vi "SSL Detection Frame Simple Estimator Cameras VelCmd.vi"(0 "Side":enum16{"Esquerdo", "Direito"}(ring)=enum."Direito" caption="Enum", 1 "cameras array":dbl[](array[numeric]), 4 "max ball vel":dbl, 5 "Estimador":T5=enum."Nenhum", 6 "Team":enum16{"Azul", "Amarelo"}(ring) caption="Enum", 8 "Fps":dbl=40.0, 9 "grSim?":bool, 10 "Field Size":T6, 11 "NewCameras":T1[](array[typedef]) {"robots_blue"."height" format="%+4.3f"; "robots_blue"."pixel_y" format="%+4.3f"; "robots_blue"."pixel_x" format="%+4.3f"; "robots_blue"."orientation" format="%+4.3f"; "robots_blue"."y" format="%+4.3f"; "robots_blue"."confidence" format="%4.3f"; "robots_blue"."x" format="%+4.3f"; "robots_yellow"."height" format="%+4.3f"; "robots_yellow"."pixel_y" format="%+4.3f"; "robots_yellow"."pixel_x" format="%+4.3f"; "robots_yellow"."orientation" format="%+4.3f"; "robots_yellow"."y" format="%+4.3f"; "robots_yellow"."confidence" format="%4.3f"; "robots_yellow"."x" format="%+4.3f"}) -> (2 "Field Size Out":T6, 3 "Detection Frame Out":T1 {"robots_blue"."height" format="%+4.3f"; "robots_blue"."pixel_y" format="%+4.3f"; "robots_blue"."pixel_x" format="%+4.3f"; "robots_blue"."orientation" format="%+4.3f"; "robots_blue"."y" format="%+4.3f"; "robots_blue"."confidence" format="%4.3f"; "robots_blue"."x" format="%+4.3f"; "robots_yellow"."height" format="%+4.3f"; "robots_yellow"."pixel_y" format="%+4.3f"; "robots_yellow"."pixel_x" format="%+4.3f"; "robots_yellow"."orientation" format="%+4.3f"; "robots_yellow"."y" format="%+4.3f"; "robots_yellow"."confidence" format="%4.3f"; "robots_yellow"."x" format="%+4.3f"})   [LabVIEW 2020]
uses:
  Controls/SSL Detection Frame.ctl
  Controls/SSL Detection Robot.ctl
  <vilib>/Analysis/Matrix/Datatypes/RealMatrix.ctl
  Controls/SSL Detection Ball.ctl
  Controls/Estimadores.ctl
  <vilib>/Analysis/Matrix/Numeric/Conversions/Array To Matrix - RA.vi
  <vilib>/Analysis/Matrix/NI_Matrix.lvlib
  <vilib>/ptbypt/NI_PtbyPt.lvlib
  Utilities_class/Utilities.lvclass
panel:
  in  "Enable":bool=TRUE
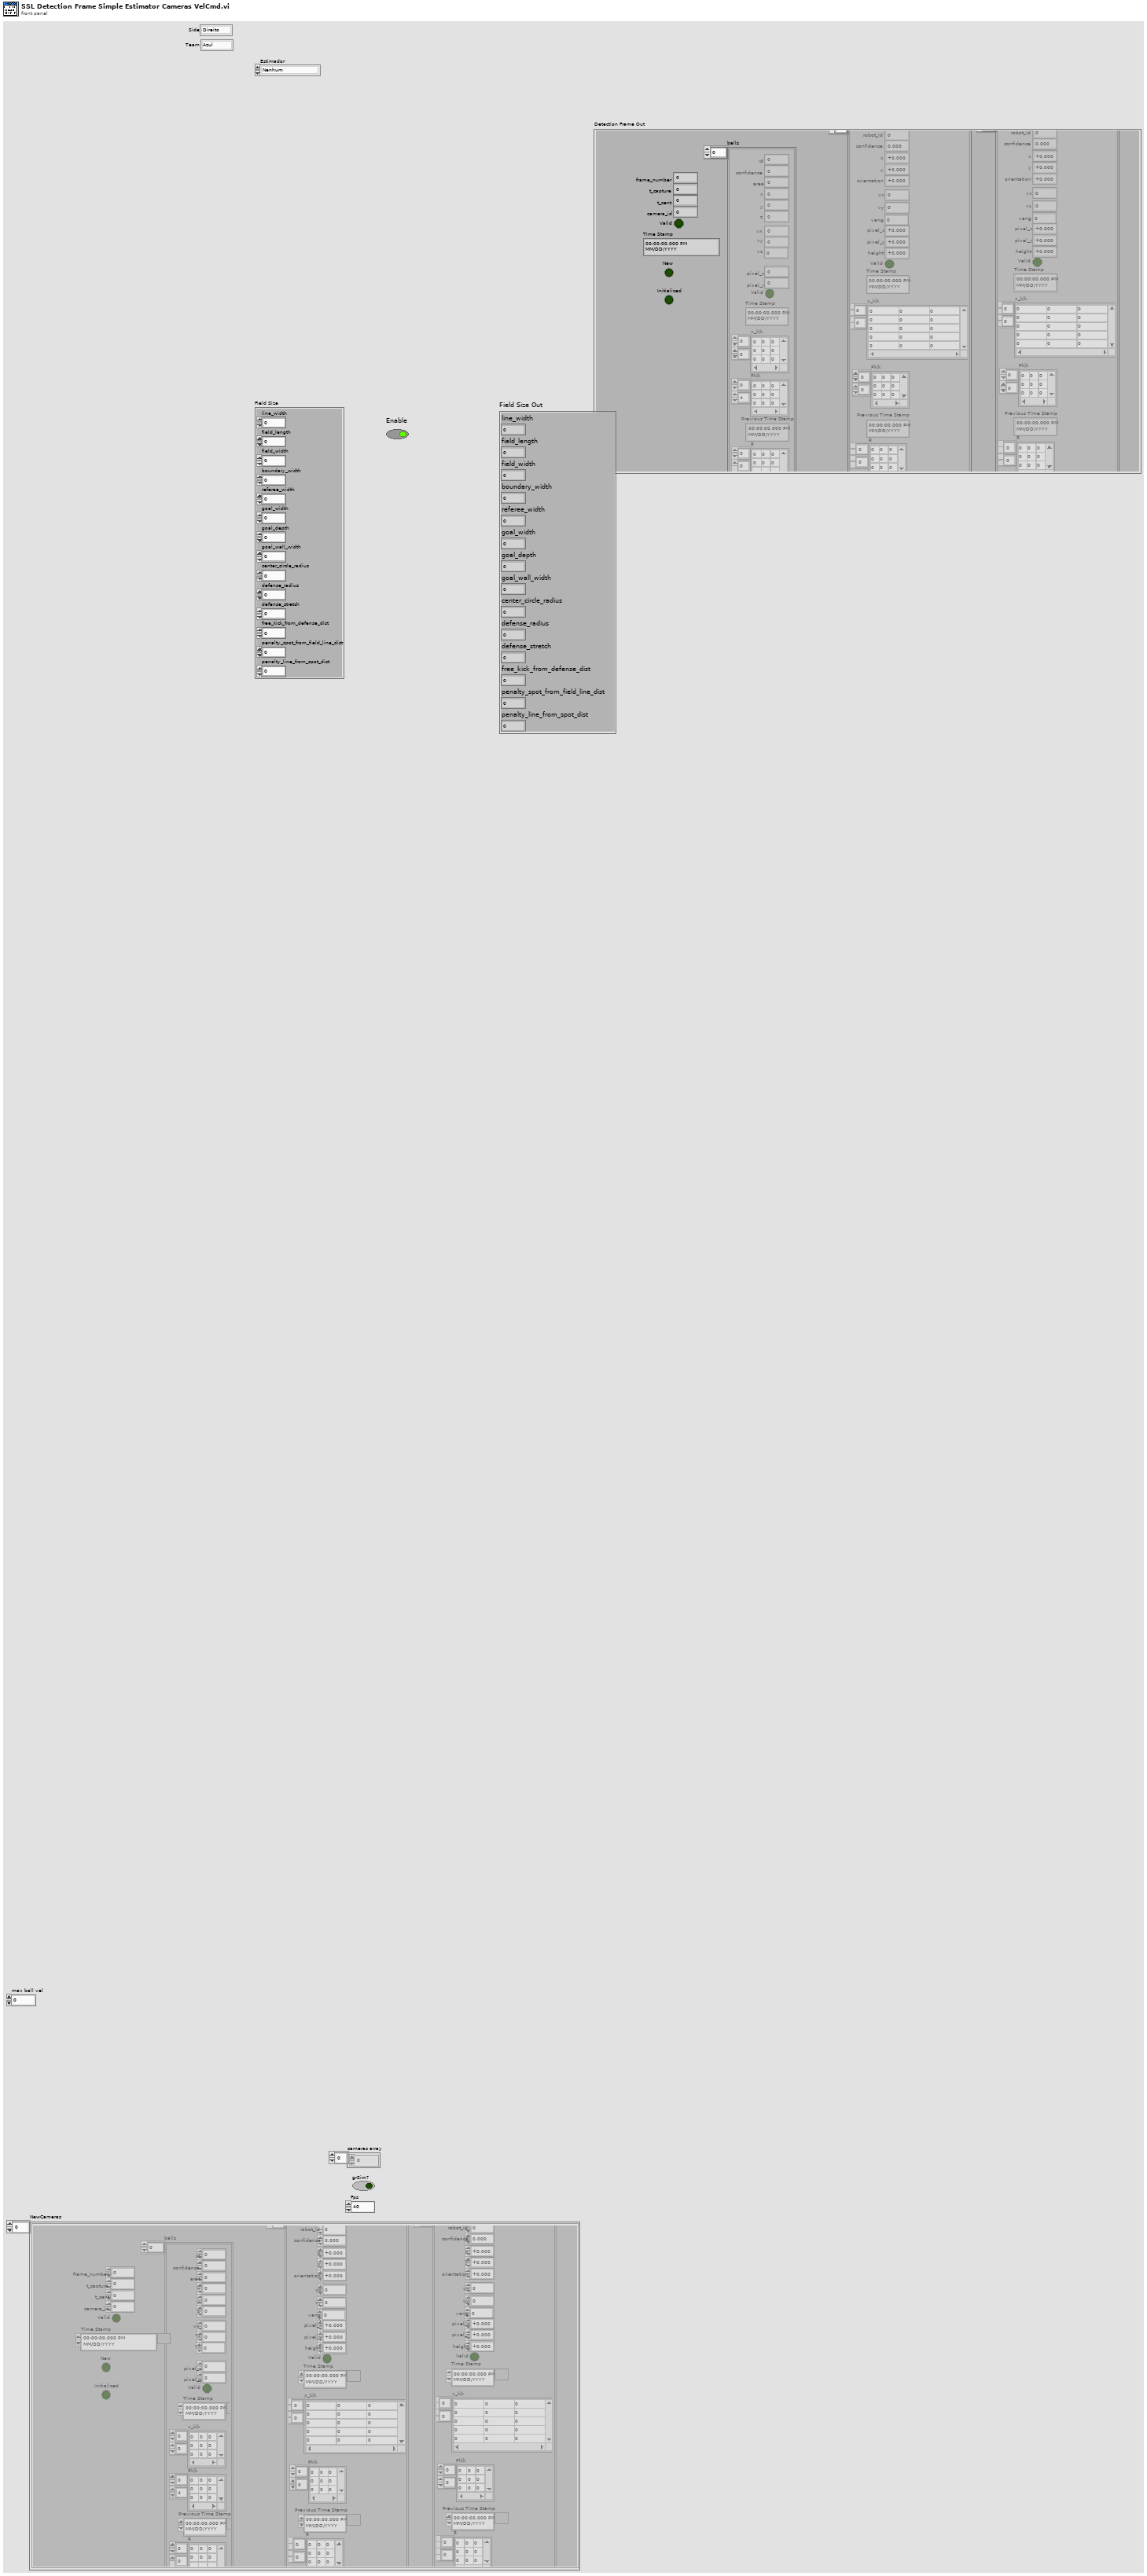
[diagram p1: front panel]
types:
  T1 = typedef "SSL Detection Frame.ctl" = cluster{"frame_number":u32, "t_capture":dbl, "t_sent":dbl, "camera_id":u32, "robots_yellow":T2[], "robots_blue":T2[], "balls":T4[], "Valid":bool, "Time Stamp":timestamp, "New":bool, "Initialized":bool}
  T2 = typedef "SSL Detection Robot.ctl" = cluster{"x":sgl, "robot_id":u32, "confidence":sgl, "y":sgl, "orientation":sgl, "pixel_x":sgl, "pixel_y":sgl, "height":sgl, "Valid":bool, "Time Stamp":timestamp, "x_k|k":T3, "Pk|k":T3, "Previous Time Stamp":timestamp, "R":T3, "vx":dbl, "vy":dbl, "vang":dbl}
  T3 = typedef "NI_Matrix.lvlib/RealMatrix.ctl" = dbl[][]
  T4 = typedef "SSL Detection Ball.ctl" = cluster{"x":sgl, "area":u32, "confidence":sgl, "y":sgl, "z":sgl, "pixel_x":sgl, "pixel_y":sgl, "Valid":bool, "Time Stamp":timestamp, "x_k|k":T3, "Pk|k":T3, "Id":u32, "Previous Time Stamp":timestamp, "R":T3, " vx":sgl, "vy":dbl, "vz":dbl}
  T5 = typedef "Estimadores.ctl" = enum16{"Variable2ndDerivate", "4thDerivate", "2ndDerivate", "Nenhum", "Simples", "Kalman"}
  T6 = cluster{"line_width":u32, "field_length":u32, "field_width":u32, "boundary_width":u32, "referee_width":u32, "goal_width":u32, "goal_depth":u32, "goal_wall_width":u32, "center_circle_radius":u32, "defense_radius":u32, "defense_stretch":u32, "free_kick_from_defense_dist":u32, "penalty_spot_from_field_line_dist":u32, "penalty_line_from_spot_dist":u32}
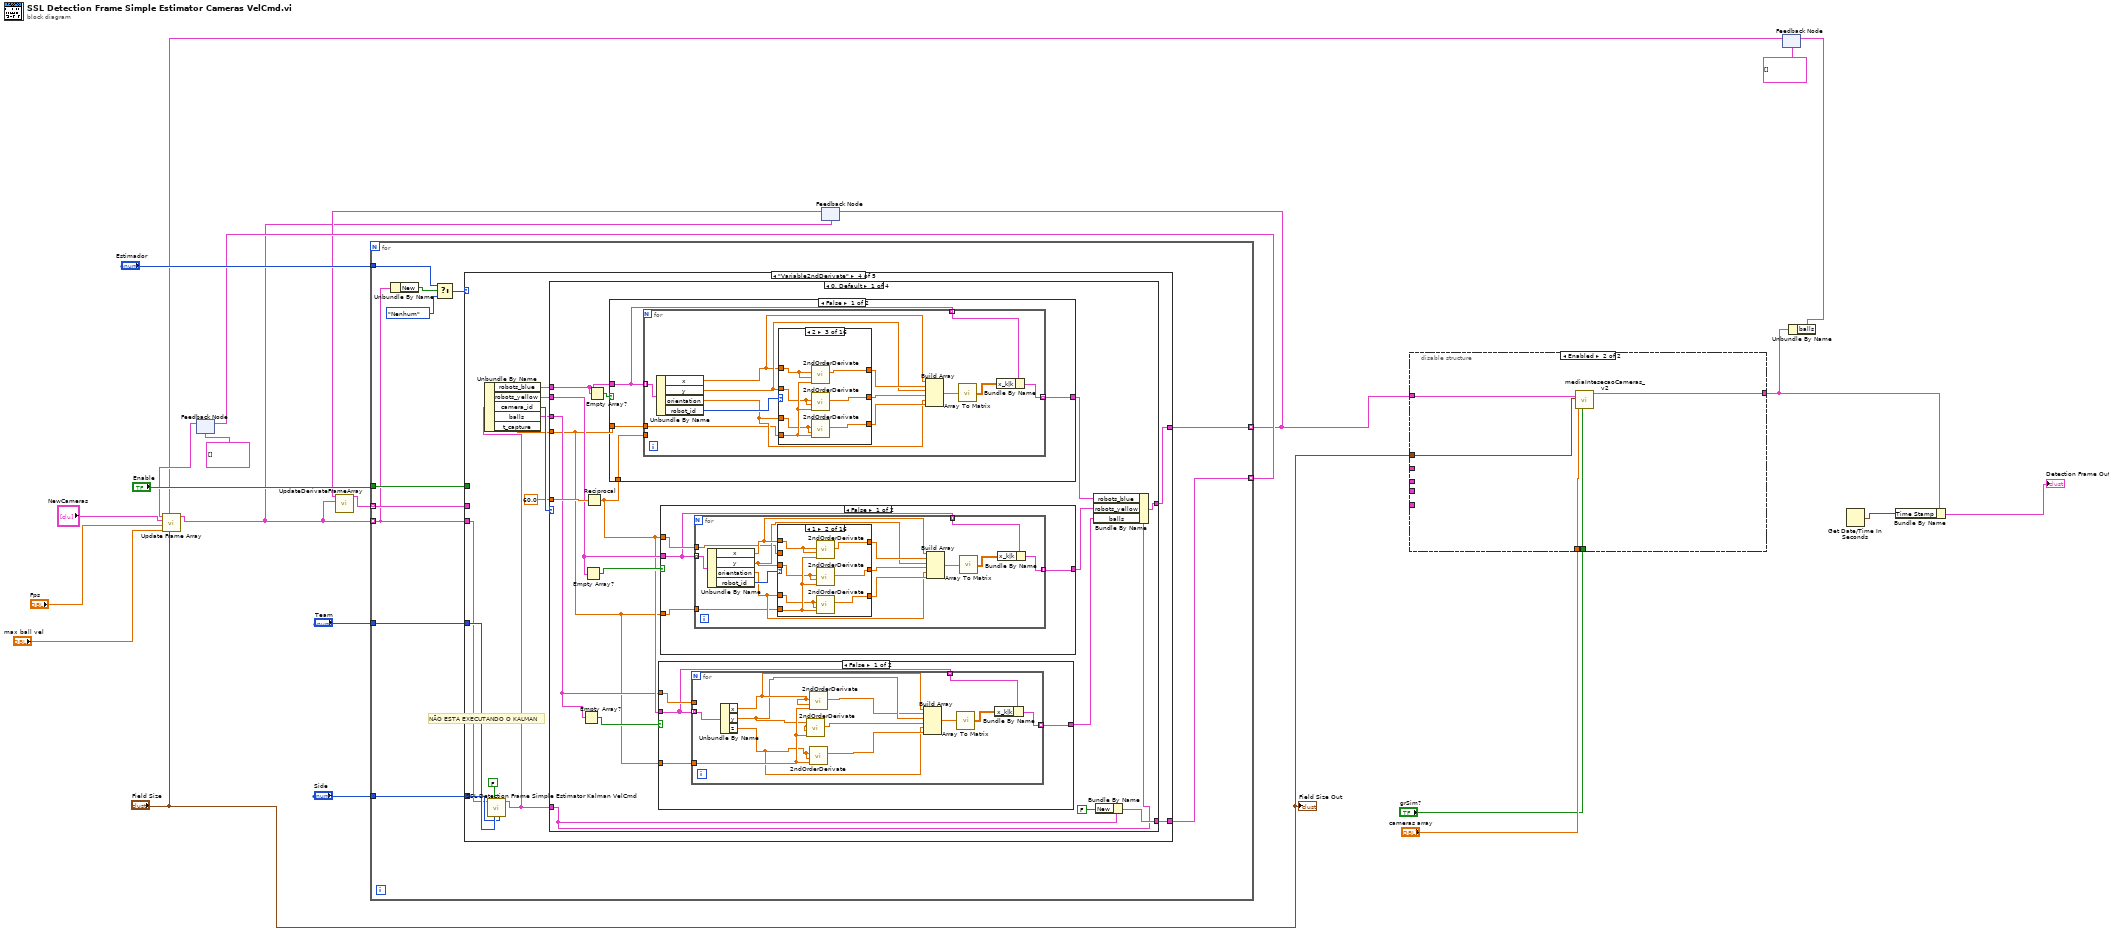
[diagram p0: block diagram]
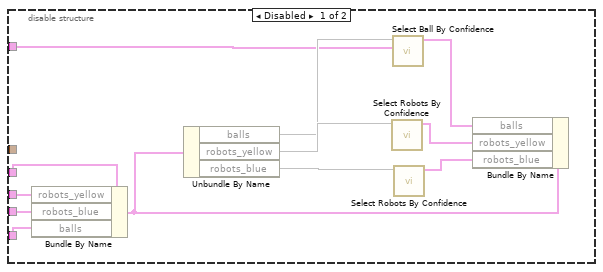
[diagram p2: hidden frame]
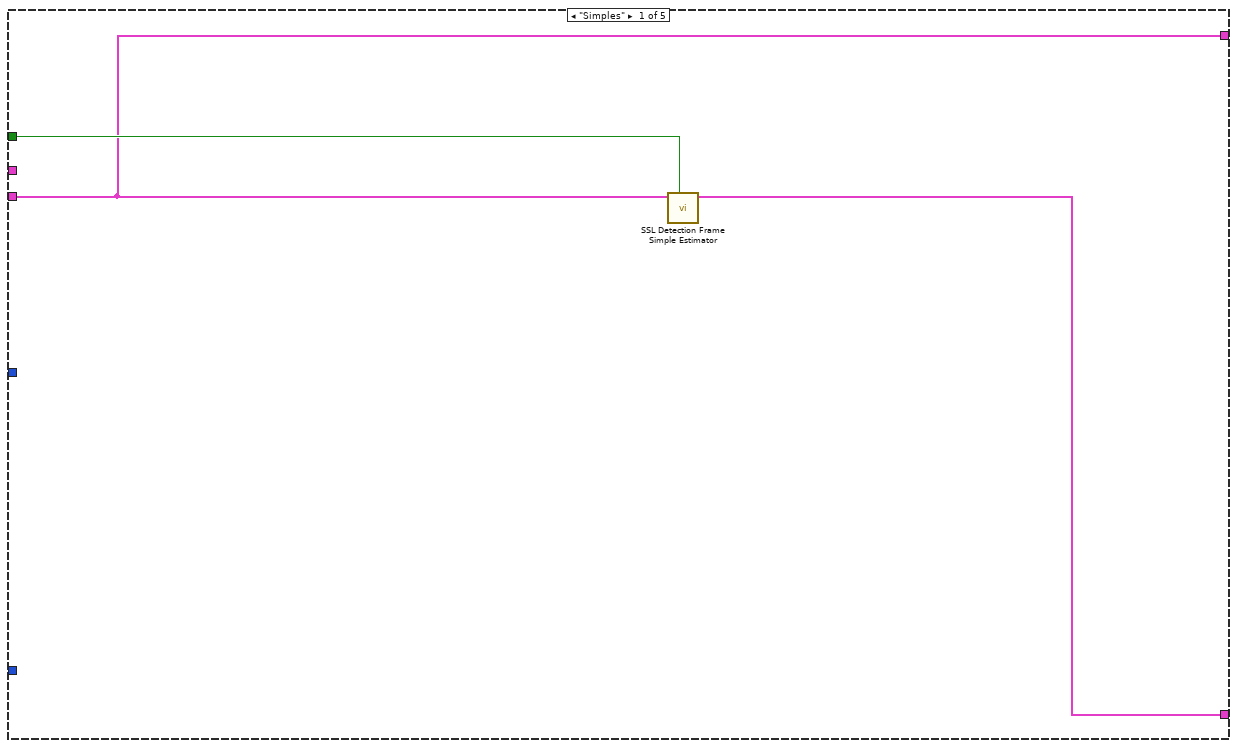
[diagram p3: hidden frame]
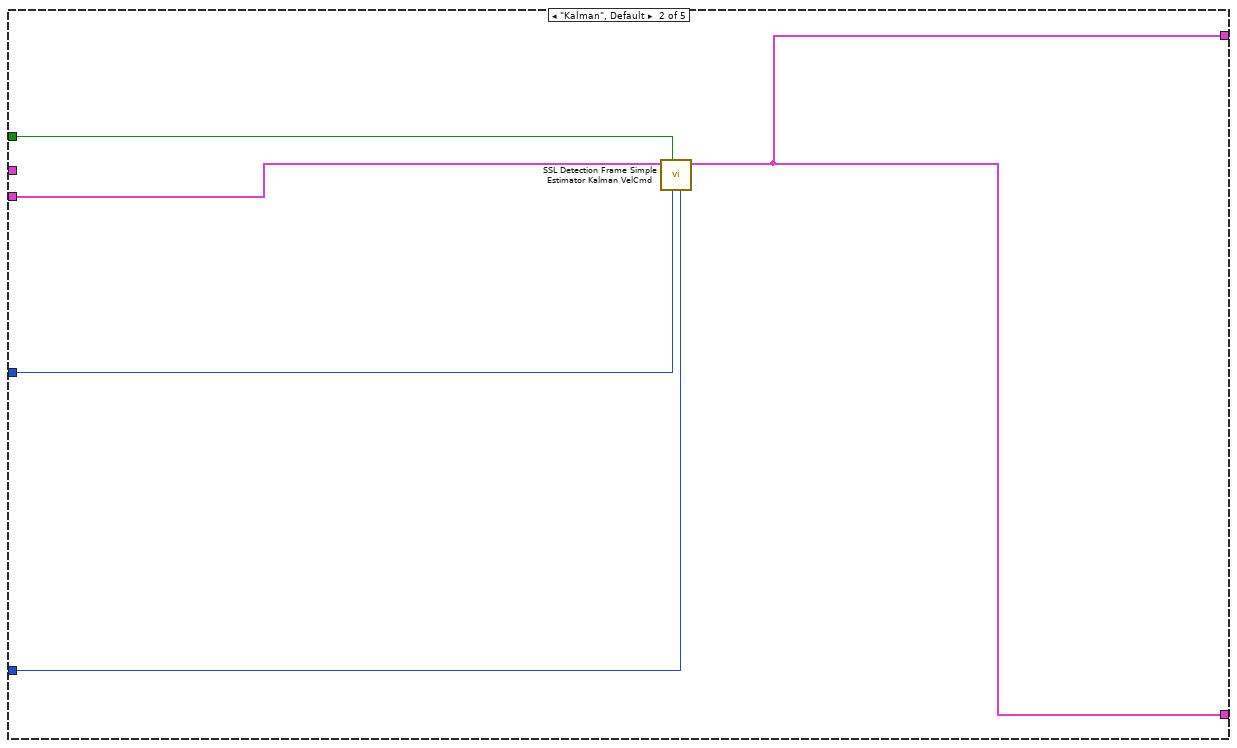
[diagram p4: hidden frame]
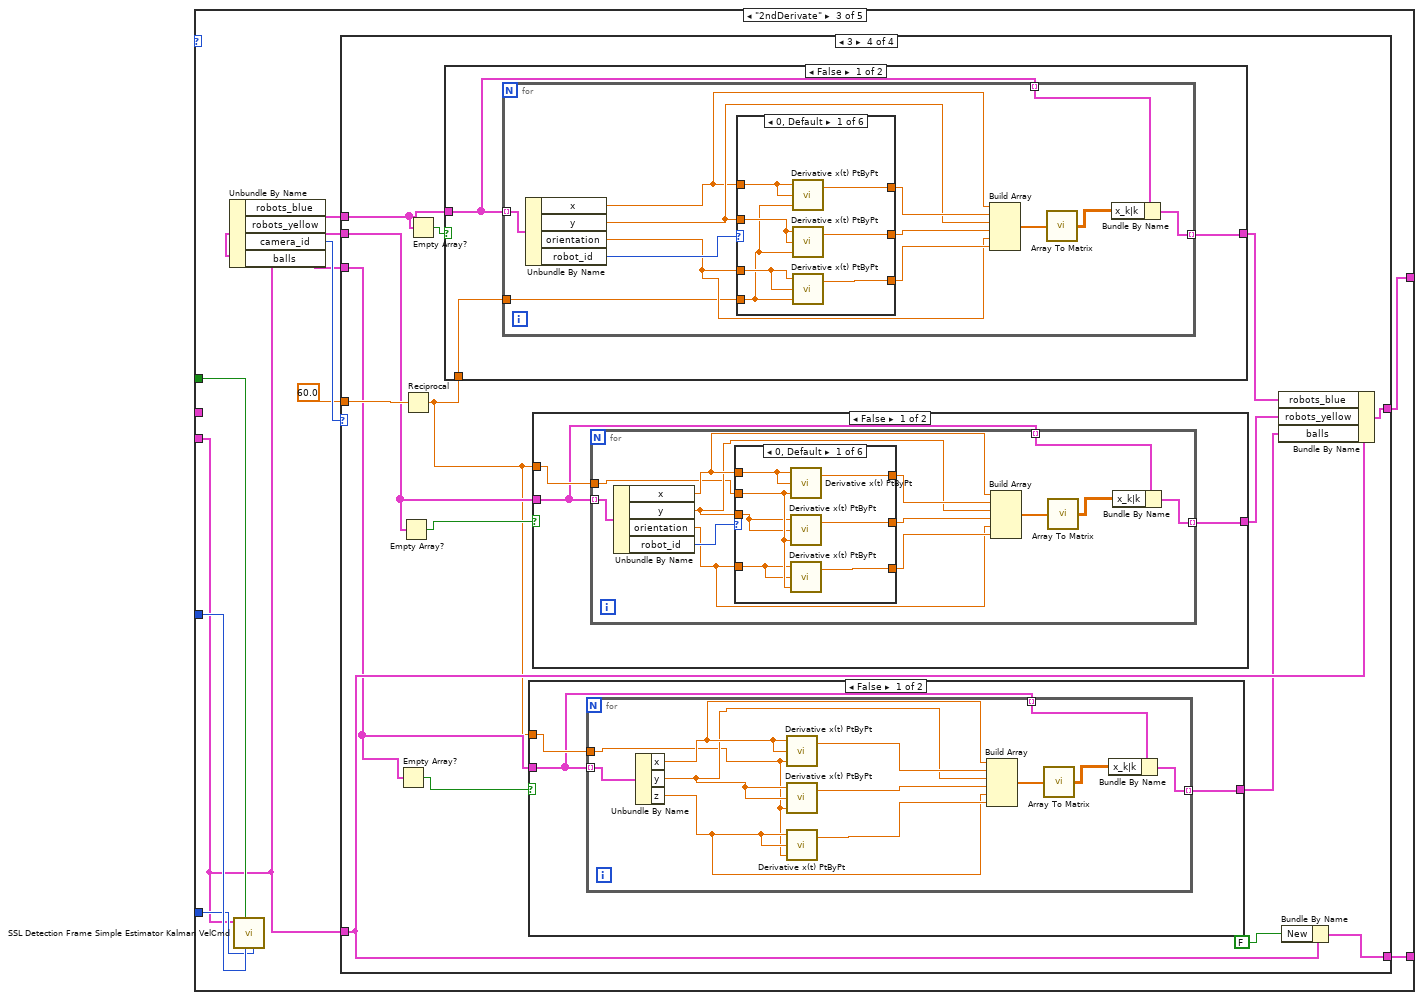
[diagram p5: hidden frame]
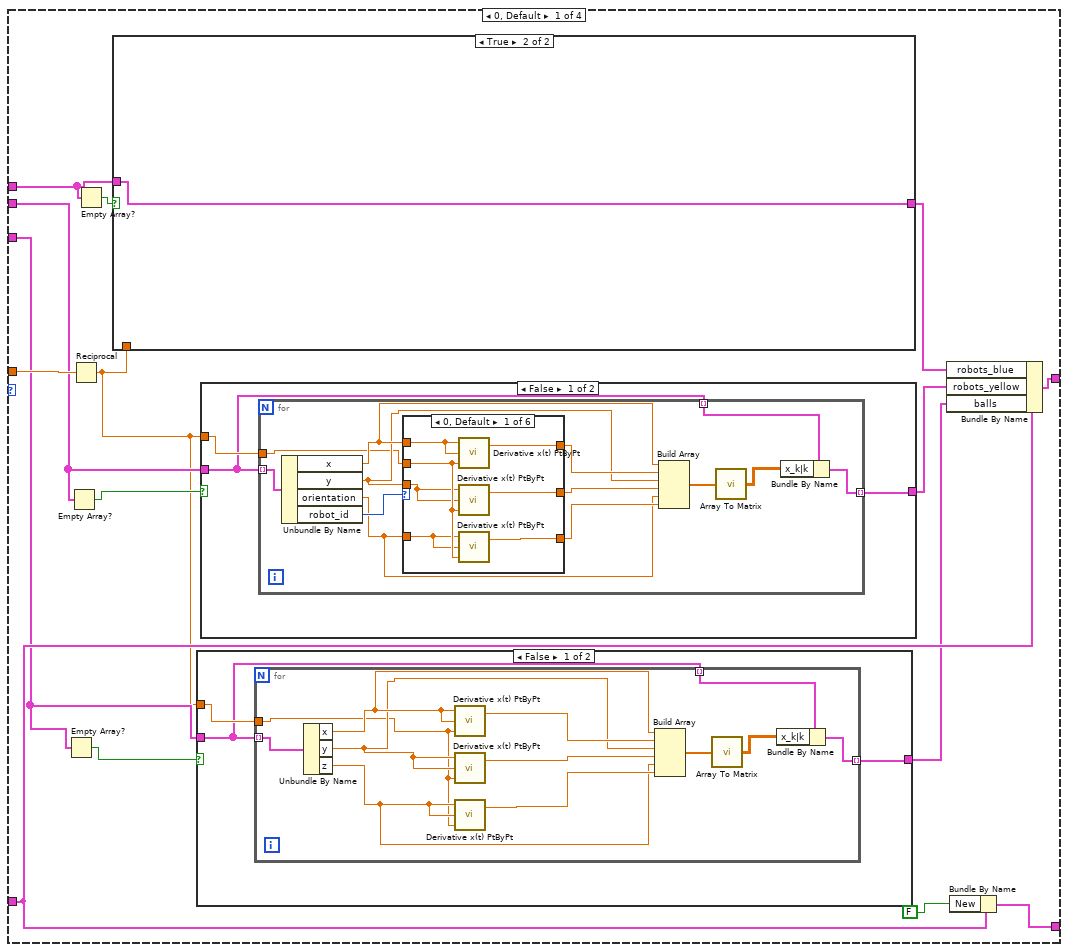
[diagram p6: hidden frame]
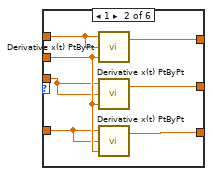
[diagram p8: hidden frame]
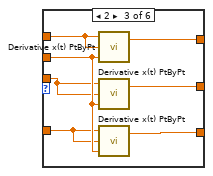
[diagram p9: hidden frame]
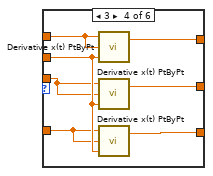
[diagram p10: hidden frame]
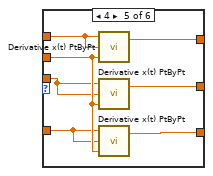
[diagram p11: hidden frame]
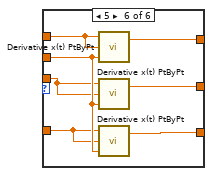
[diagram p12: hidden frame]
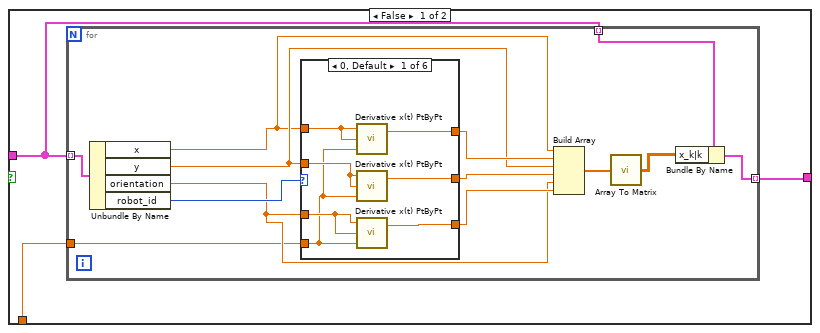
[diagram p14: hidden frame]
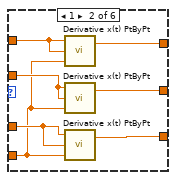
[diagram p15: hidden frame]
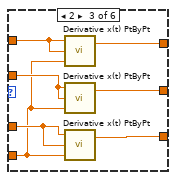
[diagram p16: hidden frame]
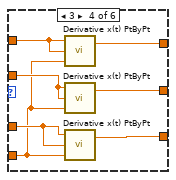
[diagram p17: hidden frame]
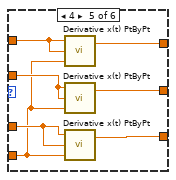
[diagram p18: hidden frame]
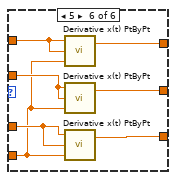
[diagram p19: hidden frame]
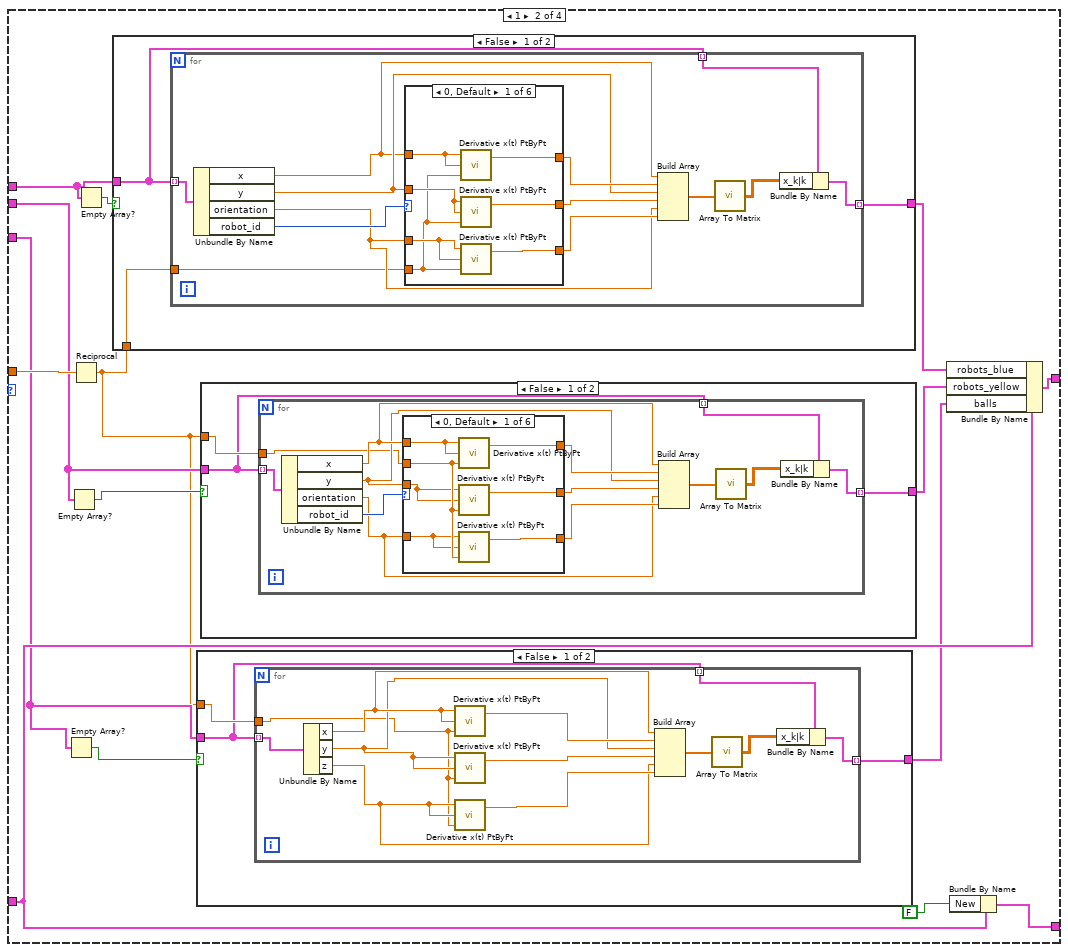
[diagram p20: hidden frame]
diagram:
  n1 = feedback #1(T1[] []) -> (w20:T1[])
  n2 = feedback #2(T4[] [] ("balls")) -> (w14:T4[])
  n3 = call "Update Frame Array.vi"("Field Size"="Field Size", "balls"=w14, "max ball vel"="max ball vel", "Fps"="Fps", "Detection Frame In"="NewCameras", "Array Detection Frame In"=w20) -> ("Detection Frame out"=w6:T1[])  [unwired: 4 in, 1 out]
  n4 = feedback #3(w6) -> (w7:T1[])
  n5 = call "UpdateDerivateFrameArray.vi"("Current Detection Frame In"=w6, "Last Array Detection Frame In"=w7) -> ("Sorted Cameras Array"=w5:T1[])  [unwired: 9 in]
  n6 = for {
    tunnel: [w33] -> w18 mode=indexing
    tunnel: "Estimador" -> [w30]
    tunnel: "Enable" -> [w34]
    tunnel: w6 -> [w25] mode=indexing
    tunnel: "Team" -> [w32]
    tunnel: "Side" -> [w31]
    tunnel: [w28] -> w4 mode=indexing
    tunnel: w5 -> [w27] mode=indexing
    # "NÃO ESTA EXECUTANDO O KALMAN"
    n7 = Unbundle By Name(w25) -> ("New"=w26:bool)
    n8 = Select(t=w30, s=w26, f=Estimadores."Nenhum" ("Estimador")) -> (s? t:f=w29:T5)
    n9 = case shown="\"Variable2ndDerivate\"" w29 {
      tunnel: [w36 w38 w47 w657 w1840] -> w33
      tunnel: w25 -> [w35 w39 w43 w652 w1840]
      tunnel: w34 -> [w37 w42 w53 _ _]
      tunnel: w32 -> [_ w41 w52 w662 _]
      tunnel: w31 -> [_ w40 w51 w661 _]
      tunnel: [w35 w38 w48 w658 w1839] -> w28
      tunnel: w27 -> [_ _ _ _ w1839]
      frame "Simples" {
        n10 = call "SSL Detection Frame Simple Estimator.vi"("Enable"=w37, "Detection Frame In"=w35) -> ("Detection Frame Out"=w36:T1)  [unwired: 8 in, 1 out]
      }
      frame "Kalman", Default {
        n11 = call "SSL Detection Frame Simple Estimator Kalman VelCmd.vi"("Lado"=w40, "Time"=w41, "Enable"=w42, "Detection Frame In"=w39) -> ("Detection Frame Out"=w38:T1)  [unwired: 6 in, 1 out]
      }
      frame "2ndDerivate" {
        n12 = Unbundle By Name(w43) -> ("robots_blue"=w50:T2[], "robots_yellow"=w49:T2[], "camera_id"=w46:u32, "balls"=w45:T4[])
        n13 = call "SSL Detection Frame Simple Estimator Kalman VelCmd.vi"("Lado"=w51, "Time"=w52, "Enable"=w53, "Detection Frame In"=w43) -> ()  [unwired: 6 in, 2 out]
        n14 = case shown="3" w46 {
          tunnel: w50 -> [w67 w216 w365 w514]
          tunnel: 60.0 -> [w66 w215 w364 w513]
          tunnel: w49 -> [w64 w213 w362 w511]
          tunnel: [w61 w210 w359 w508] -> w48
          tunnel: [w59 w208 w357 w506] -> w47
          tunnel: w43 -> [w58 w207 w356 w505]
          tunnel: w45 -> [w56 w205 w354 w503]
          frame 0, Default {
            n15 = Empty Array?(array=w56) -> (empty?=w57:bool)
            n16 = Empty Array?(array=w64) -> (empty?=w65:bool)
            n17 = Reciprocal(x=w66) -> (1/x=w55:dbl)
            n18 = Empty Array?(array=w67) -> (empty?=w68:bool)
            n19 = case shown="True" w68 {
              tunnel: w67 -> [w145 w202]
              tunnel: w55 -> [w146 _]
              tunnel: [w144 w202] -> w63
              frame False {
                n20 = for {
                  tunnel: w145 -> [w159] mode=indexing
                  tunnel: w146 -> [w149]
                  tunnel: w145 -> [w157] mode=indexing
                  tunnel: [w148] -> w144 mode=indexing
                  n21 = Unbundle By Name(w159) -> ("x"=w147:sgl, "y"=w151:sgl, "orientation"=w150:sgl, "robot_id"=w158:u32)
                  n22 = case shown="0, Default" w158 {
                    tunnel: w147 -> [w160 w170 w177 w184 w191 w198]
                    tunnel: [w166 w173 w180 w187 w194 w201] -> w156
                    tunnel: [w165 w172 w179 w186 w193 w200] -> w155
                    tunnel: [w164 w171 w178 w185 w192 w199] -> w154
                    tunnel: w151 -> [w163 w169 w176 w183 w190 w197]
                    tunnel: w150 -> [w162 w168 w175 w182 w189 w196]
                    tunnel: w149 -> [w161 w167 w174 w181 w188 w195]
                    frame 0, Default {
                      n23 = call <vilib>:"Derivative x(t) PtByPt.vi"("dt"=w161, "initial condition"=w160, "x"=w160) -> ("dx/dt"=w166:dbl)  [unwired: 1 in, 1 out]
                      n24 = call <vilib>:"Derivative x(t) PtByPt.vi"("dt"=w161, "initial condition"=w163, "x"=w163) -> ("dx/dt"=w165:dbl)  [unwired: 1 in, 1 out]
                      n25 = call <vilib>:"Derivative x(t) PtByPt.vi"("dt"=w161, "initial condition"=w162, "x"=w162) -> ("dx/dt"=w164:dbl)  [unwired: 1 in, 1 out]
                    }
                    frame 1 {
                      n26 = call <vilib>:"Derivative x(t) PtByPt.vi"("dt"=w167, "initial condition"=w170, "x"=w170) -> ("dx/dt"=w173:dbl)  [unwired: 1 in, 1 out]
                      n27 = call <vilib>:"Derivative x(t) PtByPt.vi"("dt"=w167, "initial condition"=w169, "x"=w169) -> ("dx/dt"=w172:dbl)  [unwired: 1 in, 1 out]
                      n28 = call <vilib>:"Derivative x(t) PtByPt.vi"("dt"=w167, "initial condition"=w168, "x"=w168) -> ("dx/dt"=w171:dbl)  [unwired: 1 in, 1 out]
                    }
                    frame 2 {
                      n29 = call <vilib>:"Derivative x(t) PtByPt.vi"("dt"=w174, "initial condition"=w177, "x"=w177) -> ("dx/dt"=w180:dbl)  [unwired: 1 in, 1 out]
                      n30 = call <vilib>:"Derivative x(t) PtByPt.vi"("dt"=w174, "initial condition"=w176, "x"=w176) -> ("dx/dt"=w179:dbl)  [unwired: 1 in, 1 out]
                      n31 = call <vilib>:"Derivative x(t) PtByPt.vi"("dt"=w174, "initial condition"=w175, "x"=w175) -> ("dx/dt"=w178:dbl)  [unwired: 1 in, 1 out]
                    }
                    frame 3 {
                      n32 = call <vilib>:"Derivative x(t) PtByPt.vi"("dt"=w181, "initial condition"=w184, "x"=w184) -> ("dx/dt"=w187:dbl)  [unwired: 1 in, 1 out]
                      n33 = call <vilib>:"Derivative x(t) PtByPt.vi"("dt"=w181, "initial condition"=w183, "x"=w183) -> ("dx/dt"=w186:dbl)  [unwired: 1 in, 1 out]
                      n34 = call <vilib>:"Derivative x(t) PtByPt.vi"("dt"=w181, "initial condition"=w182, "x"=w182) -> ("dx/dt"=w185:dbl)  [unwired: 1 in, 1 out]
                    }
                    frame 4 {
                      n35 = call <vilib>:"Derivative x(t) PtByPt.vi"("dt"=w188, "initial condition"=w191, "x"=w191) -> ("dx/dt"=w194:dbl)  [unwired: 1 in, 1 out]
                      n36 = call <vilib>:"Derivative x(t) PtByPt.vi"("dt"=w188, "initial condition"=w190, "x"=w190) -> ("dx/dt"=w193:dbl)  [unwired: 1 in, 1 out]
                      n37 = call <vilib>:"Derivative x(t) PtByPt.vi"("dt"=w188, "initial condition"=w189, "x"=w189) -> ("dx/dt"=w192:dbl)  [unwired: 1 in, 1 out]
                    }
                    frame 5 {
                      n38 = call <vilib>:"Derivative x(t) PtByPt.vi"("dt"=w195, "initial condition"=w198, "x"=w198) -> ("dx/dt"=w201:dbl)  [unwired: 1 in, 1 out]
                      n39 = call <vilib>:"Derivative x(t) PtByPt.vi"("dt"=w195, "initial condition"=w197, "x"=w197) -> ("dx/dt"=w200:dbl)  [unwired: 1 in, 1 out]
                      n40 = call <vilib>:"Derivative x(t) PtByPt.vi"("dt"=w195, "initial condition"=w196, "x"=w196) -> ("dx/dt"=w199:dbl)  [unwired: 1 in, 1 out]
                    }
                  }
                  n41 = Build Array(w147, w156, w151, w155, w150, w154) -> (w153:dbl[])
                  n42 = call-poly <vilib>:"Array To Matrix.vi"("Real 1D Array"=w153) -> ("Real Matrix (Column Vector)"=w152:T3)
                  n43 = Bundle By Name(cluster=w157, "x_k|k"=w152) -> (w148:T2)
                }
              }
              frame True {
              }
            }
            n44 = case shown="False" w57 {
              tunnel: w56 -> [w70 w84]
              tunnel: w55 -> [w71 _]
              tunnel: [w69 w84] -> w54
              frame False {
                n45 = for {
                  tunnel: w70 -> [w83] mode=indexing
                  tunnel: w71 -> [w72]
                  tunnel: w70 -> [w82] mode=indexing
                  tunnel: [w73] -> w69 mode=indexing
                  n46 = Unbundle By Name(w83) -> ("x"=w77:sgl, "y"=w76:sgl, "z"=w78:sgl)
                  n47 = call <vilib>:"Derivative x(t) PtByPt.vi"("dt"=w72, "initial condition"=w77, "x"=w77) -> ("dx/dt"=w81:dbl)  [unwired: 1 in, 1 out]
                  n48 = call <vilib>:"Derivative x(t) PtByPt.vi"("dt"=w72, "initial condition"=w76, "x"=w76) -> ("dx/dt"=w80:dbl)  [unwired: 1 in, 1 out]
                  n49 = call <vilib>:"Derivative x(t) PtByPt.vi"("dt"=w72, "initial condition"=w78, "x"=w78) -> ("dx/dt"=w79:dbl)  [unwired: 1 in, 1 out]
                  n50 = Build Array(w77, w81, w76, w80, w78, w79) -> (w75:dbl[])
                  n51 = call-poly <vilib>:"Array To Matrix.vi"("Real 1D Array"=w75) -> ("Real Matrix (Column Vector)"=w74:T3)
                  n52 = Bundle By Name(cluster=w82, "x_k|k"=w74) -> (w73:T4)
                }
              }
              frame True {
              }
            }
            n53 = case shown="False" w65 {
              tunnel: w64 -> [w86 w143]
              tunnel: w55 -> [w87 _]
              tunnel: [w85 w143] -> w62
              frame False {
                n54 = for {
                  tunnel: w86 -> [w100] mode=indexing
                  tunnel: w87 -> [w88]
                  tunnel: w86 -> [w98] mode=indexing
                  tunnel: [w89] -> w85 mode=indexing
                  n55 = Unbundle By Name(w100) -> ("x"=w93:sgl, "y"=w92:sgl, "orientation"=w94:sgl, "robot_id"=w99:u32)
                  n56 = case shown="0, Default" w99 {
                    tunnel: w93 -> [w104 w111 w118 w125 w132 w139]
                    tunnel: w92 -> [w102 w109 w116 w123 w130 w137]
                    tunnel: w94 -> [w101 w108 w115 w122 w129 w136]
                    tunnel: [w107 w114 w121 w128 w135 w142] -> w97
                    tunnel: [w106 w113 w120 w127 w134 w141] -> w96
                    tunnel: [w105 w112 w119 w126 w133 w140] -> w95
                    tunnel: w88 -> [w103 w110 w117 w124 w131 w138]
                    frame 0, Default {
                      n57 = call <vilib>:"Derivative x(t) PtByPt.vi"("dt"=w103, "initial condition"=w104, "x"=w104) -> ("dx/dt"=w107:dbl)  [unwired: 1 in, 1 out]
                      n58 = call <vilib>:"Derivative x(t) PtByPt.vi"("dt"=w103, "initial condition"=w102, "x"=w102) -> ("dx/dt"=w106:dbl)  [unwired: 1 in, 1 out]
                      n59 = call <vilib>:"Derivative x(t) PtByPt.vi"("dt"=w103, "initial condition"=w101, "x"=w101) -> ("dx/dt"=w105:dbl)  [unwired: 1 in, 1 out]
                    }
                    frame 1 {
                      n60 = call <vilib>:"Derivative x(t) PtByPt.vi"("dt"=w110, "initial condition"=w111, "x"=w111) -> ("dx/dt"=w114:dbl)  [unwired: 1 in, 1 out]
                      n61 = call <vilib>:"Derivative x(t) PtByPt.vi"("dt"=w110, "initial condition"=w109, "x"=w109) -> ("dx/dt"=w113:dbl)  [unwired: 1 in, 1 out]
                      n62 = call <vilib>:"Derivative x(t) PtByPt.vi"("dt"=w110, "initial condition"=w108, "x"=w108) -> ("dx/dt"=w112:dbl)  [unwired: 1 in, 1 out]
                    }
                    frame 2 {
                      n63 = call <vilib>:"Derivative x(t) PtByPt.vi"("dt"=w117, "initial condition"=w118, "x"=w118) -> ("dx/dt"=w121:dbl)  [unwired: 1 in, 1 out]
                      n64 = call <vilib>:"Derivative x(t) PtByPt.vi"("dt"=w117, "initial condition"=w116, "x"=w116) -> ("dx/dt"=w120:dbl)  [unwired: 1 in, 1 out]
                      n65 = call <vilib>:"Derivative x(t) PtByPt.vi"("dt"=w117, "initial condition"=w115, "x"=w115) -> ("dx/dt"=w119:dbl)  [unwired: 1 in, 1 out]
                    }
                    frame 3 {
                      n66 = call <vilib>:"Derivative x(t) PtByPt.vi"("dt"=w124, "initial condition"=w125, "x"=w125) -> ("dx/dt"=w128:dbl)  [unwired: 1 in, 1 out]
                      n67 = call <vilib>:"Derivative x(t) PtByPt.vi"("dt"=w124, "initial condition"=w123, "x"=w123) -> ("dx/dt"=w127:dbl)  [unwired: 1 in, 1 out]
                      n68 = call <vilib>:"Derivative x(t) PtByPt.vi"("dt"=w124, "initial condition"=w122, "x"=w122) -> ("dx/dt"=w126:dbl)  [unwired: 1 in, 1 out]
                    }
                    frame 4 {
                      n69 = call <vilib>:"Derivative x(t) PtByPt.vi"("dt"=w131, "initial condition"=w132, "x"=w132) -> ("dx/dt"=w135:dbl)  [unwired: 1 in, 1 out]
                      n70 = call <vilib>:"Derivative x(t) PtByPt.vi"("dt"=w131, "initial condition"=w130, "x"=w130) -> ("dx/dt"=w134:dbl)  [unwired: 1 in, 1 out]
                      n71 = call <vilib>:"Derivative x(t) PtByPt.vi"("dt"=w131, "initial condition"=w129, "x"=w129) -> ("dx/dt"=w133:dbl)  [unwired: 1 in, 1 out]
                    }
                    frame 5 {
                      n72 = call <vilib>:"Derivative x(t) PtByPt.vi"("dt"=w138, "initial condition"=w139, "x"=w139) -> ("dx/dt"=w142:dbl)  [unwired: 1 in, 1 out]
                      n73 = call <vilib>:"Derivative x(t) PtByPt.vi"("dt"=w138, "initial condition"=w137, "x"=w137) -> ("dx/dt"=w141:dbl)  [unwired: 1 in, 1 out]
                      n74 = call <vilib>:"Derivative x(t) PtByPt.vi"("dt"=w138, "initial condition"=w136, "x"=w136) -> ("dx/dt"=w140:dbl)  [unwired: 1 in, 1 out]
                    }
                  }
                  n75 = Build Array(w93, w97, w92, w96, w94, w95) -> (w91:dbl[])
                  n76 = call-poly <vilib>:"Array To Matrix.vi"("Real 1D Array"=w91) -> ("Real Matrix (Column Vector)"=w90:T3)
                  n77 = Bundle By Name(cluster=w98, "x_k|k"=w90) -> (w89:T2)
                }
              }
              frame True {
              }
            }
            n78 = Bundle By Name(cluster=w58, "robots_blue"=w63, "robots_yellow"=w62, "balls"=w54) -> (w61:T1)
            n79 = Bundle By Name(cluster=w58, "New"=FALSE) -> (w59:T1)
          }
          frame 1 {
            n80 = Empty Array?(array=w205) -> (empty?=w206:bool)
            n81 = Empty Array?(array=w213) -> (empty?=w214:bool)
            n82 = Reciprocal(x=w215) -> (1/x=w204:dbl)
            n83 = Empty Array?(array=w216) -> (empty?=w217:bool)
            n84 = case shown="False" w217 {
              tunnel: w216 -> [w294 w351]
              tunnel: w204 -> [w295 _]
              tunnel: [w293 w351] -> w212
              frame False {
                n85 = for {
                  tunnel: w294 -> [w308] mode=indexing
                  tunnel: w295 -> [w298]
                  tunnel: w294 -> [w306] mode=indexing
                  tunnel: [w297] -> w293 mode=indexing
                  n86 = Unbundle By Name(w308) -> ("x"=w296:sgl, "y"=w300:sgl, "orientation"=w299:sgl, "robot_id"=w307:u32)
                  n87 = case shown="0, Default" w307 {
                    tunnel: w296 -> [w309 w319 w326 w333 w340 w347]
                    tunnel: [w315 w322 w329 w336 w343 w350] -> w305
                    tunnel: [w314 w321 w328 w335 w342 w349] -> w304
                    tunnel: [w313 w320 w327 w334 w341 w348] -> w303
                    tunnel: w300 -> [w312 w318 w325 w332 w339 w346]
                    tunnel: w299 -> [w311 w317 w324 w331 w338 w345]
                    tunnel: w298 -> [w310 w316 w323 w330 w337 w344]
                    frame 0, Default {
                      n88 = call <vilib>:"Derivative x(t) PtByPt.vi"("dt"=w310, "initial condition"=w309, "x"=w309) -> ("dx/dt"=w315:dbl)  [unwired: 1 in, 1 out]
                      n89 = call <vilib>:"Derivative x(t) PtByPt.vi"("dt"=w310, "initial condition"=w312, "x"=w312) -> ("dx/dt"=w314:dbl)  [unwired: 1 in, 1 out]
                      n90 = call <vilib>:"Derivative x(t) PtByPt.vi"("dt"=w310, "initial condition"=w311, "x"=w311) -> ("dx/dt"=w313:dbl)  [unwired: 1 in, 1 out]
                    }
                    frame 1 {
                      n91 = call <vilib>:"Derivative x(t) PtByPt.vi"("dt"=w316, "initial condition"=w319, "x"=w319) -> ("dx/dt"=w322:dbl)  [unwired: 1 in, 1 out]
                      n92 = call <vilib>:"Derivative x(t) PtByPt.vi"("dt"=w316, "initial condition"=w318, "x"=w318) -> ("dx/dt"=w321:dbl)  [unwired: 1 in, 1 out]
                      n93 = call <vilib>:"Derivative x(t) PtByPt.vi"("dt"=w316, "initial condition"=w317, "x"=w317) -> ("dx/dt"=w320:dbl)  [unwired: 1 in, 1 out]
                    }
                    frame 2 {
                      n94 = call <vilib>:"Derivative x(t) PtByPt.vi"("dt"=w323, "initial condition"=w326, "x"=w326) -> ("dx/dt"=w329:dbl)  [unwired: 1 in, 1 out]
                      n95 = call <vilib>:"Derivative x(t) PtByPt.vi"("dt"=w323, "initial condition"=w325, "x"=w325) -> ("dx/dt"=w328:dbl)  [unwired: 1 in, 1 out]
                      n96 = call <vilib>:"Derivative x(t) PtByPt.vi"("dt"=w323, "initial condition"=w324, "x"=w324) -> ("dx/dt"=w327:dbl)  [unwired: 1 in, 1 out]
                    }
                    frame 3 {
                      n97 = call <vilib>:"Derivative x(t) PtByPt.vi"("dt"=w330, "initial condition"=w333, "x"=w333) -> ("dx/dt"=w336:dbl)  [unwired: 1 in, 1 out]
                      n98 = call <vilib>:"Derivative x(t) PtByPt.vi"("dt"=w330, "initial condition"=w332, "x"=w332) -> ("dx/dt"=w335:dbl)  [unwired: 1 in, 1 out]
                      n99 = call <vilib>:"Derivative x(t) PtByPt.vi"("dt"=w330, "initial condition"=w331, "x"=w331) -> ("dx/dt"=w334:dbl)  [unwired: 1 in, 1 out]
                    }
                    frame 4 {
                      n100 = call <vilib>:"Derivative x(t) PtByPt.vi"("dt"=w337, "initial condition"=w340, "x"=w340) -> ("dx/dt"=w343:dbl)  [unwired: 1 in, 1 out]
                      n101 = call <vilib>:"Derivative x(t) PtByPt.vi"("dt"=w337, "initial condition"=w339, "x"=w339) -> ("dx/dt"=w342:dbl)  [unwired: 1 in, 1 out]
                      n102 = call <vilib>:"Derivative x(t) PtByPt.vi"("dt"=w337, "initial condition"=w338, "x"=w338) -> ("dx/dt"=w341:dbl)  [unwired: 1 in, 1 out]
                    }
                    frame 5 {
                      n103 = call <vilib>:"Derivative x(t) PtByPt.vi"("dt"=w344, "initial condition"=w347, "x"=w347) -> ("dx/dt"=w350:dbl)  [unwired: 1 in, 1 out]
                      n104 = call <vilib>:"Derivative x(t) PtByPt.vi"("dt"=w344, "initial condition"=w346, "x"=w346) -> ("dx/dt"=w349:dbl)  [unwired: 1 in, 1 out]
                      n105 = call <vilib>:"Derivative x(t) PtByPt.vi"("dt"=w344, "initial condition"=w345, "x"=w345) -> ("dx/dt"=w348:dbl)  [unwired: 1 in, 1 out]
                    }
                  }
                  n106 = Build Array(w296, w305, w300, w304, w299, w303) -> (w302:dbl[])
                  n107 = call-poly <vilib>:"Array To Matrix.vi"("Real 1D Array"=w302) -> ("Real Matrix (Column Vector)"=w301:T3)
                  n108 = Bundle By Name(cluster=w306, "x_k|k"=w301) -> (w297:T2)
                }
              }
              frame True {
              }
            }
            n109 = case shown="False" w206 {
              tunnel: w205 -> [w219 w233]
              tunnel: w204 -> [w220 _]
              tunnel: [w218 w233] -> w203
              frame False {
                n110 = for {
                  tunnel: w219 -> [w232] mode=indexing
                  tunnel: w220 -> [w221]
                  tunnel: w219 -> [w231] mode=indexing
                  tunnel: [w222] -> w218 mode=indexing
                  n111 = Unbundle By Name(w232) -> ("x"=w226:sgl, "y"=w225:sgl, "z"=w227:sgl)
                  n112 = call <vilib>:"Derivative x(t) PtByPt.vi"("dt"=w221, "initial condition"=w226, "x"=w226) -> ("dx/dt"=w230:dbl)  [unwired: 1 in, 1 out]
                  n113 = call <vilib>:"Derivative x(t) PtByPt.vi"("dt"=w221, "initial condition"=w225, "x"=w225) -> ("dx/dt"=w229:dbl)  [unwired: 1 in, 1 out]
                  n114 = call <vilib>:"Derivative x(t) PtByPt.vi"("dt"=w221, "initial condition"=w227, "x"=w227) -> ("dx/dt"=w228:dbl)  [unwired: 1 in, 1 out]
                  n115 = Build Array(w226, w230, w225, w229, w227, w228) -> (w224:dbl[])
                  n116 = call-poly <vilib>:"Array To Matrix.vi"("Real 1D Array"=w224) -> ("Real Matrix (Column Vector)"=w223:T3)
                  n117 = Bundle By Name(cluster=w231, "x_k|k"=w223) -> (w222:T4)
                }
              }
              frame True {
              }
            }
            n118 = case shown="False" w214 {
              tunnel: w213 -> [w235 w292]
              tunnel: w204 -> [w236 _]
              tunnel: [w234 w292] -> w211
              frame False {
                n119 = for {
                  tunnel: w235 -> [w249] mode=indexing
                  tunnel: w236 -> [w237]
                  tunnel: w235 -> [w247] mode=indexing
                  tunnel: [w238] -> w234 mode=indexing
                  n120 = Unbundle By Name(w249) -> ("x"=w242:sgl, "y"=w241:sgl, "orientation"=w243:sgl, "robot_id"=w248:u32)
                  n121 = case shown="0, Default" w248 {
                    tunnel: w242 -> [w253 w260 w267 w274 w281 w288]
                    tunnel: w241 -> [w251 w258 w265 w272 w279 w286]
                    tunnel: w243 -> [w250 w257 w264 w271 w278 w285]
                    tunnel: [w256 w263 w270 w277 w284 w291] -> w246
                    tunnel: [w255 w262 w269 w276 w283 w290] -> w245
                    tunnel: [w254 w261 w268 w275 w282 w289] -> w244
                    tunnel: w237 -> [w252 w259 w266 w273 w280 w287]
                    frame 0, Default {
                      n122 = call <vilib>:"Derivative x(t) PtByPt.vi"("dt"=w252, "initial condition"=w253, "x"=w253) -> ("dx/dt"=w256:dbl)  [unwired: 1 in, 1 out]
                      n123 = call <vilib>:"Derivative x(t) PtByPt.vi"("dt"=w252, "initial condition"=w251, "x"=w251) -> ("dx/dt"=w255:dbl)  [unwired: 1 in, 1 out]
                      n124 = call <vilib>:"Derivative x(t) PtByPt.vi"("dt"=w252, "initial condition"=w250, "x"=w250) -> ("dx/dt"=w254:dbl)  [unwired: 1 in, 1 out]
                    }
                    frame 1 {
                      n125 = call <vilib>:"Derivative x(t) PtByPt.vi"("dt"=w259, "initial condition"=w260, "x"=w260) -> ("dx/dt"=w263:dbl)  [unwired: 1 in, 1 out]
                      n126 = call <vilib>:"Derivative x(t) PtByPt.vi"("dt"=w259, "initial condition"=w258, "x"=w258) -> ("dx/dt"=w262:dbl)  [unwired: 1 in, 1 out]
                      n127 = call <vilib>:"Derivative x(t) PtByPt.vi"("dt"=w259, "initial condition"=w257, "x"=w257) -> ("dx/dt"=w261:dbl)  [unwired: 1 in, 1 out]
                    }
                    frame 2 {
                      n128 = call <vilib>:"Derivative x(t) PtByPt.vi"("dt"=w266, "initial condition"=w267, "x"=w267) -> ("dx/dt"=w270:dbl)  [unwired: 1 in, 1 out]
                      n129 = call <vilib>:"Derivative x(t) PtByPt.vi"("dt"=w266, "initial condition"=w265, "x"=w265) -> ("dx/dt"=w269:dbl)  [unwired: 1 in, 1 out]
                      n130 = call <vilib>:"Derivative x(t) PtByPt.vi"("dt"=w266, "initial condition"=w264, "x"=w264) -> ("dx/dt"=w268:dbl)  [unwired: 1 in, 1 out]
                    }
                    frame 3 {
                      n131 = call <vilib>:"Derivative x(t) PtByPt.vi"("dt"=w273, "initial condition"=w274, "x"=w274) -> ("dx/dt"=w277:dbl)  [unwired: 1 in, 1 out]
                      n132 = call <vilib>:"Derivative x(t) PtByPt.vi"("dt"=w273, "initial condition"=w272, "x"=w272) -> ("dx/dt"=w276:dbl)  [unwired: 1 in, 1 out]
                      n133 = call <vilib>:"Derivative x(t) PtByPt.vi"("dt"=w273, "initial condition"=w271, "x"=w271) -> ("dx/dt"=w275:dbl)  [unwired: 1 in, 1 out]
                    }
                    frame 4 {
                      n134 = call <vilib>:"Derivative x(t) PtByPt.vi"("dt"=w280, "initial condition"=w281, "x"=w281) -> ("dx/dt"=w284:dbl)  [unwired: 1 in, 1 out]
                      n135 = call <vilib>:"Derivative x(t) PtByPt.vi"("dt"=w280, "initial condition"=w279, "x"=w279) -> ("dx/dt"=w283:dbl)  [unwired: 1 in, 1 out]
                      n136 = call <vilib>:"Derivative x(t) PtByPt.vi"("dt"=w280, "initial condition"=w278, "x"=w278) -> ("dx/dt"=w282:dbl)  [unwired: 1 in, 1 out]
                    }
                    frame 5 {
                      n137 = call <vilib>:"Derivative x(t) PtByPt.vi"("dt"=w287, "initial condition"=w288, "x"=w288) -> ("dx/dt"=w291:dbl)  [unwired: 1 in, 1 out]
                      n138 = call <vilib>:"Derivative x(t) PtByPt.vi"("dt"=w287, "initial condition"=w286, "x"=w286) -> ("dx/dt"=w290:dbl)  [unwired: 1 in, 1 out]
                      n139 = call <vilib>:"Derivative x(t) PtByPt.vi"("dt"=w287, "initial condition"=w285, "x"=w285) -> ("dx/dt"=w289:dbl)  [unwired: 1 in, 1 out]
                    }
                  }
                  n140 = Build Array(w242, w246, w241, w245, w243, w244) -> (w240:dbl[])
                  n141 = call-poly <vilib>:"Array To Matrix.vi"("Real 1D Array"=w240) -> ("Real Matrix (Column Vector)"=w239:T3)
                  n142 = Bundle By Name(cluster=w247, "x_k|k"=w239) -> (w238:T2)
                }
              }
              frame True {
              }
            }
            n143 = Bundle By Name(cluster=w207, "robots_blue"=w212, "robots_yellow"=w211, "balls"=w203) -> (w210:T1)
            n144 = Bundle By Name(cluster=w207, "New"=FALSE) -> (w208:T1)
          }
          frame 2 {
            n145 = Empty Array?(array=w354) -> (empty?=w355:bool)
            n146 = Empty Array?(array=w362) -> (empty?=w363:bool)
            n147 = Reciprocal(x=w364) -> (1/x=w353:dbl)
            n148 = Empty Array?(array=w365) -> (empty?=w366:bool)
            n149 = case shown="False" w366 {
              tunnel: w365 -> [w443 w500]
              tunnel: w353 -> [w444 _]
              tunnel: [w442 w500] -> w361
              frame False {
                n150 = for {
                  tunnel: w443 -> [w457] mode=indexing
                  tunnel: w444 -> [w447]
                  tunnel: w443 -> [w455] mode=indexing
                  tunnel: [w446] -> w442 mode=indexing
                  n151 = Unbundle By Name(w457) -> ("x"=w445:sgl, "y"=w449:sgl, "orientation"=w448:sgl, "robot_id"=w456:u32)
                  n152 = case shown="0, Default" w456 {
                    tunnel: w445 -> [w458 w468 w475 w482 w489 w496]
                    tunnel: [w464 w471 w478 w485 w492 w499] -> w454
                    tunnel: [w463 w470 w477 w484 w491 w498] -> w453
                    tunnel: [w462 w469 w476 w483 w490 w497] -> w452
                    tunnel: w449 -> [w461 w467 w474 w481 w488 w495]
                    tunnel: w448 -> [w460 w466 w473 w480 w487 w494]
                    tunnel: w447 -> [w459 w465 w472 w479 w486 w493]
                    frame 0, Default {
                      n153 = call <vilib>:"Derivative x(t) PtByPt.vi"("dt"=w459, "initial condition"=w458, "x"=w458) -> ("dx/dt"=w464:dbl)  [unwired: 1 in, 1 out]
                      n154 = call <vilib>:"Derivative x(t) PtByPt.vi"("dt"=w459, "initial condition"=w461, "x"=w461) -> ("dx/dt"=w463:dbl)  [unwired: 1 in, 1 out]
                      n155 = call <vilib>:"Derivative x(t) PtByPt.vi"("dt"=w459, "initial condition"=w460, "x"=w460) -> ("dx/dt"=w462:dbl)  [unwired: 1 in, 1 out]
                    }
                    frame 1 {
                      n156 = call <vilib>:"Derivative x(t) PtByPt.vi"("dt"=w465, "initial condition"=w468, "x"=w468) -> ("dx/dt"=w471:dbl)  [unwired: 1 in, 1 out]
                      n157 = call <vilib>:"Derivative x(t) PtByPt.vi"("dt"=w465, "initial condition"=w467, "x"=w467) -> ("dx/dt"=w470:dbl)  [unwired: 1 in, 1 out]
                      n158 = call <vilib>:"Derivative x(t) PtByPt.vi"("dt"=w465, "initial condition"=w466, "x"=w466) -> ("dx/dt"=w469:dbl)  [unwired: 1 in, 1 out]
                    }
                    frame 2 {
                      n159 = call <vilib>:"Derivative x(t) PtByPt.vi"("dt"=w472, "initial condition"=w475, "x"=w475) -> ("dx/dt"=w478:dbl)  [unwired: 1 in, 1 out]
                      n160 = call <vilib>:"Derivative x(t) PtByPt.vi"("dt"=w472, "initial condition"=w474, "x"=w474) -> ("dx/dt"=w477:dbl)  [unwired: 1 in, 1 out]
                      n161 = call <vilib>:"Derivative x(t) PtByPt.vi"("dt"=w472, "initial condition"=w473, "x"=w473) -> ("dx/dt"=w476:dbl)  [unwired: 1 in, 1 out]
                    }
                    frame 3 {
                      n162 = call <vilib>:"Derivative x(t) PtByPt.vi"("dt"=w479, "initial condition"=w482, "x"=w482) -> ("dx/dt"=w485:dbl)  [unwired: 1 in, 1 out]
                      n163 = call <vilib>:"Derivative x(t) PtByPt.vi"("dt"=w479, "initial condition"=w481, "x"=w481) -> ("dx/dt"=w484:dbl)  [unwired: 1 in, 1 out]
                      n164 = call <vilib>:"Derivative x(t) PtByPt.vi"("dt"=w479, "initial condition"=w480, "x"=w480) -> ("dx/dt"=w483:dbl)  [unwired: 1 in, 1 out]
                    }
                    frame 4 {
                      n165 = call <vilib>:"Derivative x(t) PtByPt.vi"("dt"=w486, "initial condition"=w489, "x"=w489) -> ("dx/dt"=w492:dbl)  [unwired: 1 in, 1 out]
                      n166 = call <vilib>:"Derivative x(t) PtByPt.vi"("dt"=w486, "initial condition"=w488, "x"=w488) -> ("dx/dt"=w491:dbl)  [unwired: 1 in, 1 out]
                      n167 = call <vilib>:"Derivative x(t) PtByPt.vi"("dt"=w486, "initial condition"=w487, "x"=w487) -> ("dx/dt"=w490:dbl)  [unwired: 1 in, 1 out]
                    }
                    frame 5 {
                      n168 = call <vilib>:"Derivative x(t) PtByPt.vi"("dt"=w493, "initial condition"=w496, "x"=w496) -> ("dx/dt"=w499:dbl)  [unwired: 1 in, 1 out]
                      n169 = call <vilib>:"Derivative x(t) PtByPt.vi"("dt"=w493, "initial condition"=w495, "x"=w495) -> ("dx/dt"=w498:dbl)  [unwired: 1 in, 1 out]
                      n170 = call <vilib>:"Derivative x(t) PtByPt.vi"("dt"=w493, "initial condition"=w494, "x"=w494) -> ("dx/dt"=w497:dbl)  [unwired: 1 in, 1 out]
                    }
                  }
                  n171 = Build Array(w445, w454, w449, w453, w448, w452) -> (w451:dbl[])
                  n172 = call-poly <vilib>:"Array To Matrix.vi"("Real 1D Array"=w451) -> ("Real Matrix (Column Vector)"=w450:T3)
                  n173 = Bundle By Name(cluster=w455, "x_k|k"=w450) -> (w446:T2)
                }
              }
              frame True {
              }
            }
            n174 = case shown="False" w355 {
              tunnel: w354 -> [w368 w382]
              tunnel: w353 -> [w369 _]
              tunnel: [w367 w382] -> w352
              frame False {
                n175 = for {
                  tunnel: w368 -> [w381] mode=indexing
                  tunnel: w369 -> [w370]
                  tunnel: w368 -> [w380] mode=indexing
                  tunnel: [w371] -> w367 mode=indexing
                  n176 = Unbundle By Name(w381) -> ("x"=w375:sgl, "y"=w374:sgl, "z"=w376:sgl)
                  n177 = call <vilib>:"Derivative x(t) PtByPt.vi"("dt"=w370, "initial condition"=w375, "x"=w375) -> ("dx/dt"=w379:dbl)  [unwired: 1 in, 1 out]
                  n178 = call <vilib>:"Derivative x(t) PtByPt.vi"("dt"=w370, "initial condition"=w374, "x"=w374) -> ("dx/dt"=w378:dbl)  [unwired: 1 in, 1 out]
                  n179 = call <vilib>:"Derivative x(t) PtByPt.vi"("dt"=w370, "initial condition"=w376, "x"=w376) -> ("dx/dt"=w377:dbl)  [unwired: 1 in, 1 out]
                  n180 = Build Array(w375, w379, w374, w378, w376, w377) -> (w373:dbl[])
                  n181 = call-poly <vilib>:"Array To Matrix.vi"("Real 1D Array"=w373) -> ("Real Matrix (Column Vector)"=w372:T3)
                  n182 = Bundle By Name(cluster=w380, "x_k|k"=w372) -> (w371:T4)
                }
              }
              frame True {
              }
            }
            n183 = case shown="False" w363 {
              tunnel: w362 -> [w384 w441]
              tunnel: w353 -> [w385 _]
              tunnel: [w383 w441] -> w360
              frame False {
                n184 = for {
                  tunnel: w384 -> [w398] mode=indexing
                  tunnel: w385 -> [w386]
                  tunnel: w384 -> [w396] mode=indexing
                  tunnel: [w387] -> w383 mode=indexing
                  n185 = Unbundle By Name(w398) -> ("x"=w391:sgl, "y"=w390:sgl, "orientation"=w392:sgl, "robot_id"=w397:u32)
                  n186 = case shown="0, Default" w397 {
                    tunnel: w391 -> [w402 w409 w416 w423 w430 w437]
                    tunnel: w390 -> [w400 w407 w414 w421 w428 w435]
                    tunnel: w392 -> [w399 w406 w413 w420 w427 w434]
                    tunnel: [w405 w412 w419 w426 w433 w440] -> w395
                    tunnel: [w404 w411 w418 w425 w432 w439] -> w394
                    tunnel: [w403 w410 w417 w424 w431 w438] -> w393
                    tunnel: w386 -> [w401 w408 w415 w422 w429 w436]
                    frame 0, Default {
                      n187 = call <vilib>:"Derivative x(t) PtByPt.vi"("dt"=w401, "initial condition"=w402, "x"=w402) -> ("dx/dt"=w405:dbl)  [unwired: 1 in, 1 out]
                      n188 = call <vilib>:"Derivative x(t) PtByPt.vi"("dt"=w401, "initial condition"=w400, "x"=w400) -> ("dx/dt"=w404:dbl)  [unwired: 1 in, 1 out]
                      n189 = call <vilib>:"Derivative x(t) PtByPt.vi"("dt"=w401, "initial condition"=w399, "x"=w399) -> ("dx/dt"=w403:dbl)  [unwired: 1 in, 1 out]
                    }
                    frame 1 {
                      n190 = call <vilib>:"Derivative x(t) PtByPt.vi"("dt"=w408, "initial condition"=w409, "x"=w409) -> ("dx/dt"=w412:dbl)  [unwired: 1 in, 1 out]
                      n191 = call <vilib>:"Derivative x(t) PtByPt.vi"("dt"=w408, "initial condition"=w407, "x"=w407) -> ("dx/dt"=w411:dbl)  [unwired: 1 in, 1 out]
                      n192 = call <vilib>:"Derivative x(t) PtByPt.vi"("dt"=w408, "initial condition"=w406, "x"=w406) -> ("dx/dt"=w410:dbl)  [unwired: 1 in, 1 out]
                    }
                    frame 2 {
                      n193 = call <vilib>:"Derivative x(t) PtByPt.vi"("dt"=w415, "initial condition"=w416, "x"=w416) -> ("dx/dt"=w419:dbl)  [unwired: 1 in, 1 out]
                      n194 = call <vilib>:"Derivative x(t) PtByPt.vi"("dt"=w415, "initial condition"=w414, "x"=w414) -> ("dx/dt"=w418:dbl)  [unwired: 1 in, 1 out]
                      n195 = call <vilib>:"Derivative x(t) PtByPt.vi"("dt"=w415, "initial condition"=w413, "x"=w413) -> ("dx/dt"=w417:dbl)  [unwired: 1 in, 1 out]
                    }
                    frame 3 {
                      n196 = call <vilib>:"Derivative x(t) PtByPt.vi"("dt"=w422, "initial condition"=w423, "x"=w423) -> ("dx/dt"=w426:dbl)  [unwired: 1 in, 1 out]
                      n197 = call <vilib>:"Derivative x(t) PtByPt.vi"("dt"=w422, "initial condition"=w421, "x"=w421) -> ("dx/dt"=w425:dbl)  [unwired: 1 in, 1 out]
                      n198 = call <vilib>:"Derivative x(t) PtByPt.vi"("dt"=w422, "initial condition"=w420, "x"=w420) -> ("dx/dt"=w424:dbl)  [unwired: 1 in, 1 out]
                    }
                    frame 4 {
                      n199 = call <vilib>:"Derivative x(t) PtByPt.vi"("dt"=w429, "initial condition"=w430, "x"=w430) -> ("dx/dt"=w433:dbl)  [unwired: 1 in, 1 out]
                      n200 = call <vilib>:"Derivative x(t) PtByPt.vi"("dt"=w429, "initial condition"=w428, "x"=w428) -> ("dx/dt"=w432:dbl)  [unwired: 1 in, 1 out]
                      n201 = call <vilib>:"Derivative x(t) PtByPt.vi"("dt"=w429, "initial condition"=w427, "x"=w427) -> ("dx/dt"=w431:dbl)  [unwired: 1 in, 1 out]
                    }
                    frame 5 {
                      n202 = call <vilib>:"Derivative x(t) PtByPt.vi"("dt"=w436, "initial condition"=w437, "x"=w437) -> ("dx/dt"=w440:dbl)  [unwired: 1 in, 1 out]
                      n203 = call <vilib>:"Derivative x(t) PtByPt.vi"("dt"=w436, "initial condition"=w435, "x"=w435) -> ("dx/dt"=w439:dbl)  [unwired: 1 in, 1 out]
                      n204 = call <vilib>:"Derivative x(t) PtByPt.vi"("dt"=w436, "initial condition"=w434, "x"=w434) -> ("dx/dt"=w438:dbl)  [unwired: 1 in, 1 out]
                    }
                  }
                  n205 = Build Array(w391, w395, w390, w394, w392, w393) -> (w389:dbl[])
                  n206 = call-poly <vilib>:"Array To Matrix.vi"("Real 1D Array"=w389) -> ("Real Matrix (Column Vector)"=w388:T3)
                  n207 = Bundle By Name(cluster=w396, "x_k|k"=w388) -> (w387:T2)
                }
              }
              frame True {
              }
            }
            n208 = Bundle By Name(cluster=w356, "robots_blue"=w361, "robots_yellow"=w360, "balls"=w352) -> (w359:T1)
            n209 = Bundle By Name(cluster=w356, "New"=FALSE) -> (w357:T1)
          }
          frame 3 {
            n210 = Empty Array?(array=w503) -> (empty?=w504:bool)
            n211 = Empty Array?(array=w511) -> (empty?=w512:bool)
            n212 = Reciprocal(x=w513) -> (1/x=w502:dbl)
            n213 = Empty Array?(array=w514) -> (empty?=w515:bool)
            n214 = case shown="False" w515 {
              tunnel: w514 -> [w592 w649]
              tunnel: w502 -> [w593 _]
              tunnel: [w591 w649] -> w510
              frame False {
                n215 = for {
                  tunnel: w592 -> [w606] mode=indexing
                  tunnel: w593 -> [w596]
                  tunnel: w592 -> [w604] mode=indexing
                  tunnel: [w595] -> w591 mode=indexing
                  n216 = Unbundle By Name(w606) -> ("x"=w594:sgl, "y"=w598:sgl, "orientation"=w597:sgl, "robot_id"=w605:u32)
                  n217 = case shown="0, Default" w605 {
                    tunnel: w594 -> [w607 w617 w624 w631 w638 w645]
                    tunnel: [w613 w620 w627 w634 w641 w648] -> w603
                    tunnel: [w612 w619 w626 w633 w640 w647] -> w602
                    tunnel: [w611 w618 w625 w632 w639 w646] -> w601
                    tunnel: w598 -> [w610 w616 w623 w630 w637 w644]
                    tunnel: w597 -> [w609 w615 w622 w629 w636 w643]
                    tunnel: w596 -> [w608 w614 w621 w628 w635 w642]
                    frame 0, Default {
                      n218 = call <vilib>:"Derivative x(t) PtByPt.vi"("dt"=w608, "initial condition"=w607, "x"=w607) -> ("dx/dt"=w613:dbl)  [unwired: 1 in, 1 out]
                      n219 = call <vilib>:"Derivative x(t) PtByPt.vi"("dt"=w608, "initial condition"=w610, "x"=w610) -> ("dx/dt"=w612:dbl)  [unwired: 1 in, 1 out]
                      n220 = call <vilib>:"Derivative x(t) PtByPt.vi"("dt"=w608, "initial condition"=w609, "x"=w609) -> ("dx/dt"=w611:dbl)  [unwired: 1 in, 1 out]
                    }
                    frame 1 {
                      n221 = call <vilib>:"Derivative x(t) PtByPt.vi"("dt"=w614, "initial condition"=w617, "x"=w617) -> ("dx/dt"=w620:dbl)  [unwired: 1 in, 1 out]
                      n222 = call <vilib>:"Derivative x(t) PtByPt.vi"("dt"=w614, "initial condition"=w616, "x"=w616) -> ("dx/dt"=w619:dbl)  [unwired: 1 in, 1 out]
                      n223 = call <vilib>:"Derivative x(t) PtByPt.vi"("dt"=w614, "initial condition"=w615, "x"=w615) -> ("dx/dt"=w618:dbl)  [unwired: 1 in, 1 out]
                    }
                    frame 2 {
                      n224 = call <vilib>:"Derivative x(t) PtByPt.vi"("dt"=w621, "initial condition"=w624, "x"=w624) -> ("dx/dt"=w627:dbl)  [unwired: 1 in, 1 out]
                      n225 = call <vilib>:"Derivative x(t) PtByPt.vi"("dt"=w621, "initial condition"=w623, "x"=w623) -> ("dx/dt"=w626:dbl)  [unwired: 1 in, 1 out]
                      n226 = call <vilib>:"Derivative x(t) PtByPt.vi"("dt"=w621, "initial condition"=w622, "x"=w622) -> ("dx/dt"=w625:dbl)  [unwired: 1 in, 1 out]
                    }
                    frame 3 {
                      n227 = call <vilib>:"Derivative x(t) PtByPt.vi"("dt"=w628, "initial condition"=w631, "x"=w631) -> ("dx/dt"=w634:dbl)  [unwired: 1 in, 1 out]
                      n228 = call <vilib>:"Derivative x(t) PtByPt.vi"("dt"=w628, "initial condition"=w630, "x"=w630) -> ("dx/dt"=w633:dbl)  [unwired: 1 in, 1 out]
                      n229 = call <vilib>:"Derivative x(t) PtByPt.vi"("dt"=w628, "initial condition"=w629, "x"=w629) -> ("dx/dt"=w632:dbl)  [unwired: 1 in, 1 out]
                    }
                    frame 4 {
                      n230 = call <vilib>:"Derivative x(t) PtByPt.vi"("dt"=w635, "initial condition"=w638, "x"=w638) -> ("dx/dt"=w641:dbl)  [unwired: 1 in, 1 out]
                      n231 = call <vilib>:"Derivative x(t) PtByPt.vi"("dt"=w635, "initial condition"=w637, "x"=w637) -> ("dx/dt"=w640:dbl)  [unwired: 1 in, 1 out]
                      n232 = call <vilib>:"Derivative x(t) PtByPt.vi"("dt"=w635, "initial condition"=w636, "x"=w636) -> ("dx/dt"=w639:dbl)  [unwired: 1 in, 1 out]
                    }
                    frame 5 {
                      n233 = call <vilib>:"Derivative x(t) PtByPt.vi"("dt"=w642, "initial condition"=w645, "x"=w645) -> ("dx/dt"=w648:dbl)  [unwired: 1 in, 1 out]
                      n234 = call <vilib>:"Derivative x(t) PtByPt.vi"("dt"=w642, "initial condition"=w644, "x"=w644) -> ("dx/dt"=w647:dbl)  [unwired: 1 in, 1 out]
                      n235 = call <vilib>:"Derivative x(t) PtByPt.vi"("dt"=w642, "initial condition"=w643, "x"=w643) -> ("dx/dt"=w646:dbl)  [unwired: 1 in, 1 out]
                    }
                  }
                  n236 = Build Array(w594, w603, w598, w602, w597, w601) -> (w600:dbl[])
                  n237 = call-poly <vilib>:"Array To Matrix.vi"("Real 1D Array"=w600) -> ("Real Matrix (Column Vector)"=w599:T3)
                  n238 = Bundle By Name(cluster=w604, "x_k|k"=w599) -> (w595:T2)
                }
              }
              frame True {
              }
            }
            n239 = case shown="False" w504 {
              tunnel: w503 -> [w517 w531]
              tunnel: w502 -> [w518 _]
              tunnel: [w516 w531] -> w501
              frame False {
                n240 = for {
                  tunnel: w517 -> [w530] mode=indexing
                  tunnel: w518 -> [w519]
                  tunnel: w517 -> [w529] mode=indexing
                  tunnel: [w520] -> w516 mode=indexing
                  n241 = Unbundle By Name(w530) -> ("x"=w524:sgl, "y"=w523:sgl, "z"=w525:sgl)
                  n242 = call <vilib>:"Derivative x(t) PtByPt.vi"("dt"=w519, "initial condition"=w524, "x"=w524) -> ("dx/dt"=w528:dbl)  [unwired: 1 in, 1 out]
                  n243 = call <vilib>:"Derivative x(t) PtByPt.vi"("dt"=w519, "initial condition"=w523, "x"=w523) -> ("dx/dt"=w527:dbl)  [unwired: 1 in, 1 out]
                  n244 = call <vilib>:"Derivative x(t) PtByPt.vi"("dt"=w519, "initial condition"=w525, "x"=w525) -> ("dx/dt"=w526:dbl)  [unwired: 1 in, 1 out]
                  n245 = Build Array(w524, w528, w523, w527, w525, w526) -> (w522:dbl[])
                  n246 = call-poly <vilib>:"Array To Matrix.vi"("Real 1D Array"=w522) -> ("Real Matrix (Column Vector)"=w521:T3)
                  n247 = Bundle By Name(cluster=w529, "x_k|k"=w521) -> (w520:T4)
                }
              }
              frame True {
              }
            }
            n248 = case shown="False" w512 {
              tunnel: w511 -> [w533 w590]
              tunnel: w502 -> [w534 _]
              tunnel: [w532 w590] -> w509
              frame False {
                n249 = for {
                  tunnel: w533 -> [w547] mode=indexing
                  tunnel: w534 -> [w535]
                  tunnel: w533 -> [w545] mode=indexing
                  tunnel: [w536] -> w532 mode=indexing
                  n250 = Unbundle By Name(w547) -> ("x"=w540:sgl, "y"=w539:sgl, "orientation"=w541:sgl, "robot_id"=w546:u32)
                  n251 = case shown="0, Default" w546 {
                    tunnel: w540 -> [w551 w558 w565 w572 w579 w586]
                    tunnel: w539 -> [w549 w556 w563 w570 w577 w584]
                    tunnel: w541 -> [w548 w555 w562 w569 w576 w583]
                    tunnel: [w554 w561 w568 w575 w582 w589] -> w544
                    tunnel: [w553 w560 w567 w574 w581 w588] -> w543
                    tunnel: [w552 w559 w566 w573 w580 w587] -> w542
                    tunnel: w535 -> [w550 w557 w564 w571 w578 w585]
                    frame 0, Default {
                      n252 = call <vilib>:"Derivative x(t) PtByPt.vi"("dt"=w550, "initial condition"=w551, "x"=w551) -> ("dx/dt"=w554:dbl)  [unwired: 1 in, 1 out]
                      n253 = call <vilib>:"Derivative x(t) PtByPt.vi"("dt"=w550, "initial condition"=w549, "x"=w549) -> ("dx/dt"=w553:dbl)  [unwired: 1 in, 1 out]
                      n254 = call <vilib>:"Derivative x(t) PtByPt.vi"("dt"=w550, "initial condition"=w548, "x"=w548) -> ("dx/dt"=w552:dbl)  [unwired: 1 in, 1 out]
                    }
                    frame 1 {
                      n255 = call <vilib>:"Derivative x(t) PtByPt.vi"("dt"=w557, "initial condition"=w558, "x"=w558) -> ("dx/dt"=w561:dbl)  [unwired: 1 in, 1 out]
                      n256 = call <vilib>:"Derivative x(t) PtByPt.vi"("dt"=w557, "initial condition"=w556, "x"=w556) -> ("dx/dt"=w560:dbl)  [unwired: 1 in, 1 out]
                      n257 = call <vilib>:"Derivative x(t) PtByPt.vi"("dt"=w557, "initial condition"=w555, "x"=w555) -> ("dx/dt"=w559:dbl)  [unwired: 1 in, 1 out]
                    }
                    frame 2 {
                      n258 = call <vilib>:"Derivative x(t) PtByPt.vi"("dt"=w564, "initial condition"=w565, "x"=w565) -> ("dx/dt"=w568:dbl)  [unwired: 1 in, 1 out]
                      n259 = call <vilib>:"Derivative x(t) PtByPt.vi"("dt"=w564, "initial condition"=w563, "x"=w563) -> ("dx/dt"=w567:dbl)  [unwired: 1 in, 1 out]
                      n260 = call <vilib>:"Derivative x(t) PtByPt.vi"("dt"=w564, "initial condition"=w562, "x"=w562) -> ("dx/dt"=w566:dbl)  [unwired: 1 in, 1 out]
                    }
                    frame 3 {
                      n261 = call <vilib>:"Derivative x(t) PtByPt.vi"("dt"=w571, "initial condition"=w572, "x"=w572) -> ("dx/dt"=w575:dbl)  [unwired: 1 in, 1 out]
                      n262 = call <vilib>:"Derivative x(t) PtByPt.vi"("dt"=w571, "initial condition"=w570, "x"=w570) -> ("dx/dt"=w574:dbl)  [unwired: 1 in, 1 out]
                      n263 = call <vilib>:"Derivative x(t) PtByPt.vi"("dt"=w571, "initial condition"=w569, "x"=w569) -> ("dx/dt"=w573:dbl)  [unwired: 1 in, 1 out]
                    }
                    frame 4 {
                      n264 = call <vilib>:"Derivative x(t) PtByPt.vi"("dt"=w578, "initial condition"=w579, "x"=w579) -> ("dx/dt"=w582:dbl)  [unwired: 1 in, 1 out]
                      n265 = call <vilib>:"Derivative x(t) PtByPt.vi"("dt"=w578, "initial condition"=w577, "x"=w577) -> ("dx/dt"=w581:dbl)  [unwired: 1 in, 1 out]
                      n266 = call <vilib>:"Derivative x(t) PtByPt.vi"("dt"=w578, "initial condition"=w576, "x"=w576) -> ("dx/dt"=w580:dbl)  [unwired: 1 in, 1 out]
                    }
                    frame 5 {
                      n267 = call <vilib>:"Derivative x(t) PtByPt.vi"("dt"=w585, "initial condition"=w586, "x"=w586) -> ("dx/dt"=w589:dbl)  [unwired: 1 in, 1 out]
                      n268 = call <vilib>:"Derivative x(t) PtByPt.vi"("dt"=w585, "initial condition"=w584, "x"=w584) -> ("dx/dt"=w588:dbl)  [unwired: 1 in, 1 out]
                      n269 = call <vilib>:"Derivative x(t) PtByPt.vi"("dt"=w585, "initial condition"=w583, "x"=w583) -> ("dx/dt"=w587:dbl)  [unwired: 1 in, 1 out]
                    }
                  }
                  n270 = Build Array(w540, w544, w539, w543, w541, w542) -> (w538:dbl[])
                  n271 = call-poly <vilib>:"Array To Matrix.vi"("Real 1D Array"=w538) -> ("Real Matrix (Column Vector)"=w537:T3)
                  n272 = Bundle By Name(cluster=w545, "x_k|k"=w537) -> (w536:T2)
                }
              }
              frame True {
              }
            }
            n273 = Bundle By Name(cluster=w505, "robots_blue"=w510, "robots_yellow"=w509, "balls"=w501) -> (w508:T1)
            n274 = Bundle By Name(cluster=w505, "New"=FALSE) -> (w506:T1)
          }
        }
      }
      frame "Variable2ndDerivate" {
        n275 = call "SSL Detection Frame Simple Estimator Kalman VelCmd.vi"("Lado"=w661, "Time"=w662, "Enable"=FALSE, "Detection Frame In"=w652) -> ("Detection Frame Out"=w651:T1)  [unwired: 6 in, 1 out]
        n276 = Unbundle By Name(w651) -> ("robots_blue"=w660:T2[], "robots_yellow"=w659:T2[], "camera_id"=w656:u32, "balls"=w655:T4[], "t_capture"=w653:dbl)
        n277 = case shown="0, Default" w656 {
          tunnel: w660 -> [w677 w971 w1265 w1559]
          tunnel: 60.0 -> [w676 w970 w1264 w1558]
          tunnel: w659 -> [w674 w968 w1262 w1556]
          tunnel: [w671 w965 w1259 w1553] -> w658
          tunnel: [w669 w963 w1257 w1551] -> w657
          tunnel: w651 -> [w668 w962 w1256 w1550]
          tunnel: w655 -> [w666 w960 w1254 w1548]
          tunnel: w653 -> [w663 w957 w1251 w1545]
          frame 0, Default {
            n278 = Empty Array?(array=w666) -> (empty?=w667:bool)
            n279 = Empty Array?(array=w674) -> (empty?=w675:bool)
            n280 = Reciprocal(x=w676) -> (1/x=w665:dbl)
            n281 = Empty Array?(array=w677) -> (empty?=w678:bool)
            n282 = case shown="False" w678 {
              tunnel: w677 -> [w829 w956]
              tunnel: w665 -> [w830 _]
              tunnel: [w828 w956] -> w673
              tunnel: w663 -> [w827 _]
              frame False {
                n283 = for {
                  tunnel: w829 -> [w843] mode=indexing
                  tunnel: w830 -> [_]
                  tunnel: w829 -> [w841] mode=indexing
                  tunnel: [w833] -> w828 mode=indexing
                  tunnel: w827 -> [w831]
                  n284 = Unbundle By Name(w843) -> ("x"=w832:sgl, "y"=w835:sgl, "orientation"=w834:sgl, "robot_id"=w842:u32)
                  n285 = case shown="2" w842 {
                    tunnel: w832 -> [w846 w853 w860 w867 w874 w881 w888 w895 w902 w909 w916 w923 w930 w937 w944 w951]
                    tunnel: [w848 w855 w862 w869 w876 w883 w890 w897 w904 w911 w918 w925 w932 w939 w946 w953] -> w840
                    tunnel: [w850 w857 w864 w871 w878 w885 w892 w899 w906 w913 w920 w927 w934 w941 w948 w955] -> w839
                    tunnel: [w849 w856 w863 w870 w877 w884 w891 w898 w905 w912 w919 w926 w933 w940 w947 w954] -> w838
                    tunnel: w835 -> [w845 w852 w859 w866 w873 w880 w887 w894 w901 w908 w915 w922 w929 w936 w943 w950]
                    tunnel: w834 -> [w844 w851 w858 w865 w872 w879 w886 w893 w900 w907 w914 w921 w928 w935 w942 w949]
                    tunnel: w831 -> [w847 w854 w861 w868 w875 w882 w889 w896 w903 w910 w917 w924 w931 w938 w945 w952]
                    frame 0, Default {
                      n286 = call "2ndOrderDerivate.vi"("t_capture"=w847, "initial condition"=w846, "x"=w846) -> ("dx/dt"=w848:dbl)  [unwired: 5 in, 3 out]
                      n287 = call "2ndOrderDerivate.vi"("t_capture"=w847, "initial condition"=w845, "x"=w845) -> ("dx/dt"=w850:dbl)  [unwired: 5 in, 3 out]
                      n288 = call "2ndOrderDerivate.vi"("t_capture"=w847, "initial condition"=w844, "x"=w844) -> ("dx/dt"=w849:dbl)  [unwired: 5 in, 3 out]
                    }
                    frame 1 {
                      n289 = call "2ndOrderDerivate.vi"("t_capture"=w854, "initial condition"=w853, "x"=w853) -> ("dx/dt"=w855:dbl)  [unwired: 5 in, 3 out]
                      n290 = call "2ndOrderDerivate.vi"("t_capture"=w854, "initial condition"=w852, "x"=w852) -> ("dx/dt"=w857:dbl)  [unwired: 5 in, 3 out]
                      n291 = call "2ndOrderDerivate.vi"("t_capture"=w854, "initial condition"=w851, "x"=w851) -> ("dx/dt"=w856:dbl)  [unwired: 5 in, 3 out]
                    }
                    frame 2 {
                      n292 = call "2ndOrderDerivate.vi"("t_capture"=w861, "initial condition"=w860, "x"=w860) -> ("dx/dt"=w862:dbl)  [unwired: 5 in, 3 out]
                      n293 = call "2ndOrderDerivate.vi"("t_capture"=w861, "initial condition"=w859, "x"=w859) -> ("dx/dt"=w864:dbl)  [unwired: 5 in, 3 out]
                      n294 = call "2ndOrderDerivate.vi"("t_capture"=w861, "initial condition"=w858, "x"=w858) -> ("dx/dt"=w863:dbl)  [unwired: 5 in, 3 out]
                    }
                    frame 3 {
                      n295 = call "2ndOrderDerivate.vi"("t_capture"=w868, "initial condition"=w867, "x"=w867) -> ("dx/dt"=w869:dbl)  [unwired: 5 in, 3 out]
                      n296 = call "2ndOrderDerivate.vi"("t_capture"=w868, "initial condition"=w866, "x"=w866) -> ("dx/dt"=w871:dbl)  [unwired: 5 in, 3 out]
                      n297 = call "2ndOrderDerivate.vi"("t_capture"=w868, "initial condition"=w865, "x"=w865) -> ("dx/dt"=w870:dbl)  [unwired: 5 in, 3 out]
                    }
                    frame 4 {
                      n298 = call "2ndOrderDerivate.vi"("t_capture"=w875, "initial condition"=w874, "x"=w874) -> ("dx/dt"=w876:dbl)  [unwired: 5 in, 3 out]
                      n299 = call "2ndOrderDerivate.vi"("t_capture"=w875, "initial condition"=w873, "x"=w873) -> ("dx/dt"=w878:dbl)  [unwired: 5 in, 3 out]
                      n300 = call "2ndOrderDerivate.vi"("t_capture"=w875, "initial condition"=w872, "x"=w872) -> ("dx/dt"=w877:dbl)  [unwired: 5 in, 3 out]
                    }
                    frame 5 {
                      n301 = call "2ndOrderDerivate.vi"("t_capture"=w882, "initial condition"=w881, "x"=w881) -> ("dx/dt"=w883:dbl)  [unwired: 5 in, 3 out]
                      n302 = call "2ndOrderDerivate.vi"("t_capture"=w882, "initial condition"=w880, "x"=w880) -> ("dx/dt"=w885:dbl)  [unwired: 5 in, 3 out]
                      n303 = call "2ndOrderDerivate.vi"("t_capture"=w882, "initial condition"=w879, "x"=w879) -> ("dx/dt"=w884:dbl)  [unwired: 5 in, 3 out]
                    }
                    frame 6 {
                      n304 = call "2ndOrderDerivate.vi"("t_capture"=w889, "initial condition"=w888, "x"=w888) -> ("dx/dt"=w890:dbl)  [unwired: 5 in, 3 out]
                      n305 = call "2ndOrderDerivate.vi"("t_capture"=w889, "initial condition"=w887, "x"=w887) -> ("dx/dt"=w892:dbl)  [unwired: 5 in, 3 out]
                      n306 = call "2ndOrderDerivate.vi"("t_capture"=w889, "initial condition"=w886, "x"=w886) -> ("dx/dt"=w891:dbl)  [unwired: 5 in, 3 out]
                    }
                    frame 7 {
                      n307 = call "2ndOrderDerivate.vi"("t_capture"=w896, "initial condition"=w895, "x"=w895) -> ("dx/dt"=w897:dbl)  [unwired: 5 in, 3 out]
                      n308 = call "2ndOrderDerivate.vi"("t_capture"=w896, "initial condition"=w894, "x"=w894) -> ("dx/dt"=w899:dbl)  [unwired: 5 in, 3 out]
                      n309 = call "2ndOrderDerivate.vi"("t_capture"=w896, "initial condition"=w893, "x"=w893) -> ("dx/dt"=w898:dbl)  [unwired: 5 in, 3 out]
                    }
                    frame 8 {
                      n310 = call "2ndOrderDerivate.vi"("t_capture"=w903, "initial condition"=w902, "x"=w902) -> ("dx/dt"=w904:dbl)  [unwired: 5 in, 3 out]
                      n311 = call "2ndOrderDerivate.vi"("t_capture"=w903, "initial condition"=w901, "x"=w901) -> ("dx/dt"=w906:dbl)  [unwired: 5 in, 3 out]
                      n312 = call "2ndOrderDerivate.vi"("t_capture"=w903, "initial condition"=w900, "x"=w900) -> ("dx/dt"=w905:dbl)  [unwired: 5 in, 3 out]
                    }
                    frame 9 {
                      n313 = call "2ndOrderDerivate.vi"("t_capture"=w910, "initial condition"=w909, "x"=w909) -> ("dx/dt"=w911:dbl)  [unwired: 5 in, 3 out]
                      n314 = call "2ndOrderDerivate.vi"("t_capture"=w910, "initial condition"=w908, "x"=w908) -> ("dx/dt"=w913:dbl)  [unwired: 5 in, 3 out]
                      n315 = call "2ndOrderDerivate.vi"("t_capture"=w910, "initial condition"=w907, "x"=w907) -> ("dx/dt"=w912:dbl)  [unwired: 5 in, 3 out]
                    }
                    frame 10 {
                      n316 = call "2ndOrderDerivate.vi"("t_capture"=w917, "initial condition"=w916, "x"=w916) -> ("dx/dt"=w918:dbl)  [unwired: 5 in, 3 out]
                      n317 = call "2ndOrderDerivate.vi"("t_capture"=w917, "initial condition"=w915, "x"=w915) -> ("dx/dt"=w920:dbl)  [unwired: 5 in, 3 out]
                      n318 = call "2ndOrderDerivate.vi"("t_capture"=w917, "initial condition"=w914, "x"=w914) -> ("dx/dt"=w919:dbl)  [unwired: 5 in, 3 out]
                    }
                    frame 11 {
                      n319 = call "2ndOrderDerivate.vi"("t_capture"=w924, "initial condition"=w923, "x"=w923) -> ("dx/dt"=w925:dbl)  [unwired: 5 in, 3 out]
                      n320 = call "2ndOrderDerivate.vi"("t_capture"=w924, "initial condition"=w922, "x"=w922) -> ("dx/dt"=w927:dbl)  [unwired: 5 in, 3 out]
                      n321 = call "2ndOrderDerivate.vi"("t_capture"=w924, "initial condition"=w921, "x"=w921) -> ("dx/dt"=w926:dbl)  [unwired: 5 in, 3 out]
                    }
                    frame 12 {
                      n322 = call "2ndOrderDerivate.vi"("t_capture"=w931, "initial condition"=w930, "x"=w930) -> ("dx/dt"=w932:dbl)  [unwired: 5 in, 3 out]
                      n323 = call "2ndOrderDerivate.vi"("t_capture"=w931, "initial condition"=w929, "x"=w929) -> ("dx/dt"=w934:dbl)  [unwired: 5 in, 3 out]
                      n324 = call "2ndOrderDerivate.vi"("t_capture"=w931, "initial condition"=w928, "x"=w928) -> ("dx/dt"=w933:dbl)  [unwired: 5 in, 3 out]
                    }
                    frame 13 {
                      n325 = call "2ndOrderDerivate.vi"("t_capture"=w938, "initial condition"=w937, "x"=w937) -> ("dx/dt"=w939:dbl)  [unwired: 5 in, 3 out]
                      n326 = call "2ndOrderDerivate.vi"("t_capture"=w938, "initial condition"=w936, "x"=w936) -> ("dx/dt"=w941:dbl)  [unwired: 5 in, 3 out]
                      n327 = call "2ndOrderDerivate.vi"("t_capture"=w938, "initial condition"=w935, "x"=w935) -> ("dx/dt"=w940:dbl)  [unwired: 5 in, 3 out]
                    }
                    frame 14 {
                      n328 = call "2ndOrderDerivate.vi"("t_capture"=w945, "initial condition"=w944, "x"=w944) -> ("dx/dt"=w946:dbl)  [unwired: 5 in, 3 out]
                      n329 = call "2ndOrderDerivate.vi"("t_capture"=w945, "initial condition"=w943, "x"=w943) -> ("dx/dt"=w948:dbl)  [unwired: 5 in, 3 out]
                      n330 = call "2ndOrderDerivate.vi"("t_capture"=w945, "initial condition"=w942, "x"=w942) -> ("dx/dt"=w947:dbl)  [unwired: 5 in, 3 out]
                    }
                    frame 15 {
                      n331 = call "2ndOrderDerivate.vi"("t_capture"=w952, "initial condition"=w951, "x"=w951) -> ("dx/dt"=w953:dbl)  [unwired: 5 in, 3 out]
                      n332 = call "2ndOrderDerivate.vi"("t_capture"=w952, "initial condition"=w950, "x"=w950) -> ("dx/dt"=w955:dbl)  [unwired: 5 in, 3 out]
                      n333 = call "2ndOrderDerivate.vi"("t_capture"=w952, "initial condition"=w949, "x"=w949) -> ("dx/dt"=w954:dbl)  [unwired: 5 in, 3 out]
                    }
                  }
                  n334 = Build Array(w832, w840, w835, w839, w834, w838) -> (w837:dbl[])
                  n335 = call-poly <vilib>:"Array To Matrix.vi"("Real 1D Array"=w837) -> ("Real Matrix (Column Vector)"=w836:T3)
                  n336 = Bundle By Name(cluster=w841, "x_k|k"=w836) -> (w833:T2)
                }
              }
              frame True {
              }
            }
            n337 = case shown="False" w667 {
              tunnel: w666 -> [w681 w695]
              tunnel: w665 -> [w682 _]
              tunnel: [w680 w695] -> w664
              tunnel: w663 -> [w679 _]
              frame False {
                n338 = for {
                  tunnel: w681 -> [w694] mode=indexing
                  tunnel: w682 -> [_]
                  tunnel: w681 -> [w693] mode=indexing
                  tunnel: [w690] -> w680 mode=indexing
                  tunnel: w679 -> [w688]
                  n339 = Unbundle By Name(w694) -> ("x"=w689:sgl, "y"=w687:sgl, "z"=w683:sgl)
                  n340 = call "2ndOrderDerivate.vi"("t_capture"=w688, "initial condition"=w687, "x"=w687) -> ("dx/dt"=w685:dbl)  [unwired: 5 in, 3 out]
                  n341 = call "2ndOrderDerivate.vi"("t_capture"=w688, "initial condition"=w689, "x"=w689) -> ("dx/dt"=w686:dbl)  [unwired: 5 in, 3 out]
                  n342 = call "2ndOrderDerivate.vi"("t_capture"=w688, "initial condition"=w683, "x"=w683) -> ("dx/dt"=w684:dbl)  [unwired: 5 in, 3 out]
                  n343 = Build Array(w689, w686, w687, w685, w683, w684) -> (w692:dbl[])
                  n344 = call-poly <vilib>:"Array To Matrix.vi"("Real 1D Array"=w692) -> ("Real Matrix (Column Vector)"=w691:T3)
                  n345 = Bundle By Name(cluster=w693, "x_k|k"=w691) -> (w690:T4)
                }
              }
              frame True {
              }
            }
            n346 = case shown="False" w675 {
              tunnel: w674 -> [w698 w826]
              tunnel: w665 -> [w699 _]
              tunnel: [w697 w826] -> w672
              tunnel: w663 -> [w696 _]
              frame False {
                n347 = for {
                  tunnel: w698 -> [w713] mode=indexing
                  tunnel: w699 -> [w701]
                  tunnel: w698 -> [w711] mode=indexing
                  tunnel: [w702] -> w697 mode=indexing
                  tunnel: w696 -> [w700]
                  n348 = Unbundle By Name(w713) -> ("x"=w706:sgl, "y"=w705:sgl, "orientation"=w707:sgl, "robot_id"=w712:u32)
                  n349 = case shown="1" w712 {
                    tunnel: w706 -> [w720 w727 w734 w741 w748 w755 w762 w769 w776 w783 w790 w797 w804 w811 w818 w825]
                    tunnel: w705 -> [w718 w725 w732 w739 w746 w753 w760 w767 w774 w781 w788 w795 w802 w809 w816 w823]
                    tunnel: w707 -> [w717 w724 w731 w738 w745 w752 w759 w766 w773 w780 w787 w794 w801 w808 w815 w822]
                    tunnel: [w716 w723 w730 w737 w744 w751 w758 w765 w772 w779 w786 w793 w800 w807 w814 w821] -> w710
                    tunnel: [w715 w722 w729 w736 w743 w750 w757 w764 w771 w778 w785 w792 w799 w806 w813 w820] -> w709
                    tunnel: [w714 w721 w728 w735 w742 w749 w756 w763 w770 w777 w784 w791 w798 w805 w812 w819] -> w708
                    tunnel: w701 -> [_ _ _ _ _ _ _ _ _ _ _ _ _ _ _ _]
                    tunnel: w700 -> [w719 w726 w733 w740 w747 w754 w761 w768 w775 w782 w789 w796 w803 w810 w817 w824]
                    frame 0, Default {
                      n350 = call "2ndOrderDerivate.vi"("t_capture"=w719, "initial condition"=w720, "x"=w720) -> ("dx/dt"=w716:dbl)  [unwired: 5 in, 3 out]
                      n351 = call "2ndOrderDerivate.vi"("t_capture"=w719, "initial condition"=w718, "x"=w718) -> ("dx/dt"=w715:dbl)  [unwired: 5 in, 3 out]
                      n352 = call "2ndOrderDerivate.vi"("t_capture"=w719, "initial condition"=w717, "x"=w717) -> ("dx/dt"=w714:dbl)  [unwired: 5 in, 3 out]
                    }
                    frame 1 {
                      n353 = call "2ndOrderDerivate.vi"("t_capture"=w726, "initial condition"=w727, "x"=w727) -> ("dx/dt"=w723:dbl)  [unwired: 5 in, 3 out]
                      n354 = call "2ndOrderDerivate.vi"("t_capture"=w726, "initial condition"=w725, "x"=w725) -> ("dx/dt"=w722:dbl)  [unwired: 5 in, 3 out]
                      n355 = call "2ndOrderDerivate.vi"("t_capture"=w726, "initial condition"=w724, "x"=w724) -> ("dx/dt"=w721:dbl)  [unwired: 5 in, 3 out]
                    }
                    frame 2 {
                      n356 = call "2ndOrderDerivate.vi"("t_capture"=w733, "initial condition"=w734, "x"=w734) -> ("dx/dt"=w730:dbl)  [unwired: 5 in, 3 out]
                      n357 = call "2ndOrderDerivate.vi"("t_capture"=w733, "initial condition"=w732, "x"=w732) -> ("dx/dt"=w729:dbl)  [unwired: 5 in, 3 out]
                      n358 = call "2ndOrderDerivate.vi"("t_capture"=w733, "initial condition"=w731, "x"=w731) -> ("dx/dt"=w728:dbl)  [unwired: 5 in, 3 out]
                    }
                    frame 3 {
                      n359 = call "2ndOrderDerivate.vi"("t_capture"=w740, "initial condition"=w741, "x"=w741) -> ("dx/dt"=w737:dbl)  [unwired: 5 in, 3 out]
                      n360 = call "2ndOrderDerivate.vi"("t_capture"=w740, "initial condition"=w739, "x"=w739) -> ("dx/dt"=w736:dbl)  [unwired: 5 in, 3 out]
                      n361 = call "2ndOrderDerivate.vi"("t_capture"=w740, "initial condition"=w738, "x"=w738) -> ("dx/dt"=w735:dbl)  [unwired: 5 in, 3 out]
                    }
                    frame 4 {
                      n362 = call "2ndOrderDerivate.vi"("t_capture"=w747, "initial condition"=w748, "x"=w748) -> ("dx/dt"=w744:dbl)  [unwired: 5 in, 3 out]
                      n363 = call "2ndOrderDerivate.vi"("t_capture"=w747, "initial condition"=w746, "x"=w746) -> ("dx/dt"=w743:dbl)  [unwired: 5 in, 3 out]
                      n364 = call "2ndOrderDerivate.vi"("t_capture"=w747, "initial condition"=w745, "x"=w745) -> ("dx/dt"=w742:dbl)  [unwired: 5 in, 3 out]
                    }
                    frame 5 {
                      n365 = call "2ndOrderDerivate.vi"("t_capture"=w754, "initial condition"=w755, "x"=w755) -> ("dx/dt"=w751:dbl)  [unwired: 5 in, 3 out]
                      n366 = call "2ndOrderDerivate.vi"("t_capture"=w754, "initial condition"=w753, "x"=w753) -> ("dx/dt"=w750:dbl)  [unwired: 5 in, 3 out]
                      n367 = call "2ndOrderDerivate.vi"("t_capture"=w754, "initial condition"=w752, "x"=w752) -> ("dx/dt"=w749:dbl)  [unwired: 5 in, 3 out]
                    }
                    frame 6 {
                      n368 = call "2ndOrderDerivate.vi"("t_capture"=w761, "initial condition"=w762, "x"=w762) -> ("dx/dt"=w758:dbl)  [unwired: 5 in, 3 out]
                      n369 = call "2ndOrderDerivate.vi"("t_capture"=w761, "initial condition"=w760, "x"=w760) -> ("dx/dt"=w757:dbl)  [unwired: 5 in, 3 out]
                      n370 = call "2ndOrderDerivate.vi"("t_capture"=w761, "initial condition"=w759, "x"=w759) -> ("dx/dt"=w756:dbl)  [unwired: 5 in, 3 out]
                    }
                    frame 7 {
                      n371 = call "2ndOrderDerivate.vi"("t_capture"=w768, "initial condition"=w769, "x"=w769) -> ("dx/dt"=w765:dbl)  [unwired: 5 in, 3 out]
                      n372 = call "2ndOrderDerivate.vi"("t_capture"=w768, "initial condition"=w767, "x"=w767) -> ("dx/dt"=w764:dbl)  [unwired: 5 in, 3 out]
                      n373 = call "2ndOrderDerivate.vi"("t_capture"=w768, "initial condition"=w766, "x"=w766) -> ("dx/dt"=w763:dbl)  [unwired: 5 in, 3 out]
                    }
                    frame 8 {
                      n374 = call "2ndOrderDerivate.vi"("t_capture"=w775, "initial condition"=w776, "x"=w776) -> ("dx/dt"=w772:dbl)  [unwired: 5 in, 3 out]
                      n375 = call "2ndOrderDerivate.vi"("t_capture"=w775, "initial condition"=w774, "x"=w774) -> ("dx/dt"=w771:dbl)  [unwired: 5 in, 3 out]
                      n376 = call "2ndOrderDerivate.vi"("t_capture"=w775, "initial condition"=w773, "x"=w773) -> ("dx/dt"=w770:dbl)  [unwired: 5 in, 3 out]
                    }
                    frame 9 {
                      n377 = call "2ndOrderDerivate.vi"("t_capture"=w782, "initial condition"=w783, "x"=w783) -> ("dx/dt"=w779:dbl)  [unwired: 5 in, 3 out]
                      n378 = call "2ndOrderDerivate.vi"("t_capture"=w782, "initial condition"=w781, "x"=w781) -> ("dx/dt"=w778:dbl)  [unwired: 5 in, 3 out]
                      n379 = call "2ndOrderDerivate.vi"("t_capture"=w782, "initial condition"=w780, "x"=w780) -> ("dx/dt"=w777:dbl)  [unwired: 5 in, 3 out]
                    }
                    frame 10 {
                      n380 = call "2ndOrderDerivate.vi"("t_capture"=w789, "initial condition"=w790, "x"=w790) -> ("dx/dt"=w786:dbl)  [unwired: 5 in, 3 out]
                      n381 = call "2ndOrderDerivate.vi"("t_capture"=w789, "initial condition"=w788, "x"=w788) -> ("dx/dt"=w785:dbl)  [unwired: 5 in, 3 out]
                      n382 = call "2ndOrderDerivate.vi"("t_capture"=w789, "initial condition"=w787, "x"=w787) -> ("dx/dt"=w784:dbl)  [unwired: 5 in, 3 out]
                    }
                    frame 11 {
                      n383 = call "2ndOrderDerivate.vi"("t_capture"=w796, "initial condition"=w797, "x"=w797) -> ("dx/dt"=w793:dbl)  [unwired: 5 in, 3 out]
                      n384 = call "2ndOrderDerivate.vi"("t_capture"=w796, "initial condition"=w795, "x"=w795) -> ("dx/dt"=w792:dbl)  [unwired: 5 in, 3 out]
                      n385 = call "2ndOrderDerivate.vi"("t_capture"=w796, "initial condition"=w794, "x"=w794) -> ("dx/dt"=w791:dbl)  [unwired: 5 in, 3 out]
                    }
                    frame 12 {
                      n386 = call "2ndOrderDerivate.vi"("t_capture"=w803, "initial condition"=w804, "x"=w804) -> ("dx/dt"=w800:dbl)  [unwired: 5 in, 3 out]
                      n387 = call "2ndOrderDerivate.vi"("t_capture"=w803, "initial condition"=w802, "x"=w802) -> ("dx/dt"=w799:dbl)  [unwired: 5 in, 3 out]
                      n388 = call "2ndOrderDerivate.vi"("t_capture"=w803, "initial condition"=w801, "x"=w801) -> ("dx/dt"=w798:dbl)  [unwired: 5 in, 3 out]
                    }
                    frame 13 {
                      n389 = call "2ndOrderDerivate.vi"("t_capture"=w810, "initial condition"=w811, "x"=w811) -> ("dx/dt"=w807:dbl)  [unwired: 5 in, 3 out]
                      n390 = call "2ndOrderDerivate.vi"("t_capture"=w810, "initial condition"=w809, "x"=w809) -> ("dx/dt"=w806:dbl)  [unwired: 5 in, 3 out]
                      n391 = call "2ndOrderDerivate.vi"("t_capture"=w810, "initial condition"=w808, "x"=w808) -> ("dx/dt"=w805:dbl)  [unwired: 5 in, 3 out]
                    }
                    frame 14 {
                      n392 = call "2ndOrderDerivate.vi"("t_capture"=w817, "initial condition"=w818, "x"=w818) -> ("dx/dt"=w814:dbl)  [unwired: 5 in, 3 out]
                      n393 = call "2ndOrderDerivate.vi"("t_capture"=w817, "initial condition"=w816, "x"=w816) -> ("dx/dt"=w813:dbl)  [unwired: 5 in, 3 out]
                      n394 = call "2ndOrderDerivate.vi"("t_capture"=w817, "initial condition"=w815, "x"=w815) -> ("dx/dt"=w812:dbl)  [unwired: 5 in, 3 out]
                    }
                    frame 15 {
                      n395 = call "2ndOrderDerivate.vi"("t_capture"=w824, "initial condition"=w825, "x"=w825) -> ("dx/dt"=w821:dbl)  [unwired: 5 in, 3 out]
                      n396 = call "2ndOrderDerivate.vi"("t_capture"=w824, "initial condition"=w823, "x"=w823) -> ("dx/dt"=w820:dbl)  [unwired: 5 in, 3 out]
                      n397 = call "2ndOrderDerivate.vi"("t_capture"=w824, "initial condition"=w822, "x"=w822) -> ("dx/dt"=w819:dbl)  [unwired: 5 in, 3 out]
                    }
                  }
                  n398 = Build Array(w706, w710, w705, w709, w707, w708) -> (w704:dbl[])
                  n399 = call-poly <vilib>:"Array To Matrix.vi"("Real 1D Array"=w704) -> ("Real Matrix (Column Vector)"=w703:T3)
                  n400 = Bundle By Name(cluster=w711, "x_k|k"=w703) -> (w702:T2)
                }
              }
              frame True {
              }
            }
            n401 = Bundle By Name(cluster=w668, "robots_blue"=w673, "robots_yellow"=w672, "balls"=w664) -> (w671:T1)
            n402 = Bundle By Name(cluster=w668, "New"=FALSE) -> (w669:T1)
          }
          frame 1 {
            n403 = Empty Array?(array=w960) -> (empty?=w961:bool)
            n404 = Empty Array?(array=w968) -> (empty?=w969:bool)
            n405 = Reciprocal(x=w970) -> (1/x=w959:dbl)
            n406 = Empty Array?(array=w971) -> (empty?=w972:bool)
            n407 = case shown="False" w972 {
              tunnel: w971 -> [w1123 w1250]
              tunnel: w959 -> [w1124 _]
              tunnel: [w1122 w1250] -> w967
              tunnel: w957 -> [w1121 _]
              frame False {
                n408 = for {
                  tunnel: w1123 -> [w1137] mode=indexing
                  tunnel: w1124 -> [_]
                  tunnel: w1123 -> [w1135] mode=indexing
                  tunnel: [w1127] -> w1122 mode=indexing
                  tunnel: w1121 -> [w1125]
                  n409 = Unbundle By Name(w1137) -> ("x"=w1126:sgl, "y"=w1129:sgl, "orientation"=w1128:sgl, "robot_id"=w1136:u32)
                  n410 = case shown="2" w1136 {
                    tunnel: w1126 -> [w1140 w1147 w1154 w1161 w1168 w1175 w1182 w1189 w1196 w1203 w1210 w1217 w1224 w1231 w1238 w1245]
                    tunnel: [w1142 w1149 w1156 w1163 w1170 w1177 w1184 w1191 w1198 w1205 w1212 w1219 w1226 w1233 w1240 w1247] -> w1134
                    tunnel: [w1144 w1151 w1158 w1165 w1172 w1179 w1186 w1193 w1200 w1207 w1214 w1221 w1228 w1235 w1242 w1249] -> w1133
                    tunnel: [w1143 w1150 w1157 w1164 w1171 w1178 w1185 w1192 w1199 w1206 w1213 w1220 w1227 w1234 w1241 w1248] -> w1132
                    tunnel: w1129 -> [w1139 w1146 w1153 w1160 w1167 w1174 w1181 w1188 w1195 w1202 w1209 w1216 w1223 w1230 w1237 w1244]
                    tunnel: w1128 -> [w1138 w1145 w1152 w1159 w1166 w1173 w1180 w1187 w1194 w1201 w1208 w1215 w1222 w1229 w1236 w1243]
                    tunnel: w1125 -> [w1141 w1148 w1155 w1162 w1169 w1176 w1183 w1190 w1197 w1204 w1211 w1218 w1225 w1232 w1239 w1246]
                    frame 0, Default {
                      n411 = call "2ndOrderDerivate.vi"("t_capture"=w1141, "initial condition"=w1140, "x"=w1140) -> ("dx/dt"=w1142:dbl)  [unwired: 5 in, 3 out]
                      n412 = call "2ndOrderDerivate.vi"("t_capture"=w1141, "initial condition"=w1139, "x"=w1139) -> ("dx/dt"=w1144:dbl)  [unwired: 5 in, 3 out]
                      n413 = call "2ndOrderDerivate.vi"("t_capture"=w1141, "initial condition"=w1138, "x"=w1138) -> ("dx/dt"=w1143:dbl)  [unwired: 5 in, 3 out]
                    }
                    frame 1 {
                      n414 = call "2ndOrderDerivate.vi"("t_capture"=w1148, "initial condition"=w1147, "x"=w1147) -> ("dx/dt"=w1149:dbl)  [unwired: 5 in, 3 out]
                      n415 = call "2ndOrderDerivate.vi"("t_capture"=w1148, "initial condition"=w1146, "x"=w1146) -> ("dx/dt"=w1151:dbl)  [unwired: 5 in, 3 out]
                      n416 = call "2ndOrderDerivate.vi"("t_capture"=w1148, "initial condition"=w1145, "x"=w1145) -> ("dx/dt"=w1150:dbl)  [unwired: 5 in, 3 out]
                    }
                    frame 2 {
                      n417 = call "2ndOrderDerivate.vi"("t_capture"=w1155, "initial condition"=w1154, "x"=w1154) -> ("dx/dt"=w1156:dbl)  [unwired: 5 in, 3 out]
                      n418 = call "2ndOrderDerivate.vi"("t_capture"=w1155, "initial condition"=w1153, "x"=w1153) -> ("dx/dt"=w1158:dbl)  [unwired: 5 in, 3 out]
                      n419 = call "2ndOrderDerivate.vi"("t_capture"=w1155, "initial condition"=w1152, "x"=w1152) -> ("dx/dt"=w1157:dbl)  [unwired: 5 in, 3 out]
                    }
                    frame 3 {
                      n420 = call "2ndOrderDerivate.vi"("t_capture"=w1162, "initial condition"=w1161, "x"=w1161) -> ("dx/dt"=w1163:dbl)  [unwired: 5 in, 3 out]
                      n421 = call "2ndOrderDerivate.vi"("t_capture"=w1162, "initial condition"=w1160, "x"=w1160) -> ("dx/dt"=w1165:dbl)  [unwired: 5 in, 3 out]
                      n422 = call "2ndOrderDerivate.vi"("t_capture"=w1162, "initial condition"=w1159, "x"=w1159) -> ("dx/dt"=w1164:dbl)  [unwired: 5 in, 3 out]
                    }
                    frame 4 {
                      n423 = call "2ndOrderDerivate.vi"("t_capture"=w1169, "initial condition"=w1168, "x"=w1168) -> ("dx/dt"=w1170:dbl)  [unwired: 5 in, 3 out]
                      n424 = call "2ndOrderDerivate.vi"("t_capture"=w1169, "initial condition"=w1167, "x"=w1167) -> ("dx/dt"=w1172:dbl)  [unwired: 5 in, 3 out]
                      n425 = call "2ndOrderDerivate.vi"("t_capture"=w1169, "initial condition"=w1166, "x"=w1166) -> ("dx/dt"=w1171:dbl)  [unwired: 5 in, 3 out]
                    }
                    frame 5 {
                      n426 = call "2ndOrderDerivate.vi"("t_capture"=w1176, "initial condition"=w1175, "x"=w1175) -> ("dx/dt"=w1177:dbl)  [unwired: 5 in, 3 out]
                      n427 = call "2ndOrderDerivate.vi"("t_capture"=w1176, "initial condition"=w1174, "x"=w1174) -> ("dx/dt"=w1179:dbl)  [unwired: 5 in, 3 out]
                      n428 = call "2ndOrderDerivate.vi"("t_capture"=w1176, "initial condition"=w1173, "x"=w1173) -> ("dx/dt"=w1178:dbl)  [unwired: 5 in, 3 out]
                    }
                    frame 6 {
                      n429 = call "2ndOrderDerivate.vi"("t_capture"=w1183, "initial condition"=w1182, "x"=w1182) -> ("dx/dt"=w1184:dbl)  [unwired: 5 in, 3 out]
                      n430 = call "2ndOrderDerivate.vi"("t_capture"=w1183, "initial condition"=w1181, "x"=w1181) -> ("dx/dt"=w1186:dbl)  [unwired: 5 in, 3 out]
                      n431 = call "2ndOrderDerivate.vi"("t_capture"=w1183, "initial condition"=w1180, "x"=w1180) -> ("dx/dt"=w1185:dbl)  [unwired: 5 in, 3 out]
                    }
                    frame 7 {
                      n432 = call "2ndOrderDerivate.vi"("t_capture"=w1190, "initial condition"=w1189, "x"=w1189) -> ("dx/dt"=w1191:dbl)  [unwired: 5 in, 3 out]
                      n433 = call "2ndOrderDerivate.vi"("t_capture"=w1190, "initial condition"=w1188, "x"=w1188) -> ("dx/dt"=w1193:dbl)  [unwired: 5 in, 3 out]
                      n434 = call "2ndOrderDerivate.vi"("t_capture"=w1190, "initial condition"=w1187, "x"=w1187) -> ("dx/dt"=w1192:dbl)  [unwired: 5 in, 3 out]
                    }
                    frame 8 {
                      n435 = call "2ndOrderDerivate.vi"("t_capture"=w1197, "initial condition"=w1196, "x"=w1196) -> ("dx/dt"=w1198:dbl)  [unwired: 5 in, 3 out]
                      n436 = call "2ndOrderDerivate.vi"("t_capture"=w1197, "initial condition"=w1195, "x"=w1195) -> ("dx/dt"=w1200:dbl)  [unwired: 5 in, 3 out]
                      n437 = call "2ndOrderDerivate.vi"("t_capture"=w1197, "initial condition"=w1194, "x"=w1194) -> ("dx/dt"=w1199:dbl)  [unwired: 5 in, 3 out]
                    }
                    frame 9 {
                      n438 = call "2ndOrderDerivate.vi"("t_capture"=w1204, "initial condition"=w1203, "x"=w1203) -> ("dx/dt"=w1205:dbl)  [unwired: 5 in, 3 out]
                      n439 = call "2ndOrderDerivate.vi"("t_capture"=w1204, "initial condition"=w1202, "x"=w1202) -> ("dx/dt"=w1207:dbl)  [unwired: 5 in, 3 out]
                      n440 = call "2ndOrderDerivate.vi"("t_capture"=w1204, "initial condition"=w1201, "x"=w1201) -> ("dx/dt"=w1206:dbl)  [unwired: 5 in, 3 out]
                    }
                    frame 10 {
                      n441 = call "2ndOrderDerivate.vi"("t_capture"=w1211, "initial condition"=w1210, "x"=w1210) -> ("dx/dt"=w1212:dbl)  [unwired: 5 in, 3 out]
                      n442 = call "2ndOrderDerivate.vi"("t_capture"=w1211, "initial condition"=w1209, "x"=w1209) -> ("dx/dt"=w1214:dbl)  [unwired: 5 in, 3 out]
                      n443 = call "2ndOrderDerivate.vi"("t_capture"=w1211, "initial condition"=w1208, "x"=w1208) -> ("dx/dt"=w1213:dbl)  [unwired: 5 in, 3 out]
                    }
                    frame 11 {
                      n444 = call "2ndOrderDerivate.vi"("t_capture"=w1218, "initial condition"=w1217, "x"=w1217) -> ("dx/dt"=w1219:dbl)  [unwired: 5 in, 3 out]
                      n445 = call "2ndOrderDerivate.vi"("t_capture"=w1218, "initial condition"=w1216, "x"=w1216) -> ("dx/dt"=w1221:dbl)  [unwired: 5 in, 3 out]
                      n446 = call "2ndOrderDerivate.vi"("t_capture"=w1218, "initial condition"=w1215, "x"=w1215) -> ("dx/dt"=w1220:dbl)  [unwired: 5 in, 3 out]
                    }
                    frame 12 {
                      n447 = call "2ndOrderDerivate.vi"("t_capture"=w1225, "initial condition"=w1224, "x"=w1224) -> ("dx/dt"=w1226:dbl)  [unwired: 5 in, 3 out]
                      n448 = call "2ndOrderDerivate.vi"("t_capture"=w1225, "initial condition"=w1223, "x"=w1223) -> ("dx/dt"=w1228:dbl)  [unwired: 5 in, 3 out]
                      n449 = call "2ndOrderDerivate.vi"("t_capture"=w1225, "initial condition"=w1222, "x"=w1222) -> ("dx/dt"=w1227:dbl)  [unwired: 5 in, 3 out]
                    }
                    frame 13 {
                      n450 = call "2ndOrderDerivate.vi"("t_capture"=w1232, "initial condition"=w1231, "x"=w1231) -> ("dx/dt"=w1233:dbl)  [unwired: 5 in, 3 out]
                      n451 = call "2ndOrderDerivate.vi"("t_capture"=w1232, "initial condition"=w1230, "x"=w1230) -> ("dx/dt"=w1235:dbl)  [unwired: 5 in, 3 out]
                      n452 = call "2ndOrderDerivate.vi"("t_capture"=w1232, "initial condition"=w1229, "x"=w1229) -> ("dx/dt"=w1234:dbl)  [unwired: 5 in, 3 out]
                    }
                    frame 14 {
                      n453 = call "2ndOrderDerivate.vi"("t_capture"=w1239, "initial condition"=w1238, "x"=w1238) -> ("dx/dt"=w1240:dbl)  [unwired: 5 in, 3 out]
                      n454 = call "2ndOrderDerivate.vi"("t_capture"=w1239, "initial condition"=w1237, "x"=w1237) -> ("dx/dt"=w1242:dbl)  [unwired: 5 in, 3 out]
                      n455 = call "2ndOrderDerivate.vi"("t_capture"=w1239, "initial condition"=w1236, "x"=w1236) -> ("dx/dt"=w1241:dbl)  [unwired: 5 in, 3 out]
                    }
                    frame 15 {
                      n456 = call "2ndOrderDerivate.vi"("t_capture"=w1246, "initial condition"=w1245, "x"=w1245) -> ("dx/dt"=w1247:dbl)  [unwired: 5 in, 3 out]
                      n457 = call "2ndOrderDerivate.vi"("t_capture"=w1246, "initial condition"=w1244, "x"=w1244) -> ("dx/dt"=w1249:dbl)  [unwired: 5 in, 3 out]
                      n458 = call "2ndOrderDerivate.vi"("t_capture"=w1246, "initial condition"=w1243, "x"=w1243) -> ("dx/dt"=w1248:dbl)  [unwired: 5 in, 3 out]
                    }
                  }
                  n459 = Build Array(w1126, w1134, w1129, w1133, w1128, w1132) -> (w1131:dbl[])
                  n460 = call-poly <vilib>:"Array To Matrix.vi"("Real 1D Array"=w1131) -> ("Real Matrix (Column Vector)"=w1130:T3)
                  n461 = Bundle By Name(cluster=w1135, "x_k|k"=w1130) -> (w1127:T2)
                }
              }
              frame True {
              }
            }
            n462 = case shown="False" w961 {
              tunnel: w960 -> [w975 w989]
              tunnel: w959 -> [w976 _]
              tunnel: [w974 w989] -> w958
              tunnel: w957 -> [w973 _]
              frame False {
                n463 = for {
                  tunnel: w975 -> [w988] mode=indexing
                  tunnel: w976 -> [_]
                  tunnel: w975 -> [w987] mode=indexing
                  tunnel: [w984] -> w974 mode=indexing
                  tunnel: w973 -> [w982]
                  n464 = Unbundle By Name(w988) -> ("x"=w983:sgl, "y"=w981:sgl, "z"=w977:sgl)
                  n465 = call "2ndOrderDerivate.vi"("t_capture"=w982, "initial condition"=w981, "x"=w981) -> ("dx/dt"=w979:dbl)  [unwired: 5 in, 3 out]
                  n466 = call "2ndOrderDerivate.vi"("t_capture"=w982, "initial condition"=w983, "x"=w983) -> ("dx/dt"=w980:dbl)  [unwired: 5 in, 3 out]
                  n467 = call "2ndOrderDerivate.vi"("t_capture"=w982, "initial condition"=w977, "x"=w977) -> ("dx/dt"=w978:dbl)  [unwired: 5 in, 3 out]
                  n468 = Build Array(w983, w980, w981, w979, w977, w978) -> (w986:dbl[])
                  n469 = call-poly <vilib>:"Array To Matrix.vi"("Real 1D Array"=w986) -> ("Real Matrix (Column Vector)"=w985:T3)
                  n470 = Bundle By Name(cluster=w987, "x_k|k"=w985) -> (w984:T4)
                }
              }
              frame True {
              }
            }
            n471 = case shown="False" w969 {
              tunnel: w968 -> [w992 w1120]
              tunnel: w959 -> [w993 _]
              tunnel: [w991 w1120] -> w966
              tunnel: w957 -> [w990 _]
              frame False {
                n472 = for {
                  tunnel: w992 -> [w1007] mode=indexing
                  tunnel: w993 -> [w995]
                  tunnel: w992 -> [w1005] mode=indexing
                  tunnel: [w996] -> w991 mode=indexing
                  tunnel: w990 -> [w994]
                  n473 = Unbundle By Name(w1007) -> ("x"=w1000:sgl, "y"=w999:sgl, "orientation"=w1001:sgl, "robot_id"=w1006:u32)
                  n474 = case shown="1" w1006 {
                    tunnel: w1000 -> [w1014 w1021 w1028 w1035 w1042 w1049 w1056 w1063 w1070 w1077 w1084 w1091 w1098 w1105 w1112 w1119]
                    tunnel: w999 -> [w1012 w1019 w1026 w1033 w1040 w1047 w1054 w1061 w1068 w1075 w1082 w1089 w1096 w1103 w1110 w1117]
                    tunnel: w1001 -> [w1011 w1018 w1025 w1032 w1039 w1046 w1053 w1060 w1067 w1074 w1081 w1088 w1095 w1102 w1109 w1116]
                    tunnel: [w1010 w1017 w1024 w1031 w1038 w1045 w1052 w1059 w1066 w1073 w1080 w1087 w1094 w1101 w1108 w1115] -> w1004
                    tunnel: [w1009 w1016 w1023 w1030 w1037 w1044 w1051 w1058 w1065 w1072 w1079 w1086 w1093 w1100 w1107 w1114] -> w1003
                    tunnel: [w1008 w1015 w1022 w1029 w1036 w1043 w1050 w1057 w1064 w1071 w1078 w1085 w1092 w1099 w1106 w1113] -> w1002
                    tunnel: w995 -> [_ _ _ _ _ _ _ _ _ _ _ _ _ _ _ _]
                    tunnel: w994 -> [w1013 w1020 w1027 w1034 w1041 w1048 w1055 w1062 w1069 w1076 w1083 w1090 w1097 w1104 w1111 w1118]
                    frame 0, Default {
                      n475 = call "2ndOrderDerivate.vi"("t_capture"=w1013, "initial condition"=w1014, "x"=w1014) -> ("dx/dt"=w1010:dbl)  [unwired: 5 in, 3 out]
                      n476 = call "2ndOrderDerivate.vi"("t_capture"=w1013, "initial condition"=w1012, "x"=w1012) -> ("dx/dt"=w1009:dbl)  [unwired: 5 in, 3 out]
                      n477 = call "2ndOrderDerivate.vi"("t_capture"=w1013, "initial condition"=w1011, "x"=w1011) -> ("dx/dt"=w1008:dbl)  [unwired: 5 in, 3 out]
                    }
                    frame 1 {
                      n478 = call "2ndOrderDerivate.vi"("t_capture"=w1020, "initial condition"=w1021, "x"=w1021) -> ("dx/dt"=w1017:dbl)  [unwired: 5 in, 3 out]
                      n479 = call "2ndOrderDerivate.vi"("t_capture"=w1020, "initial condition"=w1019, "x"=w1019) -> ("dx/dt"=w1016:dbl)  [unwired: 5 in, 3 out]
                      n480 = call "2ndOrderDerivate.vi"("t_capture"=w1020, "initial condition"=w1018, "x"=w1018) -> ("dx/dt"=w1015:dbl)  [unwired: 5 in, 3 out]
                    }
                    frame 2 {
                      n481 = call "2ndOrderDerivate.vi"("t_capture"=w1027, "initial condition"=w1028, "x"=w1028) -> ("dx/dt"=w1024:dbl)  [unwired: 5 in, 3 out]
                      n482 = call "2ndOrderDerivate.vi"("t_capture"=w1027, "initial condition"=w1026, "x"=w1026) -> ("dx/dt"=w1023:dbl)  [unwired: 5 in, 3 out]
                      n483 = call "2ndOrderDerivate.vi"("t_capture"=w1027, "initial condition"=w1025, "x"=w1025) -> ("dx/dt"=w1022:dbl)  [unwired: 5 in, 3 out]
                    }
                    frame 3 {
                      n484 = call "2ndOrderDerivate.vi"("t_capture"=w1034, "initial condition"=w1035, "x"=w1035) -> ("dx/dt"=w1031:dbl)  [unwired: 5 in, 3 out]
                      n485 = call "2ndOrderDerivate.vi"("t_capture"=w1034, "initial condition"=w1033, "x"=w1033) -> ("dx/dt"=w1030:dbl)  [unwired: 5 in, 3 out]
                      n486 = call "2ndOrderDerivate.vi"("t_capture"=w1034, "initial condition"=w1032, "x"=w1032) -> ("dx/dt"=w1029:dbl)  [unwired: 5 in, 3 out]
                    }
                    frame 4 {
                      n487 = call "2ndOrderDerivate.vi"("t_capture"=w1041, "initial condition"=w1042, "x"=w1042) -> ("dx/dt"=w1038:dbl)  [unwired: 5 in, 3 out]
                      n488 = call "2ndOrderDerivate.vi"("t_capture"=w1041, "initial condition"=w1040, "x"=w1040) -> ("dx/dt"=w1037:dbl)  [unwired: 5 in, 3 out]
                      n489 = call "2ndOrderDerivate.vi"("t_capture"=w1041, "initial condition"=w1039, "x"=w1039) -> ("dx/dt"=w1036:dbl)  [unwired: 5 in, 3 out]
                    }
                    frame 5 {
                      n490 = call "2ndOrderDerivate.vi"("t_capture"=w1048, "initial condition"=w1049, "x"=w1049) -> ("dx/dt"=w1045:dbl)  [unwired: 5 in, 3 out]
                      n491 = call "2ndOrderDerivate.vi"("t_capture"=w1048, "initial condition"=w1047, "x"=w1047) -> ("dx/dt"=w1044:dbl)  [unwired: 5 in, 3 out]
                      n492 = call "2ndOrderDerivate.vi"("t_capture"=w1048, "initial condition"=w1046, "x"=w1046) -> ("dx/dt"=w1043:dbl)  [unwired: 5 in, 3 out]
                    }
                    frame 6 {
                      n493 = call "2ndOrderDerivate.vi"("t_capture"=w1055, "initial condition"=w1056, "x"=w1056) -> ("dx/dt"=w1052:dbl)  [unwired: 5 in, 3 out]
                      n494 = call "2ndOrderDerivate.vi"("t_capture"=w1055, "initial condition"=w1054, "x"=w1054) -> ("dx/dt"=w1051:dbl)  [unwired: 5 in, 3 out]
                      n495 = call "2ndOrderDerivate.vi"("t_capture"=w1055, "initial condition"=w1053, "x"=w1053) -> ("dx/dt"=w1050:dbl)  [unwired: 5 in, 3 out]
                    }
                    frame 7 {
                      n496 = call "2ndOrderDerivate.vi"("t_capture"=w1062, "initial condition"=w1063, "x"=w1063) -> ("dx/dt"=w1059:dbl)  [unwired: 5 in, 3 out]
                      n497 = call "2ndOrderDerivate.vi"("t_capture"=w1062, "initial condition"=w1061, "x"=w1061) -> ("dx/dt"=w1058:dbl)  [unwired: 5 in, 3 out]
                      n498 = call "2ndOrderDerivate.vi"("t_capture"=w1062, "initial condition"=w1060, "x"=w1060) -> ("dx/dt"=w1057:dbl)  [unwired: 5 in, 3 out]
                    }
                    frame 8 {
                      n499 = call "2ndOrderDerivate.vi"("t_capture"=w1069, "initial condition"=w1070, "x"=w1070) -> ("dx/dt"=w1066:dbl)  [unwired: 5 in, 3 out]
                      n500 = call "2ndOrderDerivate.vi"("t_capture"=w1069, "initial condition"=w1068, "x"=w1068) -> ("dx/dt"=w1065:dbl)  [unwired: 5 in, 3 out]
                      n501 = call "2ndOrderDerivate.vi"("t_capture"=w1069, "initial condition"=w1067, "x"=w1067) -> ("dx/dt"=w1064:dbl)  [unwired: 5 in, 3 out]
                    }
                    frame 9 {
                      n502 = call "2ndOrderDerivate.vi"("t_capture"=w1076, "initial condition"=w1077, "x"=w1077) -> ("dx/dt"=w1073:dbl)  [unwired: 5 in, 3 out]
                      n503 = call "2ndOrderDerivate.vi"("t_capture"=w1076, "initial condition"=w1075, "x"=w1075) -> ("dx/dt"=w1072:dbl)  [unwired: 5 in, 3 out]
                      n504 = call "2ndOrderDerivate.vi"("t_capture"=w1076, "initial condition"=w1074, "x"=w1074) -> ("dx/dt"=w1071:dbl)  [unwired: 5 in, 3 out]
                    }
                    frame 10 {
                      n505 = call "2ndOrderDerivate.vi"("t_capture"=w1083, "initial condition"=w1084, "x"=w1084) -> ("dx/dt"=w1080:dbl)  [unwired: 5 in, 3 out]
                      n506 = call "2ndOrderDerivate.vi"("t_capture"=w1083, "initial condition"=w1082, "x"=w1082) -> ("dx/dt"=w1079:dbl)  [unwired: 5 in, 3 out]
                      n507 = call "2ndOrderDerivate.vi"("t_capture"=w1083, "initial condition"=w1081, "x"=w1081) -> ("dx/dt"=w1078:dbl)  [unwired: 5 in, 3 out]
                    }
                    frame 11 {
                      n508 = call "2ndOrderDerivate.vi"("t_capture"=w1090, "initial condition"=w1091, "x"=w1091) -> ("dx/dt"=w1087:dbl)  [unwired: 5 in, 3 out]
                      n509 = call "2ndOrderDerivate.vi"("t_capture"=w1090, "initial condition"=w1089, "x"=w1089) -> ("dx/dt"=w1086:dbl)  [unwired: 5 in, 3 out]
                      n510 = call "2ndOrderDerivate.vi"("t_capture"=w1090, "initial condition"=w1088, "x"=w1088) -> ("dx/dt"=w1085:dbl)  [unwired: 5 in, 3 out]
                    }
                    frame 12 {
                      n511 = call "2ndOrderDerivate.vi"("t_capture"=w1097, "initial condition"=w1098, "x"=w1098) -> ("dx/dt"=w1094:dbl)  [unwired: 5 in, 3 out]
                      n512 = call "2ndOrderDerivate.vi"("t_capture"=w1097, "initial condition"=w1096, "x"=w1096) -> ("dx/dt"=w1093:dbl)  [unwired: 5 in, 3 out]
                      n513 = call "2ndOrderDerivate.vi"("t_capture"=w1097, "initial condition"=w1095, "x"=w1095) -> ("dx/dt"=w1092:dbl)  [unwired: 5 in, 3 out]
                    }
                    frame 13 {
                      n514 = call "2ndOrderDerivate.vi"("t_capture"=w1104, "initial condition"=w1105, "x"=w1105) -> ("dx/dt"=w1101:dbl)  [unwired: 5 in, 3 out]
                      n515 = call "2ndOrderDerivate.vi"("t_capture"=w1104, "initial condition"=w1103, "x"=w1103) -> ("dx/dt"=w1100:dbl)  [unwired: 5 in, 3 out]
                      n516 = call "2ndOrderDerivate.vi"("t_capture"=w1104, "initial condition"=w1102, "x"=w1102) -> ("dx/dt"=w1099:dbl)  [unwired: 5 in, 3 out]
                    }
                    frame 14 {
                      n517 = call "2ndOrderDerivate.vi"("t_capture"=w1111, "initial condition"=w1112, "x"=w1112) -> ("dx/dt"=w1108:dbl)  [unwired: 5 in, 3 out]
                      n518 = call "2ndOrderDerivate.vi"("t_capture"=w1111, "initial condition"=w1110, "x"=w1110) -> ("dx/dt"=w1107:dbl)  [unwired: 5 in, 3 out]
                      n519 = call "2ndOrderDerivate.vi"("t_capture"=w1111, "initial condition"=w1109, "x"=w1109) -> ("dx/dt"=w1106:dbl)  [unwired: 5 in, 3 out]
                    }
                    frame 15 {
                      n520 = call "2ndOrderDerivate.vi"("t_capture"=w1118, "initial condition"=w1119, "x"=w1119) -> ("dx/dt"=w1115:dbl)  [unwired: 5 in, 3 out]
                      n521 = call "2ndOrderDerivate.vi"("t_capture"=w1118, "initial condition"=w1117, "x"=w1117) -> ("dx/dt"=w1114:dbl)  [unwired: 5 in, 3 out]
                      n522 = call "2ndOrderDerivate.vi"("t_capture"=w1118, "initial condition"=w1116, "x"=w1116) -> ("dx/dt"=w1113:dbl)  [unwired: 5 in, 3 out]
                    }
                  }
                  n523 = Build Array(w1000, w1004, w999, w1003, w1001, w1002) -> (w998:dbl[])
                  n524 = call-poly <vilib>:"Array To Matrix.vi"("Real 1D Array"=w998) -> ("Real Matrix (Column Vector)"=w997:T3)
                  n525 = Bundle By Name(cluster=w1005, "x_k|k"=w997) -> (w996:T2)
                }
              }
              frame True {
              }
            }
            n526 = Bundle By Name(cluster=w962, "robots_blue"=w967, "robots_yellow"=w966, "balls"=w958) -> (w965:T1)
            n527 = Bundle By Name(cluster=w962, "New"=FALSE) -> (w963:T1)
          }
          frame 2 {
            n528 = Empty Array?(array=w1254) -> (empty?=w1255:bool)
            n529 = Empty Array?(array=w1262) -> (empty?=w1263:bool)
            n530 = Reciprocal(x=w1264) -> (1/x=w1253:dbl)
            n531 = Empty Array?(array=w1265) -> (empty?=w1266:bool)
            n532 = case shown="False" w1266 {
              tunnel: w1265 -> [w1417 w1544]
              tunnel: w1253 -> [w1418 _]
              tunnel: [w1416 w1544] -> w1261
              tunnel: w1251 -> [w1415 _]
              frame False {
                n533 = for {
                  tunnel: w1417 -> [w1431] mode=indexing
                  tunnel: w1418 -> [_]
                  tunnel: w1417 -> [w1429] mode=indexing
                  tunnel: [w1421] -> w1416 mode=indexing
                  tunnel: w1415 -> [w1419]
                  n534 = Unbundle By Name(w1431) -> ("x"=w1420:sgl, "y"=w1423:sgl, "orientation"=w1422:sgl, "robot_id"=w1430:u32)
                  n535 = case shown="2" w1430 {
                    tunnel: w1420 -> [w1434 w1441 w1448 w1455 w1462 w1469 w1476 w1483 w1490 w1497 w1504 w1511 w1518 w1525 w1532 w1539]
                    tunnel: [w1436 w1443 w1450 w1457 w1464 w1471 w1478 w1485 w1492 w1499 w1506 w1513 w1520 w1527 w1534 w1541] -> w1428
                    tunnel: [w1438 w1445 w1452 w1459 w1466 w1473 w1480 w1487 w1494 w1501 w1508 w1515 w1522 w1529 w1536 w1543] -> w1427
                    tunnel: [w1437 w1444 w1451 w1458 w1465 w1472 w1479 w1486 w1493 w1500 w1507 w1514 w1521 w1528 w1535 w1542] -> w1426
                    tunnel: w1423 -> [w1433 w1440 w1447 w1454 w1461 w1468 w1475 w1482 w1489 w1496 w1503 w1510 w1517 w1524 w1531 w1538]
                    tunnel: w1422 -> [w1432 w1439 w1446 w1453 w1460 w1467 w1474 w1481 w1488 w1495 w1502 w1509 w1516 w1523 w1530 w1537]
                    tunnel: w1419 -> [w1435 w1442 w1449 w1456 w1463 w1470 w1477 w1484 w1491 w1498 w1505 w1512 w1519 w1526 w1533 w1540]
                    frame 0, Default {
                      n536 = call "2ndOrderDerivate.vi"("t_capture"=w1435, "initial condition"=w1434, "x"=w1434) -> ("dx/dt"=w1436:dbl)  [unwired: 5 in, 3 out]
                      n537 = call "2ndOrderDerivate.vi"("t_capture"=w1435, "initial condition"=w1433, "x"=w1433) -> ("dx/dt"=w1438:dbl)  [unwired: 5 in, 3 out]
                      n538 = call "2ndOrderDerivate.vi"("t_capture"=w1435, "initial condition"=w1432, "x"=w1432) -> ("dx/dt"=w1437:dbl)  [unwired: 5 in, 3 out]
                    }
                    frame 1 {
                      n539 = call "2ndOrderDerivate.vi"("t_capture"=w1442, "initial condition"=w1441, "x"=w1441) -> ("dx/dt"=w1443:dbl)  [unwired: 5 in, 3 out]
                      n540 = call "2ndOrderDerivate.vi"("t_capture"=w1442, "initial condition"=w1440, "x"=w1440) -> ("dx/dt"=w1445:dbl)  [unwired: 5 in, 3 out]
                      n541 = call "2ndOrderDerivate.vi"("t_capture"=w1442, "initial condition"=w1439, "x"=w1439) -> ("dx/dt"=w1444:dbl)  [unwired: 5 in, 3 out]
                    }
                    frame 2 {
                      n542 = call "2ndOrderDerivate.vi"("t_capture"=w1449, "initial condition"=w1448, "x"=w1448) -> ("dx/dt"=w1450:dbl)  [unwired: 5 in, 3 out]
                      n543 = call "2ndOrderDerivate.vi"("t_capture"=w1449, "initial condition"=w1447, "x"=w1447) -> ("dx/dt"=w1452:dbl)  [unwired: 5 in, 3 out]
                      n544 = call "2ndOrderDerivate.vi"("t_capture"=w1449, "initial condition"=w1446, "x"=w1446) -> ("dx/dt"=w1451:dbl)  [unwired: 5 in, 3 out]
                    }
                    frame 3 {
                      n545 = call "2ndOrderDerivate.vi"("t_capture"=w1456, "initial condition"=w1455, "x"=w1455) -> ("dx/dt"=w1457:dbl)  [unwired: 5 in, 3 out]
                      n546 = call "2ndOrderDerivate.vi"("t_capture"=w1456, "initial condition"=w1454, "x"=w1454) -> ("dx/dt"=w1459:dbl)  [unwired: 5 in, 3 out]
                      n547 = call "2ndOrderDerivate.vi"("t_capture"=w1456, "initial condition"=w1453, "x"=w1453) -> ("dx/dt"=w1458:dbl)  [unwired: 5 in, 3 out]
                    }
                    frame 4 {
                      n548 = call "2ndOrderDerivate.vi"("t_capture"=w1463, "initial condition"=w1462, "x"=w1462) -> ("dx/dt"=w1464:dbl)  [unwired: 5 in, 3 out]
                      n549 = call "2ndOrderDerivate.vi"("t_capture"=w1463, "initial condition"=w1461, "x"=w1461) -> ("dx/dt"=w1466:dbl)  [unwired: 5 in, 3 out]
                      n550 = call "2ndOrderDerivate.vi"("t_capture"=w1463, "initial condition"=w1460, "x"=w1460) -> ("dx/dt"=w1465:dbl)  [unwired: 5 in, 3 out]
                    }
                    frame 5 {
                      n551 = call "2ndOrderDerivate.vi"("t_capture"=w1470, "initial condition"=w1469, "x"=w1469) -> ("dx/dt"=w1471:dbl)  [unwired: 5 in, 3 out]
                      n552 = call "2ndOrderDerivate.vi"("t_capture"=w1470, "initial condition"=w1468, "x"=w1468) -> ("dx/dt"=w1473:dbl)  [unwired: 5 in, 3 out]
                      n553 = call "2ndOrderDerivate.vi"("t_capture"=w1470, "initial condition"=w1467, "x"=w1467) -> ("dx/dt"=w1472:dbl)  [unwired: 5 in, 3 out]
                    }
                    frame 6 {
                      n554 = call "2ndOrderDerivate.vi"("t_capture"=w1477, "initial condition"=w1476, "x"=w1476) -> ("dx/dt"=w1478:dbl)  [unwired: 5 in, 3 out]
                      n555 = call "2ndOrderDerivate.vi"("t_capture"=w1477, "initial condition"=w1475, "x"=w1475) -> ("dx/dt"=w1480:dbl)  [unwired: 5 in, 3 out]
                      n556 = call "2ndOrderDerivate.vi"("t_capture"=w1477, "initial condition"=w1474, "x"=w1474) -> ("dx/dt"=w1479:dbl)  [unwired: 5 in, 3 out]
                    }
                    frame 7 {
                      n557 = call "2ndOrderDerivate.vi"("t_capture"=w1484, "initial condition"=w1483, "x"=w1483) -> ("dx/dt"=w1485:dbl)  [unwired: 5 in, 3 out]
                      n558 = call "2ndOrderDerivate.vi"("t_capture"=w1484, "initial condition"=w1482, "x"=w1482) -> ("dx/dt"=w1487:dbl)  [unwired: 5 in, 3 out]
                      n559 = call "2ndOrderDerivate.vi"("t_capture"=w1484, "initial condition"=w1481, "x"=w1481) -> ("dx/dt"=w1486:dbl)  [unwired: 5 in, 3 out]
                    }
                    frame 8 {
                      n560 = call "2ndOrderDerivate.vi"("t_capture"=w1491, "initial condition"=w1490, "x"=w1490) -> ("dx/dt"=w1492:dbl)  [unwired: 5 in, 3 out]
                      n561 = call "2ndOrderDerivate.vi"("t_capture"=w1491, "initial condition"=w1489, "x"=w1489) -> ("dx/dt"=w1494:dbl)  [unwired: 5 in, 3 out]
                      n562 = call "2ndOrderDerivate.vi"("t_capture"=w1491, "initial condition"=w1488, "x"=w1488) -> ("dx/dt"=w1493:dbl)  [unwired: 5 in, 3 out]
                    }
                    frame 9 {
                      n563 = call "2ndOrderDerivate.vi"("t_capture"=w1498, "initial condition"=w1497, "x"=w1497) -> ("dx/dt"=w1499:dbl)  [unwired: 5 in, 3 out]
                      n564 = call "2ndOrderDerivate.vi"("t_capture"=w1498, "initial condition"=w1496, "x"=w1496) -> ("dx/dt"=w1501:dbl)  [unwired: 5 in, 3 out]
                      n565 = call "2ndOrderDerivate.vi"("t_capture"=w1498, "initial condition"=w1495, "x"=w1495) -> ("dx/dt"=w1500:dbl)  [unwired: 5 in, 3 out]
                    }
                    frame 10 {
                      n566 = call "2ndOrderDerivate.vi"("t_capture"=w1505, "initial condition"=w1504, "x"=w1504) -> ("dx/dt"=w1506:dbl)  [unwired: 5 in, 3 out]
                      n567 = call "2ndOrderDerivate.vi"("t_capture"=w1505, "initial condition"=w1503, "x"=w1503) -> ("dx/dt"=w1508:dbl)  [unwired: 5 in, 3 out]
                      n568 = call "2ndOrderDerivate.vi"("t_capture"=w1505, "initial condition"=w1502, "x"=w1502) -> ("dx/dt"=w1507:dbl)  [unwired: 5 in, 3 out]
                    }
                    frame 11 {
                      n569 = call "2ndOrderDerivate.vi"("t_capture"=w1512, "initial condition"=w1511, "x"=w1511) -> ("dx/dt"=w1513:dbl)  [unwired: 5 in, 3 out]
                      n570 = call "2ndOrderDerivate.vi"("t_capture"=w1512, "initial condition"=w1510, "x"=w1510) -> ("dx/dt"=w1515:dbl)  [unwired: 5 in, 3 out]
                      n571 = call "2ndOrderDerivate.vi"("t_capture"=w1512, "initial condition"=w1509, "x"=w1509) -> ("dx/dt"=w1514:dbl)  [unwired: 5 in, 3 out]
                    }
                    frame 12 {
                      n572 = call "2ndOrderDerivate.vi"("t_capture"=w1519, "initial condition"=w1518, "x"=w1518) -> ("dx/dt"=w1520:dbl)  [unwired: 5 in, 3 out]
                      n573 = call "2ndOrderDerivate.vi"("t_capture"=w1519, "initial condition"=w1517, "x"=w1517) -> ("dx/dt"=w1522:dbl)  [unwired: 5 in, 3 out]
                      n574 = call "2ndOrderDerivate.vi"("t_capture"=w1519, "initial condition"=w1516, "x"=w1516) -> ("dx/dt"=w1521:dbl)  [unwired: 5 in, 3 out]
                    }
                    frame 13 {
                      n575 = call "2ndOrderDerivate.vi"("t_capture"=w1526, "initial condition"=w1525, "x"=w1525) -> ("dx/dt"=w1527:dbl)  [unwired: 5 in, 3 out]
                      n576 = call "2ndOrderDerivate.vi"("t_capture"=w1526, "initial condition"=w1524, "x"=w1524) -> ("dx/dt"=w1529:dbl)  [unwired: 5 in, 3 out]
                      n577 = call "2ndOrderDerivate.vi"("t_capture"=w1526, "initial condition"=w1523, "x"=w1523) -> ("dx/dt"=w1528:dbl)  [unwired: 5 in, 3 out]
                    }
                    frame 14 {
                      n578 = call "2ndOrderDerivate.vi"("t_capture"=w1533, "initial condition"=w1532, "x"=w1532) -> ("dx/dt"=w1534:dbl)  [unwired: 5 in, 3 out]
                      n579 = call "2ndOrderDerivate.vi"("t_capture"=w1533, "initial condition"=w1531, "x"=w1531) -> ("dx/dt"=w1536:dbl)  [unwired: 5 in, 3 out]
                      n580 = call "2ndOrderDerivate.vi"("t_capture"=w1533, "initial condition"=w1530, "x"=w1530) -> ("dx/dt"=w1535:dbl)  [unwired: 5 in, 3 out]
                    }
                    frame 15 {
                      n581 = call "2ndOrderDerivate.vi"("t_capture"=w1540, "initial condition"=w1539, "x"=w1539) -> ("dx/dt"=w1541:dbl)  [unwired: 5 in, 3 out]
                      n582 = call "2ndOrderDerivate.vi"("t_capture"=w1540, "initial condition"=w1538, "x"=w1538) -> ("dx/dt"=w1543:dbl)  [unwired: 5 in, 3 out]
                      n583 = call "2ndOrderDerivate.vi"("t_capture"=w1540, "initial condition"=w1537, "x"=w1537) -> ("dx/dt"=w1542:dbl)  [unwired: 5 in, 3 out]
                    }
                  }
                  n584 = Build Array(w1420, w1428, w1423, w1427, w1422, w1426) -> (w1425:dbl[])
                  n585 = call-poly <vilib>:"Array To Matrix.vi"("Real 1D Array"=w1425) -> ("Real Matrix (Column Vector)"=w1424:T3)
                  n586 = Bundle By Name(cluster=w1429, "x_k|k"=w1424) -> (w1421:T2)
                }
              }
              frame True {
              }
            }
            n587 = case shown="False" w1255 {
              tunnel: w1254 -> [w1269 w1283]
              tunnel: w1253 -> [w1270 _]
              tunnel: [w1268 w1283] -> w1252
              tunnel: w1251 -> [w1267 _]
              frame False {
                n588 = for {
                  tunnel: w1269 -> [w1282] mode=indexing
                  tunnel: w1270 -> [_]
                  tunnel: w1269 -> [w1281] mode=indexing
                  tunnel: [w1278] -> w1268 mode=indexing
                  tunnel: w1267 -> [w1276]
                  n589 = Unbundle By Name(w1282) -> ("x"=w1277:sgl, "y"=w1275:sgl, "z"=w1271:sgl)
                  n590 = call "2ndOrderDerivate.vi"("t_capture"=w1276, "initial condition"=w1275, "x"=w1275) -> ("dx/dt"=w1273:dbl)  [unwired: 5 in, 3 out]
                  n591 = call "2ndOrderDerivate.vi"("t_capture"=w1276, "initial condition"=w1277, "x"=w1277) -> ("dx/dt"=w1274:dbl)  [unwired: 5 in, 3 out]
                  n592 = call "2ndOrderDerivate.vi"("t_capture"=w1276, "initial condition"=w1271, "x"=w1271) -> ("dx/dt"=w1272:dbl)  [unwired: 5 in, 3 out]
                  n593 = Build Array(w1277, w1274, w1275, w1273, w1271, w1272) -> (w1280:dbl[])
                  n594 = call-poly <vilib>:"Array To Matrix.vi"("Real 1D Array"=w1280) -> ("Real Matrix (Column Vector)"=w1279:T3)
                  n595 = Bundle By Name(cluster=w1281, "x_k|k"=w1279) -> (w1278:T4)
                }
              }
              frame True {
              }
            }
            n596 = case shown="False" w1263 {
              tunnel: w1262 -> [w1286 w1414]
              tunnel: w1253 -> [w1287 _]
              tunnel: [w1285 w1414] -> w1260
              tunnel: w1251 -> [w1284 _]
              frame False {
                n597 = for {
                  tunnel: w1286 -> [w1301] mode=indexing
                  tunnel: w1287 -> [w1289]
                  tunnel: w1286 -> [w1299] mode=indexing
                  tunnel: [w1290] -> w1285 mode=indexing
                  tunnel: w1284 -> [w1288]
                  n598 = Unbundle By Name(w1301) -> ("x"=w1294:sgl, "y"=w1293:sgl, "orientation"=w1295:sgl, "robot_id"=w1300:u32)
                  n599 = case shown="1" w1300 {
                    tunnel: w1294 -> [w1308 w1315 w1322 w1329 w1336 w1343 w1350 w1357 w1364 w1371 w1378 w1385 w1392 w1399 w1406 w1413]
                    tunnel: w1293 -> [w1306 w1313 w1320 w1327 w1334 w1341 w1348 w1355 w1362 w1369 w1376 w1383 w1390 w1397 w1404 w1411]
                    tunnel: w1295 -> [w1305 w1312 w1319 w1326 w1333 w1340 w1347 w1354 w1361 w1368 w1375 w1382 w1389 w1396 w1403 w1410]
                    tunnel: [w1304 w1311 w1318 w1325 w1332 w1339 w1346 w1353 w1360 w1367 w1374 w1381 w1388 w1395 w1402 w1409] -> w1298
                    tunnel: [w1303 w1310 w1317 w1324 w1331 w1338 w1345 w1352 w1359 w1366 w1373 w1380 w1387 w1394 w1401 w1408] -> w1297
                    tunnel: [w1302 w1309 w1316 w1323 w1330 w1337 w1344 w1351 w1358 w1365 w1372 w1379 w1386 w1393 w1400 w1407] -> w1296
                    tunnel: w1289 -> [_ _ _ _ _ _ _ _ _ _ _ _ _ _ _ _]
                    tunnel: w1288 -> [w1307 w1314 w1321 w1328 w1335 w1342 w1349 w1356 w1363 w1370 w1377 w1384 w1391 w1398 w1405 w1412]
                    frame 0, Default {
                      n600 = call "2ndOrderDerivate.vi"("t_capture"=w1307, "initial condition"=w1308, "x"=w1308) -> ("dx/dt"=w1304:dbl)  [unwired: 5 in, 3 out]
                      n601 = call "2ndOrderDerivate.vi"("t_capture"=w1307, "initial condition"=w1306, "x"=w1306) -> ("dx/dt"=w1303:dbl)  [unwired: 5 in, 3 out]
                      n602 = call "2ndOrderDerivate.vi"("t_capture"=w1307, "initial condition"=w1305, "x"=w1305) -> ("dx/dt"=w1302:dbl)  [unwired: 5 in, 3 out]
                    }
                    frame 1 {
                      n603 = call "2ndOrderDerivate.vi"("t_capture"=w1314, "initial condition"=w1315, "x"=w1315) -> ("dx/dt"=w1311:dbl)  [unwired: 5 in, 3 out]
                      n604 = call "2ndOrderDerivate.vi"("t_capture"=w1314, "initial condition"=w1313, "x"=w1313) -> ("dx/dt"=w1310:dbl)  [unwired: 5 in, 3 out]
                      n605 = call "2ndOrderDerivate.vi"("t_capture"=w1314, "initial condition"=w1312, "x"=w1312) -> ("dx/dt"=w1309:dbl)  [unwired: 5 in, 3 out]
                    }
                    frame 2 {
                      n606 = call "2ndOrderDerivate.vi"("t_capture"=w1321, "initial condition"=w1322, "x"=w1322) -> ("dx/dt"=w1318:dbl)  [unwired: 5 in, 3 out]
                      n607 = call "2ndOrderDerivate.vi"("t_capture"=w1321, "initial condition"=w1320, "x"=w1320) -> ("dx/dt"=w1317:dbl)  [unwired: 5 in, 3 out]
                      n608 = call "2ndOrderDerivate.vi"("t_capture"=w1321, "initial condition"=w1319, "x"=w1319) -> ("dx/dt"=w1316:dbl)  [unwired: 5 in, 3 out]
                    }
                    frame 3 {
                      n609 = call "2ndOrderDerivate.vi"("t_capture"=w1328, "initial condition"=w1329, "x"=w1329) -> ("dx/dt"=w1325:dbl)  [unwired: 5 in, 3 out]
                      n610 = call "2ndOrderDerivate.vi"("t_capture"=w1328, "initial condition"=w1327, "x"=w1327) -> ("dx/dt"=w1324:dbl)  [unwired: 5 in, 3 out]
                      n611 = call "2ndOrderDerivate.vi"("t_capture"=w1328, "initial condition"=w1326, "x"=w1326) -> ("dx/dt"=w1323:dbl)  [unwired: 5 in, 3 out]
                    }
                    frame 4 {
                      n612 = call "2ndOrderDerivate.vi"("t_capture"=w1335, "initial condition"=w1336, "x"=w1336) -> ("dx/dt"=w1332:dbl)  [unwired: 5 in, 3 out]
                      n613 = call "2ndOrderDerivate.vi"("t_capture"=w1335, "initial condition"=w1334, "x"=w1334) -> ("dx/dt"=w1331:dbl)  [unwired: 5 in, 3 out]
                      n614 = call "2ndOrderDerivate.vi"("t_capture"=w1335, "initial condition"=w1333, "x"=w1333) -> ("dx/dt"=w1330:dbl)  [unwired: 5 in, 3 out]
                    }
                    frame 5 {
                      n615 = call "2ndOrderDerivate.vi"("t_capture"=w1342, "initial condition"=w1343, "x"=w1343) -> ("dx/dt"=w1339:dbl)  [unwired: 5 in, 3 out]
                      n616 = call "2ndOrderDerivate.vi"("t_capture"=w1342, "initial condition"=w1341, "x"=w1341) -> ("dx/dt"=w1338:dbl)  [unwired: 5 in, 3 out]
                      n617 = call "2ndOrderDerivate.vi"("t_capture"=w1342, "initial condition"=w1340, "x"=w1340) -> ("dx/dt"=w1337:dbl)  [unwired: 5 in, 3 out]
                    }
                    frame 6 {
                      n618 = call "2ndOrderDerivate.vi"("t_capture"=w1349, "initial condition"=w1350, "x"=w1350) -> ("dx/dt"=w1346:dbl)  [unwired: 5 in, 3 out]
                      n619 = call "2ndOrderDerivate.vi"("t_capture"=w1349, "initial condition"=w1348, "x"=w1348) -> ("dx/dt"=w1345:dbl)  [unwired: 5 in, 3 out]
                      n620 = call "2ndOrderDerivate.vi"("t_capture"=w1349, "initial condition"=w1347, "x"=w1347) -> ("dx/dt"=w1344:dbl)  [unwired: 5 in, 3 out]
                    }
                    frame 7 {
                      n621 = call "2ndOrderDerivate.vi"("t_capture"=w1356, "initial condition"=w1357, "x"=w1357) -> ("dx/dt"=w1353:dbl)  [unwired: 5 in, 3 out]
                      n622 = call "2ndOrderDerivate.vi"("t_capture"=w1356, "initial condition"=w1355, "x"=w1355) -> ("dx/dt"=w1352:dbl)  [unwired: 5 in, 3 out]
                      n623 = call "2ndOrderDerivate.vi"("t_capture"=w1356, "initial condition"=w1354, "x"=w1354) -> ("dx/dt"=w1351:dbl)  [unwired: 5 in, 3 out]
                    }
                    frame 8 {
                      n624 = call "2ndOrderDerivate.vi"("t_capture"=w1363, "initial condition"=w1364, "x"=w1364) -> ("dx/dt"=w1360:dbl)  [unwired: 5 in, 3 out]
                      n625 = call "2ndOrderDerivate.vi"("t_capture"=w1363, "initial condition"=w1362, "x"=w1362) -> ("dx/dt"=w1359:dbl)  [unwired: 5 in, 3 out]
                      n626 = call "2ndOrderDerivate.vi"("t_capture"=w1363, "initial condition"=w1361, "x"=w1361) -> ("dx/dt"=w1358:dbl)  [unwired: 5 in, 3 out]
                    }
                    frame 9 {
                      n627 = call "2ndOrderDerivate.vi"("t_capture"=w1370, "initial condition"=w1371, "x"=w1371) -> ("dx/dt"=w1367:dbl)  [unwired: 5 in, 3 out]
                      n628 = call "2ndOrderDerivate.vi"("t_capture"=w1370, "initial condition"=w1369, "x"=w1369) -> ("dx/dt"=w1366:dbl)  [unwired: 5 in, 3 out]
                      n629 = call "2ndOrderDerivate.vi"("t_capture"=w1370, "initial condition"=w1368, "x"=w1368) -> ("dx/dt"=w1365:dbl)  [unwired: 5 in, 3 out]
                    }
                    frame 10 {
                      n630 = call "2ndOrderDerivate.vi"("t_capture"=w1377, "initial condition"=w1378, "x"=w1378) -> ("dx/dt"=w1374:dbl)  [unwired: 5 in, 3 out]
                      n631 = call "2ndOrderDerivate.vi"("t_capture"=w1377, "initial condition"=w1376, "x"=w1376) -> ("dx/dt"=w1373:dbl)  [unwired: 5 in, 3 out]
                      n632 = call "2ndOrderDerivate.vi"("t_capture"=w1377, "initial condition"=w1375, "x"=w1375) -> ("dx/dt"=w1372:dbl)  [unwired: 5 in, 3 out]
                    }
                    frame 11 {
                      n633 = call "2ndOrderDerivate.vi"("t_capture"=w1384, "initial condition"=w1385, "x"=w1385) -> ("dx/dt"=w1381:dbl)  [unwired: 5 in, 3 out]
                      n634 = call "2ndOrderDerivate.vi"("t_capture"=w1384, "initial condition"=w1383, "x"=w1383) -> ("dx/dt"=w1380:dbl)  [unwired: 5 in, 3 out]
                      n635 = call "2ndOrderDerivate.vi"("t_capture"=w1384, "initial condition"=w1382, "x"=w1382) -> ("dx/dt"=w1379:dbl)  [unwired: 5 in, 3 out]
                    }
                    frame 12 {
                      n636 = call "2ndOrderDerivate.vi"("t_capture"=w1391, "initial condition"=w1392, "x"=w1392) -> ("dx/dt"=w1388:dbl)  [unwired: 5 in, 3 out]
                      n637 = call "2ndOrderDerivate.vi"("t_capture"=w1391, "initial condition"=w1390, "x"=w1390) -> ("dx/dt"=w1387:dbl)  [unwired: 5 in, 3 out]
                      n638 = call "2ndOrderDerivate.vi"("t_capture"=w1391, "initial condition"=w1389, "x"=w1389) -> ("dx/dt"=w1386:dbl)  [unwired: 5 in, 3 out]
                    }
                    frame 13 {
                      n639 = call "2ndOrderDerivate.vi"("t_capture"=w1398, "initial condition"=w1399, "x"=w1399) -> ("dx/dt"=w1395:dbl)  [unwired: 5 in, 3 out]
                      n640 = call "2ndOrderDerivate.vi"("t_capture"=w1398, "initial condition"=w1397, "x"=w1397) -> ("dx/dt"=w1394:dbl)  [unwired: 5 in, 3 out]
                      n641 = call "2ndOrderDerivate.vi"("t_capture"=w1398, "initial condition"=w1396, "x"=w1396) -> ("dx/dt"=w1393:dbl)  [unwired: 5 in, 3 out]
                    }
                    frame 14 {
                      n642 = call "2ndOrderDerivate.vi"("t_capture"=w1405, "initial condition"=w1406, "x"=w1406) -> ("dx/dt"=w1402:dbl)  [unwired: 5 in, 3 out]
                      n643 = call "2ndOrderDerivate.vi"("t_capture"=w1405, "initial condition"=w1404, "x"=w1404) -> ("dx/dt"=w1401:dbl)  [unwired: 5 in, 3 out]
                      n644 = call "2ndOrderDerivate.vi"("t_capture"=w1405, "initial condition"=w1403, "x"=w1403) -> ("dx/dt"=w1400:dbl)  [unwired: 5 in, 3 out]
                    }
                    frame 15 {
                      n645 = call "2ndOrderDerivate.vi"("t_capture"=w1412, "initial condition"=w1413, "x"=w1413) -> ("dx/dt"=w1409:dbl)  [unwired: 5 in, 3 out]
                      n646 = call "2ndOrderDerivate.vi"("t_capture"=w1412, "initial condition"=w1411, "x"=w1411) -> ("dx/dt"=w1408:dbl)  [unwired: 5 in, 3 out]
                      n647 = call "2ndOrderDerivate.vi"("t_capture"=w1412, "initial condition"=w1410, "x"=w1410) -> ("dx/dt"=w1407:dbl)  [unwired: 5 in, 3 out]
                    }
                  }
                  n648 = Build Array(w1294, w1298, w1293, w1297, w1295, w1296) -> (w1292:dbl[])
                  n649 = call-poly <vilib>:"Array To Matrix.vi"("Real 1D Array"=w1292) -> ("Real Matrix (Column Vector)"=w1291:T3)
                  n650 = Bundle By Name(cluster=w1299, "x_k|k"=w1291) -> (w1290:T2)
                }
              }
              frame True {
              }
            }
            n651 = Bundle By Name(cluster=w1256, "robots_blue"=w1261, "robots_yellow"=w1260, "balls"=w1252) -> (w1259:T1)
            n652 = Bundle By Name(cluster=w1256, "New"=FALSE) -> (w1257:T1)
          }
          frame 3 {
            n653 = Empty Array?(array=w1548) -> (empty?=w1549:bool)
            n654 = Empty Array?(array=w1556) -> (empty?=w1557:bool)
            n655 = Reciprocal(x=w1558) -> (1/x=w1547:dbl)
            n656 = Empty Array?(array=w1559) -> (empty?=w1560:bool)
            n657 = case shown="False" w1560 {
              tunnel: w1559 -> [w1712 w1838]
              tunnel: w1547 -> [w1713 _]
              tunnel: [w1711 w1838] -> w1555
              tunnel: w1545 -> [w1710 _]
              frame False {
                n658 = for {
                  tunnel: w1712 -> [w1714] mode=indexing
                  tunnel: w1713 -> [_]
                  tunnel: [w1717] -> w1711 mode=indexing
                  tunnel: w1710 -> [w1715]
                  n659 = Unbundle By Name(w1714) -> ("x"=w1716:sgl, "y"=w1719:sgl, "orientation"=w1718:sgl, "robot_id"=w1725:u32)  [unwired: 1 out]
                  n660 = case shown="2" w1725 {
                    tunnel: w1716 -> [w1728 w1735 w1742 w1749 w1756 w1763 w1770 w1777 w1784 w1791 w1798 w1805 w1812 w1819 w1826 w1833]
                    tunnel: [w1730 w1737 w1744 w1751 w1758 w1765 w1772 w1779 w1786 w1793 w1800 w1807 w1814 w1821 w1828 w1835] -> w1724
                    tunnel: [w1732 w1739 w1746 w1753 w1760 w1767 w1774 w1781 w1788 w1795 w1802 w1809 w1816 w1823 w1830 w1837] -> w1723
                    tunnel: [w1731 w1738 w1745 w1752 w1759 w1766 w1773 w1780 w1787 w1794 w1801 w1808 w1815 w1822 w1829 w1836] -> w1722
                    tunnel: w1719 -> [w1727 w1734 w1741 w1748 w1755 w1762 w1769 w1776 w1783 w1790 w1797 w1804 w1811 w1818 w1825 w1832]
                    tunnel: w1718 -> [w1726 w1733 w1740 w1747 w1754 w1761 w1768 w1775 w1782 w1789 w1796 w1803 w1810 w1817 w1824 w1831]
                    tunnel: w1715 -> [w1729 w1736 w1743 w1750 w1757 w1764 w1771 w1778 w1785 w1792 w1799 w1806 w1813 w1820 w1827 w1834]
                    frame 0, Default {
                      n661 = call "2ndOrderDerivate.vi"("t_capture"=w1729, "initial condition"=w1728, "x"=w1728) -> ("dx/dt"=w1730:dbl)  [unwired: 5 in, 3 out]
                      n662 = call "2ndOrderDerivate.vi"("t_capture"=w1729, "initial condition"=w1727, "x"=w1727) -> ("dx/dt"=w1732:dbl)  [unwired: 5 in, 3 out]
                      n663 = call "2ndOrderDerivate.vi"("t_capture"=w1729, "initial condition"=w1726, "x"=w1726) -> ("dx/dt"=w1731:dbl)  [unwired: 5 in, 3 out]
                    }
                    frame 1 {
                      n664 = call "2ndOrderDerivate.vi"("t_capture"=w1736, "initial condition"=w1735, "x"=w1735) -> ("dx/dt"=w1737:dbl)  [unwired: 5 in, 3 out]
                      n665 = call "2ndOrderDerivate.vi"("t_capture"=w1736, "initial condition"=w1734, "x"=w1734) -> ("dx/dt"=w1739:dbl)  [unwired: 5 in, 3 out]
                      n666 = call "2ndOrderDerivate.vi"("t_capture"=w1736, "initial condition"=w1733, "x"=w1733) -> ("dx/dt"=w1738:dbl)  [unwired: 5 in, 3 out]
                    }
                    frame 2 {
                      n667 = call "2ndOrderDerivate.vi"("t_capture"=w1743, "initial condition"=w1742, "x"=w1742) -> ("dx/dt"=w1744:dbl)  [unwired: 5 in, 3 out]
                      n668 = call "2ndOrderDerivate.vi"("t_capture"=w1743, "initial condition"=w1741, "x"=w1741) -> ("dx/dt"=w1746:dbl)  [unwired: 5 in, 3 out]
                      n669 = call "2ndOrderDerivate.vi"("t_capture"=w1743, "initial condition"=w1740, "x"=w1740) -> ("dx/dt"=w1745:dbl)  [unwired: 5 in, 3 out]
                    }
                    frame 3 {
                      n670 = call "2ndOrderDerivate.vi"("t_capture"=w1750, "initial condition"=w1749, "x"=w1749) -> ("dx/dt"=w1751:dbl)  [unwired: 5 in, 3 out]
                      n671 = call "2ndOrderDerivate.vi"("t_capture"=w1750, "initial condition"=w1748, "x"=w1748) -> ("dx/dt"=w1753:dbl)  [unwired: 5 in, 3 out]
                      n672 = call "2ndOrderDerivate.vi"("t_capture"=w1750, "initial condition"=w1747, "x"=w1747) -> ("dx/dt"=w1752:dbl)  [unwired: 5 in, 3 out]
                    }
                    frame 4 {
                      n673 = call "2ndOrderDerivate.vi"("t_capture"=w1757, "initial condition"=w1756, "x"=w1756) -> ("dx/dt"=w1758:dbl)  [unwired: 5 in, 3 out]
                      n674 = call "2ndOrderDerivate.vi"("t_capture"=w1757, "initial condition"=w1755, "x"=w1755) -> ("dx/dt"=w1760:dbl)  [unwired: 5 in, 3 out]
                      n675 = call "2ndOrderDerivate.vi"("t_capture"=w1757, "initial condition"=w1754, "x"=w1754) -> ("dx/dt"=w1759:dbl)  [unwired: 5 in, 3 out]
                    }
                    frame 5 {
                      n676 = call "2ndOrderDerivate.vi"("t_capture"=w1764, "initial condition"=w1763, "x"=w1763) -> ("dx/dt"=w1765:dbl)  [unwired: 5 in, 3 out]
                      n677 = call "2ndOrderDerivate.vi"("t_capture"=w1764, "initial condition"=w1762, "x"=w1762) -> ("dx/dt"=w1767:dbl)  [unwired: 5 in, 3 out]
                      n678 = call "2ndOrderDerivate.vi"("t_capture"=w1764, "initial condition"=w1761, "x"=w1761) -> ("dx/dt"=w1766:dbl)  [unwired: 5 in, 3 out]
                    }
                    frame 6 {
                      n679 = call "2ndOrderDerivate.vi"("t_capture"=w1771, "initial condition"=w1770, "x"=w1770) -> ("dx/dt"=w1772:dbl)  [unwired: 5 in, 3 out]
                      n680 = call "2ndOrderDerivate.vi"("t_capture"=w1771, "initial condition"=w1769, "x"=w1769) -> ("dx/dt"=w1774:dbl)  [unwired: 5 in, 3 out]
                      n681 = call "2ndOrderDerivate.vi"("t_capture"=w1771, "initial condition"=w1768, "x"=w1768) -> ("dx/dt"=w1773:dbl)  [unwired: 5 in, 3 out]
                    }
                    frame 7 {
                      n682 = call "2ndOrderDerivate.vi"("t_capture"=w1778, "initial condition"=w1777, "x"=w1777) -> ("dx/dt"=w1779:dbl)  [unwired: 5 in, 3 out]
                      n683 = call "2ndOrderDerivate.vi"("t_capture"=w1778, "initial condition"=w1776, "x"=w1776) -> ("dx/dt"=w1781:dbl)  [unwired: 5 in, 3 out]
                      n684 = call "2ndOrderDerivate.vi"("t_capture"=w1778, "initial condition"=w1775, "x"=w1775) -> ("dx/dt"=w1780:dbl)  [unwired: 5 in, 3 out]
                    }
                    frame 8 {
                      n685 = call "2ndOrderDerivate.vi"("t_capture"=w1785, "initial condition"=w1784, "x"=w1784) -> ("dx/dt"=w1786:dbl)  [unwired: 5 in, 3 out]
                      n686 = call "2ndOrderDerivate.vi"("t_capture"=w1785, "initial condition"=w1783, "x"=w1783) -> ("dx/dt"=w1788:dbl)  [unwired: 5 in, 3 out]
                      n687 = call "2ndOrderDerivate.vi"("t_capture"=w1785, "initial condition"=w1782, "x"=w1782) -> ("dx/dt"=w1787:dbl)  [unwired: 5 in, 3 out]
                    }
                    frame 9 {
                      n688 = call "2ndOrderDerivate.vi"("t_capture"=w1792, "initial condition"=w1791, "x"=w1791) -> ("dx/dt"=w1793:dbl)  [unwired: 5 in, 3 out]
                      n689 = call "2ndOrderDerivate.vi"("t_capture"=w1792, "initial condition"=w1790, "x"=w1790) -> ("dx/dt"=w1795:dbl)  [unwired: 5 in, 3 out]
                      n690 = call "2ndOrderDerivate.vi"("t_capture"=w1792, "initial condition"=w1789, "x"=w1789) -> ("dx/dt"=w1794:dbl)  [unwired: 5 in, 3 out]
                    }
                    frame 10 {
                      n691 = call "2ndOrderDerivate.vi"("t_capture"=w1799, "initial condition"=w1798, "x"=w1798) -> ("dx/dt"=w1800:dbl)  [unwired: 5 in, 3 out]
                      n692 = call "2ndOrderDerivate.vi"("t_capture"=w1799, "initial condition"=w1797, "x"=w1797) -> ("dx/dt"=w1802:dbl)  [unwired: 5 in, 3 out]
                      n693 = call "2ndOrderDerivate.vi"("t_capture"=w1799, "initial condition"=w1796, "x"=w1796) -> ("dx/dt"=w1801:dbl)  [unwired: 5 in, 3 out]
                    }
                    frame 11 {
                      n694 = call "2ndOrderDerivate.vi"("t_capture"=w1806, "initial condition"=w1805, "x"=w1805) -> ("dx/dt"=w1807:dbl)  [unwired: 5 in, 3 out]
                      n695 = call "2ndOrderDerivate.vi"("t_capture"=w1806, "initial condition"=w1804, "x"=w1804) -> ("dx/dt"=w1809:dbl)  [unwired: 5 in, 3 out]
                      n696 = call "2ndOrderDerivate.vi"("t_capture"=w1806, "initial condition"=w1803, "x"=w1803) -> ("dx/dt"=w1808:dbl)  [unwired: 5 in, 3 out]
                    }
                    frame 12 {
                      n697 = call "2ndOrderDerivate.vi"("t_capture"=w1813, "initial condition"=w1812, "x"=w1812) -> ("dx/dt"=w1814:dbl)  [unwired: 5 in, 3 out]
                      n698 = call "2ndOrderDerivate.vi"("t_capture"=w1813, "initial condition"=w1811, "x"=w1811) -> ("dx/dt"=w1816:dbl)  [unwired: 5 in, 3 out]
                      n699 = call "2ndOrderDerivate.vi"("t_capture"=w1813, "initial condition"=w1810, "x"=w1810) -> ("dx/dt"=w1815:dbl)  [unwired: 5 in, 3 out]
                    }
                    frame 13 {
                      n700 = call "2ndOrderDerivate.vi"("t_capture"=w1820, "initial condition"=w1819, "x"=w1819) -> ("dx/dt"=w1821:dbl)  [unwired: 5 in, 3 out]
                      n701 = call "2ndOrderDerivate.vi"("t_capture"=w1820, "initial condition"=w1818, "x"=w1818) -> ("dx/dt"=w1823:dbl)  [unwired: 5 in, 3 out]
                      n702 = call "2ndOrderDerivate.vi"("t_capture"=w1820, "initial condition"=w1817, "x"=w1817) -> ("dx/dt"=w1822:dbl)  [unwired: 5 in, 3 out]
                    }
                    frame 14 {
                      n703 = call "2ndOrderDerivate.vi"("t_capture"=w1827, "initial condition"=w1826, "x"=w1826) -> ("dx/dt"=w1828:dbl)  [unwired: 5 in, 3 out]
                      n704 = call "2ndOrderDerivate.vi"("t_capture"=w1827, "initial condition"=w1825, "x"=w1825) -> ("dx/dt"=w1830:dbl)  [unwired: 5 in, 3 out]
                      n705 = call "2ndOrderDerivate.vi"("t_capture"=w1827, "initial condition"=w1824, "x"=w1824) -> ("dx/dt"=w1829:dbl)  [unwired: 5 in, 3 out]
                    }
                    frame 15 {
                      n706 = call "2ndOrderDerivate.vi"("t_capture"=w1834, "initial condition"=w1833, "x"=w1833) -> ("dx/dt"=w1835:dbl)  [unwired: 5 in, 3 out]
                      n707 = call "2ndOrderDerivate.vi"("t_capture"=w1834, "initial condition"=w1832, "x"=w1832) -> ("dx/dt"=w1837:dbl)  [unwired: 5 in, 3 out]
                      n708 = call "2ndOrderDerivate.vi"("t_capture"=w1834, "initial condition"=w1831, "x"=w1831) -> ("dx/dt"=w1836:dbl)  [unwired: 5 in, 3 out]
                    }
                  }
                  n709 = Build Array(w1716, w1724, w1719, w1723, w1718, w1722) -> (w1721:dbl[])
                  n710 = call-poly <vilib>:"Array To Matrix.vi"("Real 1D Array"=w1721) -> ("Real Matrix (Column Vector)"=w1720:T3)
                  n711 = Bundle By Name(cluster=w1714, "x_k|k"=w1720) -> (w1717:T2)
                }
              }
              frame True {
              }
            }
            n712 = case shown="False" w1549 {
              tunnel: w1548 -> [w1563 w1577]
              tunnel: w1547 -> [w1564 _]
              tunnel: [w1562 w1577] -> w1546
              tunnel: w1545 -> [w1561 _]
              frame False {
                n713 = for {
                  tunnel: w1563 -> [w1576] mode=indexing
                  tunnel: w1564 -> [_]
                  tunnel: w1563 -> [w1575] mode=indexing
                  tunnel: [w1572] -> w1562 mode=indexing
                  tunnel: w1561 -> [w1570]
                  n714 = Unbundle By Name(w1576) -> ("x"=w1571:sgl, "y"=w1569:sgl, "z"=w1565:sgl)
                  n715 = call "2ndOrderDerivate.vi"("t_capture"=w1570, "initial condition"=w1569, "x"=w1569) -> ("dx/dt"=w1567:dbl)  [unwired: 5 in, 3 out]
                  n716 = call "2ndOrderDerivate.vi"("t_capture"=w1570, "initial condition"=w1571, "x"=w1571) -> ("dx/dt"=w1568:dbl)  [unwired: 5 in, 3 out]
                  n717 = call "2ndOrderDerivate.vi"("t_capture"=w1570, "initial condition"=w1565, "x"=w1565) -> ("dx/dt"=w1566:dbl)  [unwired: 5 in, 3 out]
                  n718 = Build Array(w1571, w1568, w1569, w1567, w1565, w1566) -> (w1574:dbl[])
                  n719 = call-poly <vilib>:"Array To Matrix.vi"("Real 1D Array"=w1574) -> ("Real Matrix (Column Vector)"=w1573:T3)
                  n720 = Bundle By Name(cluster=w1575, "x_k|k"=w1573) -> (w1572:T4)
                }
              }
              frame True {
              }
            }
            n721 = case shown="False" w1557 {
              tunnel: w1556 -> [w1580 w1709]
              tunnel: w1547 -> [w1581 _]
              tunnel: [w1579 w1709] -> w1554
              tunnel: w1545 -> [w1578 _]
              frame False {
                n722 = for {
                  tunnel: w1580 -> [w1596] mode=indexing
                  tunnel: w1581 -> [w1584]
                  tunnel: w1580 -> [w1594] mode=indexing
                  tunnel: [w1585] -> w1579 mode=indexing if=w1582
                  tunnel: w1578 -> [w1583]
                  n723 = Unbundle By Name(w1596) -> ("x"=w1589:sgl, "y"=w1588:sgl, "orientation"=w1590:sgl, "robot_id"=w1595:u32, "Valid"=w1582:bool)
                  n724 = case shown="1" w1595 {
                    tunnel: w1589 -> [w1603 w1610 w1617 w1624 w1631 w1638 w1645 w1652 w1659 w1666 w1673 w1680 w1687 w1694 w1701 w1708]
                    tunnel: w1588 -> [w1601 w1608 w1615 w1622 w1629 w1636 w1643 w1650 w1657 w1664 w1671 w1678 w1685 w1692 w1699 w1706]
                    tunnel: w1590 -> [w1600 w1607 w1614 w1621 w1628 w1635 w1642 w1649 w1656 w1663 w1670 w1677 w1684 w1691 w1698 w1705]
                    tunnel: [w1599 w1606 w1613 w1620 w1627 w1634 w1641 w1648 w1655 w1662 w1669 w1676 w1683 w1690 w1697 w1704] -> w1593
                    tunnel: [w1598 w1605 w1612 w1619 w1626 w1633 w1640 w1647 w1654 w1661 w1668 w1675 w1682 w1689 w1696 w1703] -> w1592
                    tunnel: [w1597 w1604 w1611 w1618 w1625 w1632 w1639 w1646 w1653 w1660 w1667 w1674 w1681 w1688 w1695 w1702] -> w1591
                    tunnel: w1584 -> [_ _ _ _ _ _ _ _ _ _ _ _ _ _ _ _]
                    tunnel: w1583 -> [w1602 w1609 w1616 w1623 w1630 w1637 w1644 w1651 w1658 w1665 w1672 w1679 w1686 w1693 w1700 w1707]
                    frame 0, Default {
                      n725 = call "2ndOrderDerivate.vi"("t_capture"=w1602, "initial condition"=w1603, "x"=w1603) -> ("dx/dt"=w1599:dbl)  [unwired: 5 in, 3 out]
                      n726 = call "2ndOrderDerivate.vi"("t_capture"=w1602, "initial condition"=w1601, "x"=w1601) -> ("dx/dt"=w1598:dbl)  [unwired: 5 in, 3 out]
                      n727 = call "2ndOrderDerivate.vi"("t_capture"=w1602, "initial condition"=w1600, "x"=w1600) -> ("dx/dt"=w1597:dbl)  [unwired: 5 in, 3 out]
                    }
                    frame 1 {
                      n728 = call "2ndOrderDerivate.vi"("t_capture"=w1609, "initial condition"=w1610, "x"=w1610) -> ("dx/dt"=w1606:dbl)  [unwired: 5 in, 3 out]
                      n729 = call "2ndOrderDerivate.vi"("t_capture"=w1609, "initial condition"=w1608, "x"=w1608) -> ("dx/dt"=w1605:dbl)  [unwired: 5 in, 3 out]
                      n730 = call "2ndOrderDerivate.vi"("t_capture"=w1609, "initial condition"=w1607, "x"=w1607) -> ("dx/dt"=w1604:dbl)  [unwired: 5 in, 3 out]
                    }
                    frame 2 {
                      n731 = call "2ndOrderDerivate.vi"("t_capture"=w1616, "initial condition"=w1617, "x"=w1617) -> ("dx/dt"=w1613:dbl)  [unwired: 5 in, 3 out]
                      n732 = call "2ndOrderDerivate.vi"("t_capture"=w1616, "initial condition"=w1615, "x"=w1615) -> ("dx/dt"=w1612:dbl)  [unwired: 5 in, 3 out]
                      n733 = call "2ndOrderDerivate.vi"("t_capture"=w1616, "initial condition"=w1614, "x"=w1614) -> ("dx/dt"=w1611:dbl)  [unwired: 5 in, 3 out]
                    }
                    frame 3 {
                      n734 = call "2ndOrderDerivate.vi"("t_capture"=w1623, "initial condition"=w1624, "x"=w1624) -> ("dx/dt"=w1620:dbl)  [unwired: 5 in, 3 out]
                      n735 = call "2ndOrderDerivate.vi"("t_capture"=w1623, "initial condition"=w1622, "x"=w1622) -> ("dx/dt"=w1619:dbl)  [unwired: 5 in, 3 out]
                      n736 = call "2ndOrderDerivate.vi"("t_capture"=w1623, "initial condition"=w1621, "x"=w1621) -> ("dx/dt"=w1618:dbl)  [unwired: 5 in, 3 out]
                    }
                    frame 4 {
                      n737 = call "2ndOrderDerivate.vi"("t_capture"=w1630, "initial condition"=w1631, "x"=w1631) -> ("dx/dt"=w1627:dbl)  [unwired: 5 in, 3 out]
                      n738 = call "2ndOrderDerivate.vi"("t_capture"=w1630, "initial condition"=w1629, "x"=w1629) -> ("dx/dt"=w1626:dbl)  [unwired: 5 in, 3 out]
                      n739 = call "2ndOrderDerivate.vi"("t_capture"=w1630, "initial condition"=w1628, "x"=w1628) -> ("dx/dt"=w1625:dbl)  [unwired: 5 in, 3 out]
                    }
                    frame 5 {
                      n740 = call "2ndOrderDerivate.vi"("t_capture"=w1637, "initial condition"=w1638, "x"=w1638) -> ("dx/dt"=w1634:dbl)  [unwired: 5 in, 3 out]
                      n741 = call "2ndOrderDerivate.vi"("t_capture"=w1637, "initial condition"=w1636, "x"=w1636) -> ("dx/dt"=w1633:dbl)  [unwired: 5 in, 3 out]
                      n742 = call "2ndOrderDerivate.vi"("t_capture"=w1637, "initial condition"=w1635, "x"=w1635) -> ("dx/dt"=w1632:dbl)  [unwired: 5 in, 3 out]
                    }
                    frame 6 {
                      n743 = call "2ndOrderDerivate.vi"("t_capture"=w1644, "initial condition"=w1645, "x"=w1645) -> ("dx/dt"=w1641:dbl)  [unwired: 5 in, 3 out]
                      n744 = call "2ndOrderDerivate.vi"("t_capture"=w1644, "initial condition"=w1643, "x"=w1643) -> ("dx/dt"=w1640:dbl)  [unwired: 5 in, 3 out]
                      n745 = call "2ndOrderDerivate.vi"("t_capture"=w1644, "initial condition"=w1642, "x"=w1642) -> ("dx/dt"=w1639:dbl)  [unwired: 5 in, 3 out]
                    }
                    frame 7 {
                      n746 = call "2ndOrderDerivate.vi"("t_capture"=w1651, "initial condition"=w1652, "x"=w1652) -> ("dx/dt"=w1648:dbl)  [unwired: 5 in, 3 out]
                      n747 = call "2ndOrderDerivate.vi"("t_capture"=w1651, "initial condition"=w1650, "x"=w1650) -> ("dx/dt"=w1647:dbl)  [unwired: 5 in, 3 out]
                      n748 = call "2ndOrderDerivate.vi"("t_capture"=w1651, "initial condition"=w1649, "x"=w1649) -> ("dx/dt"=w1646:dbl)  [unwired: 5 in, 3 out]
                    }
                    frame 8 {
                      n749 = call "2ndOrderDerivate.vi"("t_capture"=w1658, "initial condition"=w1659, "x"=w1659) -> ("dx/dt"=w1655:dbl)  [unwired: 5 in, 3 out]
                      n750 = call "2ndOrderDerivate.vi"("t_capture"=w1658, "initial condition"=w1657, "x"=w1657) -> ("dx/dt"=w1654:dbl)  [unwired: 5 in, 3 out]
                      n751 = call "2ndOrderDerivate.vi"("t_capture"=w1658, "initial condition"=w1656, "x"=w1656) -> ("dx/dt"=w1653:dbl)  [unwired: 5 in, 3 out]
                    }
                    frame 9 {
                      n752 = call "2ndOrderDerivate.vi"("t_capture"=w1665, "initial condition"=w1666, "x"=w1666) -> ("dx/dt"=w1662:dbl)  [unwired: 5 in, 3 out]
                      n753 = call "2ndOrderDerivate.vi"("t_capture"=w1665, "initial condition"=w1664, "x"=w1664) -> ("dx/dt"=w1661:dbl)  [unwired: 5 in, 3 out]
                      n754 = call "2ndOrderDerivate.vi"("t_capture"=w1665, "initial condition"=w1663, "x"=w1663) -> ("dx/dt"=w1660:dbl)  [unwired: 5 in, 3 out]
                    }
                    frame 10 {
                      n755 = call "2ndOrderDerivate.vi"("t_capture"=w1672, "initial condition"=w1673, "x"=w1673) -> ("dx/dt"=w1669:dbl)  [unwired: 5 in, 3 out]
                      n756 = call "2ndOrderDerivate.vi"("t_capture"=w1672, "initial condition"=w1671, "x"=w1671) -> ("dx/dt"=w1668:dbl)  [unwired: 5 in, 3 out]
                      n757 = call "2ndOrderDerivate.vi"("t_capture"=w1672, "initial condition"=w1670, "x"=w1670) -> ("dx/dt"=w1667:dbl)  [unwired: 5 in, 3 out]
                    }
                    frame 11 {
                      n758 = call "2ndOrderDerivate.vi"("t_capture"=w1679, "initial condition"=w1680, "x"=w1680) -> ("dx/dt"=w1676:dbl)  [unwired: 5 in, 3 out]
                      n759 = call "2ndOrderDerivate.vi"("t_capture"=w1679, "initial condition"=w1678, "x"=w1678) -> ("dx/dt"=w1675:dbl)  [unwired: 5 in, 3 out]
                      n760 = call "2ndOrderDerivate.vi"("t_capture"=w1679, "initial condition"=w1677, "x"=w1677) -> ("dx/dt"=w1674:dbl)  [unwired: 5 in, 3 out]
                    }
                    frame 12 {
                      n761 = call "2ndOrderDerivate.vi"("t_capture"=w1686, "initial condition"=w1687, "x"=w1687) -> ("dx/dt"=w1683:dbl)  [unwired: 5 in, 3 out]
                      n762 = call "2ndOrderDerivate.vi"("t_capture"=w1686, "initial condition"=w1685, "x"=w1685) -> ("dx/dt"=w1682:dbl)  [unwired: 5 in, 3 out]
                      n763 = call "2ndOrderDerivate.vi"("t_capture"=w1686, "initial condition"=w1684, "x"=w1684) -> ("dx/dt"=w1681:dbl)  [unwired: 5 in, 3 out]
                    }
                    frame 13 {
                      n764 = call "2ndOrderDerivate.vi"("t_capture"=w1693, "initial condition"=w1694, "x"=w1694) -> ("dx/dt"=w1690:dbl)  [unwired: 5 in, 3 out]
                      n765 = call "2ndOrderDerivate.vi"("t_capture"=w1693, "initial condition"=w1692, "x"=w1692) -> ("dx/dt"=w1689:dbl)  [unwired: 5 in, 3 out]
                      n766 = call "2ndOrderDerivate.vi"("t_capture"=w1693, "initial condition"=w1691, "x"=w1691) -> ("dx/dt"=w1688:dbl)  [unwired: 5 in, 3 out]
                    }
                    frame 14 {
                      n767 = call "2ndOrderDerivate.vi"("t_capture"=w1700, "initial condition"=w1701, "x"=w1701) -> ("dx/dt"=w1697:dbl)  [unwired: 5 in, 3 out]
                      n768 = call "2ndOrderDerivate.vi"("t_capture"=w1700, "initial condition"=w1699, "x"=w1699) -> ("dx/dt"=w1696:dbl)  [unwired: 5 in, 3 out]
                      n769 = call "2ndOrderDerivate.vi"("t_capture"=w1700, "initial condition"=w1698, "x"=w1698) -> ("dx/dt"=w1695:dbl)  [unwired: 5 in, 3 out]
                    }
                    frame 15 {
                      n770 = call "2ndOrderDerivate.vi"("t_capture"=w1707, "initial condition"=w1708, "x"=w1708) -> ("dx/dt"=w1704:dbl)  [unwired: 5 in, 3 out]
                      n771 = call "2ndOrderDerivate.vi"("t_capture"=w1707, "initial condition"=w1706, "x"=w1706) -> ("dx/dt"=w1703:dbl)  [unwired: 5 in, 3 out]
                      n772 = call "2ndOrderDerivate.vi"("t_capture"=w1707, "initial condition"=w1705, "x"=w1705) -> ("dx/dt"=w1702:dbl)  [unwired: 5 in, 3 out]
                    }
                  }
                  n773 = Build Array(w1589, w1593, w1588, w1592, w1590, w1591) -> (w1587:dbl[])
                  n774 = call-poly <vilib>:"Array To Matrix.vi"("Real 1D Array"=w1587) -> ("Real Matrix (Column Vector)"=w1586:T3)
                  n775 = Bundle By Name(cluster=w1594, "x_k|k"=w1586) -> (w1585:T2)
                }
              }
              frame True {
              }
            }
            n776 = Bundle By Name(cluster=w1550, "robots_blue"=w1555, "robots_yellow"=w1554, "balls"=w1546) -> (w1553:T1)
            n777 = Bundle By Name(cluster=w1550, "New"=FALSE) -> (w1551:T1)
          }
        }
      }
      frame "Nenhum" {
      }
    }
  }
  n778 = feedback-in #1(w18) -> ()
  n779 = feedback-in #3(w4) -> ()
  n780 = disable-structure shown="Enabled" {
    disable-tunnel: _ -> [w1853 _]
    disable-tunnel: _ -> [w1852 _]
    disable-tunnel: _ -> [w1851 _]
    disable-tunnel: _ -> [w1846 _]
    disable-tunnel: w4 -> [w1843 w1858]
    disable-tunnel: [_ w1857] -> w3
    disable-tunnel: "cameras array" -> [_ w1856]
    disable-tunnel: "grSim?" -> [_ w1855]
    disable-tunnel: "Field Size" -> [_ w1854]
    frame Disabled {
      n781 = Bundle By Name(cluster=w1853, "robots_yellow"=w1852, "robots_blue"=w1851, "balls"=w1846) -> (w1842:cluster{})
      n782 = Unbundle By Name(w1842) -> ("balls"=w1845, "robots_yellow"=w1848, "robots_blue"=w1850)
      n783 = call "Select Robots By Confidence.vi"("robots_blue"=w1848) -> ("Array"=w1847:T2[])  [unwired: 10 in]
      n784 = call "Select Ball By Confidence.vi"("Array"=w1843, "balls"=w1845) -> ("balls out"=w1844:T4[])  [unwired: 9 in]
      n785 = call "Select Robots By Confidence.vi"("robots_blue"=w1850) -> ("Array"=w1849:T2[])  [unwired: 10 in]
      n786 = Bundle By Name(cluster=w1842, "balls"=w1844, "robots_yellow"=w1847, "robots_blue"=w1849) -> (w1841:cluster{})
    }
    frame Enabled {
      n787 = call "mediaIntesecaoCameras_v2.vi"("grsim?"=w1855, "cameras array"=w1856, "Field Geometry In"=w1854, "Cameras Array"=w1858) -> ("frame out"=w1857:T1)  [unwired: 7 in]
    }
  }
  n788 = Unbundle By Name(w3) -> ("balls"=w9:T4[])
  n789 = feedback-in #2(w9) -> ()
  n790 = Get Date/Time In Seconds() -> (seconds since 1Jan1904=w2:timestamp)
  n791 = Bundle By Name(cluster=w3, "Time Stamp"=w2) -> (→"Detection Frame Out":T1)
  "Field Size Out" <- "Field Size"
